vi "COD主界面（列队使用）.vi"() -> (8 "多列列表框":i32(listbox))   [LabVIEW 2016, in "斯坦道CODMn.lvlib"]
uses:
  <vilib>/Analysis/6fits.llb/Curve Fitting Criteria.ctl
  <vilib>/Utility/miscctls.llb/LVPointTypeDef.ctl
  <vilib>/Utility/config.llb/Read Key (I32).vi
  <vilib>/Utility/config.llb/Read Key (Double).vi
  <vilib>/Utility/config.llb/Read Key (Boolean).vi
  <vilib>/Utility/config.llb/Write Key (I32).vi
  <vilib>/Utility/config.llb/Read Key (String).vi
  <vilib>/Utility/config.llb/Write Key (Double).vi
  <vilib>/Utility/config.llb/Write Key (Boolean).vi
  <vilib>/Utility/config.llb/Write Key (String).vi
  <vilib>/Waveform/WDTFileIO.llb/Read Waveform from File.vi
  <vilib>/ptbypt/NI_PtbyPt.lvlib
  <vilib>/Utility/config.llb/NI_LVConfig.lvlib
  <vilib>/Analysis/NI_AALPro.lvlib
panel:
  in  "方程系数 2":cluster{"K":dbl, "b":dbl, "X^2":dbl} {"X^2" format="%#.6g"; "b" format="%#.6g"; "K" format="%#.6g"}
  out "r^2 2":dbl caption="r^2" format="%.8g"
  out "拟合公式 2":string
  in  "跨度值":dbl
  in  "公式切换阈值滴定数(0-9999)":u16
  out "公式系数":dbl[](array[numeric])
  in  "存校准信息":bool
  out "标液校准时间4":timestamp format="%<%Y/%m/%d %H:%M:%S>T"
  out "标液校准时间3":timestamp format="%<%Y/%m/%d %H:%M:%S>T"
  out "标液校准时间2":timestamp format="%<%Y/%m/%d %H:%M:%S>T"
  out "标液校准时间1":timestamp format="%<%Y/%m/%d %H:%M:%S>T"
  out "零点校准时间":timestamp format="%<%Y/%m/%d %H:%M:%S>T"
  in  "远程标样校准":enum16{"标液1", "标液2", "标液3", "标液4"}(ring)
  in  "远程校准量程":enum16{"低量程", "高量程"}(ring)
  in  "温度曲线":bool
  out "温度波形时间":timestamp
  in  "历史波形 2":bool
  out "时间-温度":u16[](array[numeric]) caption="数组"
  in  "关闭 4":bool
  out "时间温度曲线":u16[](graph)
  in  "加标回收量程：":enum32{"H", "L", "AUTO"}(ring)=enum."AUTO"
  in  "定时设置":cluster{"启动":bool, "控制命令":T1, "测量参数":T2}(xcontrol)
  out "氢氧化钠":dbl
  in  "序列号变更":bool
  out "模块版本号":string
  in  "更新程序":bool
  out "进样无液体告警":bool
  out "校准内容显示":string
  out "60分钟超时报警":bool
  in  "仪器参数":bool
  out "CODMn序列号":string
  out "CODMn软件版本：":string
  in  "标样核查量程选择":enum32{"H", "L", "AUTO"}(ring)=enum."AUTO"
  in  "标样浓度":dbl
  in  "零点核查量程选择":enum32{"H", "L", "AUTO"}(ring)=enum."AUTO"
  in  "零点核查浓度":dbl
  out "序列号":string
  in  "采水泵排液时间/s:":i32
  in  "采水泵润洗时间/s:":i32
  in  "采水泵沉淀时间/s:":i32
  in  "采水泵进样时间/s:":i32
  in  "常规版/认证版":enum16{"常规版-酸性", "常规版-碱性", "认证版", "浮台版"}(ring)
  in  "释放串口":bool
  in  "打开串口":bool
  in  "保存参数":dbl[](array[numeric])
  out "报警数字":i16
  out "CODMn工作状态":T3(ring)
  out "ORP-K":string
  out "ORP-B":string
  out "ORP-A":string
  out "x = y?":bool
  out "稀释倍数解释":string
  in  "跨度量程选择":enum32{"H", "L", "AUTO"}(ring)=enum."AUTO"
  in  "跨度液浓度":dbl
  in  "水样：":dbl
  in  "蒸馏水：":dbl
  in  "标液：":dbl
  in  "零点核查样：":dbl
  in  "加标回收样：":dbl
  in  "草酸钠":dbl
  in  "高锰酸钾":dbl
  in  "硫酸":dbl
  out "量程解释说明":string
  in  "高切低阈值:":dbl
  in  "低切高阈值:":dbl
  in  "水样量程选择:":enum16{"L", "H", "自动切换测一次", "自动切换测两次"}(ring)
  in  "氢氧化钠：":dbl
  in  "标准液浓度":dbl
  in  "温度":dbl
  in  "恒温时间":dbl
  in  "当前量程：":enum16{"L", "H"}(ring)
  in  "CODMn零点核查选择":enum16{"零点核查走纯水管", "零点核查走零漂管"}(ring)
  in  "锁定按钮":bool
  in  "低量程稀释倍数:":i8=1
  in  "高量程稀释倍数:":i8=2
  out "基本量程(显示)":string
  out "测量模式(显示)":string
  out "数据时间":string
  out "断电排液标记":bool
  out "COM":string
  in  "启用5":bool
  in  "校准5":bool
  in  "泵滴定数5":dbl
  in  "浓度5":dbl
  in  "启用4":bool
  in  "校准4":bool
  in  "泵滴定数4":dbl
  in  "浓度4":dbl
  out "波形时间":timestamp
  in  "历史波形":bool
  out "滴定数-ORP值":u16[](array[numeric]) caption="数组"
  in  "关闭 3":bool
  in  "滴定曲线":bool
  out "ORP滴定曲线":u16[](graph)
  out "空白测试标记":bool
  out "跨度核查标记":bool
  in  "量程选择":enum16{"低量程", "高量程"}(ring)
  in  "手动控制":bool
  in  "选用水样":enum16{"葡萄糖", "草酸钠"}(ring)
  in  "方程系数":cluster{"K":dbl, "b":dbl, "X^2":dbl} {"X^2" format="%#.6g"; "b" format="%#.6g"; "K" format="%#.6g"}
  out "XY图":cluster{"X Values":dbl[], "Y Values":dbl[]}[](graph)
  in  "模型":enum32{"线性", "多项式", "折线"}(ring)
  out "启动时间":timestamp format="%<%Y/%m/%d %H:%M:%S>T"
  in  "关闭 2":bool
  out "r^2":dbl format="%.8g"
  out "拟合公式":string
  in  "启用3":bool
  in  "启用2":bool
  in  "启用1":bool
  in  "校准3":bool
  in  "校准2":bool
  in  "校准1":bool
  in  "泵滴定数3":dbl
  in  "泵滴定数2":dbl
  in  "泵滴定数1":dbl
  in  "浓度3":dbl
  in  "浓度2":dbl
  in  "浓度1":dbl
  in  "写入":bool
  out "零点核查标记":bool
  out "排液故障":bool
  out "进水样超量程":bool
  out "标样核查标记":bool
  out "平行样测量":bool
  out "加标回收测量":bool
  out "质控样测量":bool
  out "待机":bool
  out "校标错误":bool
  out "校零错误":bool
  out "测量错误":bool
  out "草酸钠报警":bool
  out "高锰酸钾报警":bool
  out "加热故障":bool
  out "温控器故障":bool
  out "ORP故障":bool
  out "排液标记":bool
  out "故障标记":bool
  out "校标标记":bool
  out "校零标记":bool
  out "通讯状态":bool
  out "水样测量":bool
  in  "读取":bool
  in  "返回":bool
  in  "校准配置":bool
  in  "零点泵计量数 2":dbl
  in  "标度泵计量数 2":dbl
  out "标度滴定值":dbl
  out "零点滴定值":dbl
  in  "保存":bool
  in  "关闭":bool
  out "仪器时间":timestamp format="%<%Y/%m/%d %H:%M:%S>T"
  out "秒":u16
  out "分":u16
  out "COD浓度（mg/L)":dbl format="%.2g"
  out "进样管":dbl
  out "高锰酸钾":dbl
  out "草酸钠":dbl
  out "硫酸":dbl
  out "实时ORP":dbl
  out "温度℃":dbl
  out "加热":bool
  out "搅拌":bool
  out "进硫酸":bool
  out "进加标回收样":bool
  out "进零点核查样":bool
  out "进标液":bool
  out "进蒸馏水":bool
  out "进水样":bool
  out "进草酸钠":bool
  out "进高锰酸钾":bool
  in  "启动":bool
  in  "故障清除":bool
  in  "参数配置":bool
  in  "停止":bool
  in  "单步启动":bool
  out "系统时间":timestamp
  in  "时间校准":bool
  out "模式（受控）":u16
  # "测试时长："
  # "注：遇到加热故障和排液故障时仪器不能正常启动，\n必须排查故障并点击报警清除按钮方可运行。"
  # "mg/L"
  # "基本参数设置"
  # "校零校标结果"
  # "泵计量参数设置"
  # "校零结果："
  # "校零滴定值："
  # "高锰酸钾："
  # "加热恒温温度(℃):"
  # "草酸钠："
  # "校标结果："
  # "标度滴定值："
  # "恒温时间(分钟):"
  # "零点泵计量值："
  # "硫酸："
  # "标准液浓度(mg/L):"
  # "标度泵计量值："
  # "跨度核查浓度："
  # "跨度核查量程："
  # "零点核查浓度："
  # "标样浓度："
  # "零点核查量程："
  # "标样核查量程："
  # "跨度值:"
  # "校准配置界面"
  # "测量信号值"
  # "启用"
  # "校准时间"
  # "浓度"
  # "零点"
  # "标液1"
  # "标液2"
  # "标液3"
  # "标液4"
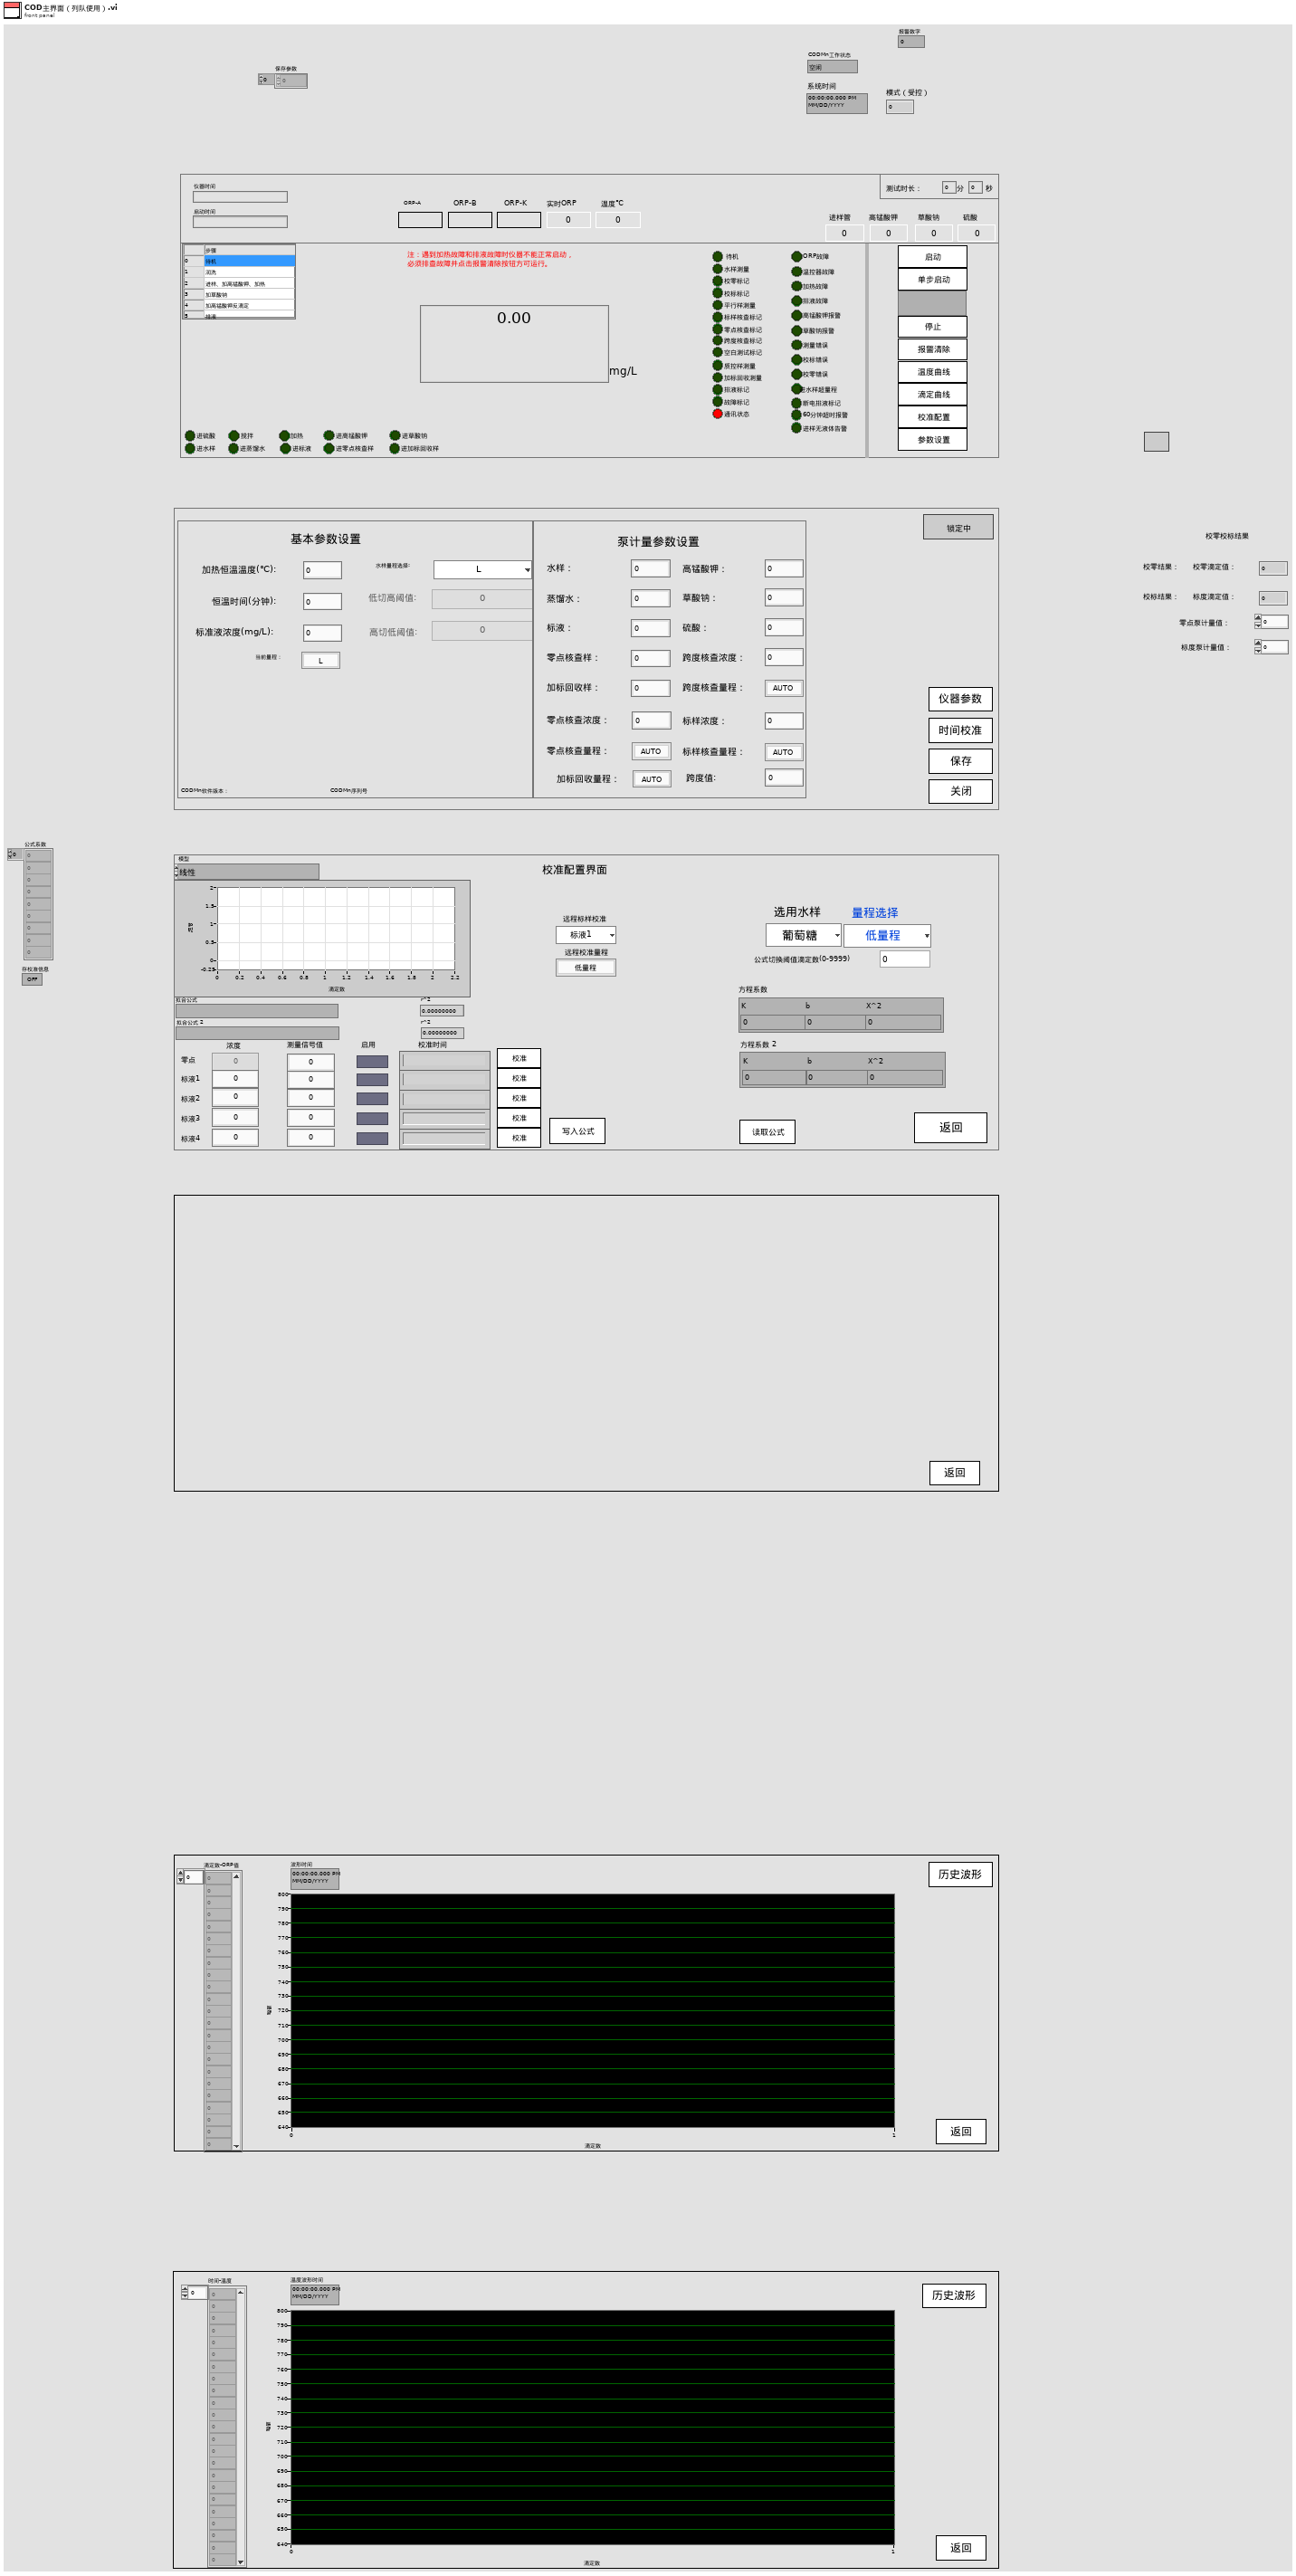
[diagram p1: front panel]
types:
  T1 = typedef "定时设置.xctl/国标控制命令.ctl" = enum16{"启动测量", "标样核查", "零点核查", "跨度核查", "空白测试", "平行样测试", "加标回收", "空白校准", "标样校准", "初始化（清洗）", "停止测试", "仪器重启", "校时", "模式设置", "测量间隔设置"}
  T2 = typedef "定时设置.xctl/测量参数.ctl" = u16
  T3 = enum16{"空闲", "水样测试", "标样核查", "零点核查", "跨度核查", "空白测试", "平行样测试", "质控样", "空白校准", "标样校准", "加标回收"}
  T4 = typedef "LVPointTypeDef.ctl" = cluster{"Horizontal":i16, "Vertical":i16}
  T5 = cluster{"Major":u16, "Minor":u16, "Fix":u16, "Build":u16}
  T6 = typedef "NI_LVConfig.lvlib/Config Data RefNum.ctl" = refnum<k1>
  T7 = cluster{"时间源选择":enum16{"系统时间源", "仪器时间源"}, "外部时间源":timestamp}
  T8 = enum32{"Bad", "Idle", "Run top level", "Running"}
  T9 = enum8{"Enabled", "Disabled", "Disabled and Grayed Out"}
  T10 = cluster{"时间":timestamp, "测量模式":string, "数据类型":string, "检测值":sgl, "单位":string, "数据标识":string, "因子编码":string, "标样参考值":sgl, "ORP-A":sgl, "ORP-B":sgl, "ORP-K":sgl, "COD滴定值":sgl, "高锰酸钾滴定数":sgl, "温度":sgl, "量程":sgl, "LastTime":timestamp, "序列号:":string, "跨度值":sgl}
  T11 = cluster{"因子编码":u32, "单位":u16, "标样参考值":sgl, "水样数据时间":timestamp, "水样实测值":sgl, "水样数据标识":string, "标样数据时间":timestamp, "标样实测值":sgl, "标样数据标识":string, "空白数据时间":timestamp, "空白实测值":sgl, "空白数据标识":string, "零点核查数据时间":timestamp, "零点核查实测值":sgl, "零点核查数据标识":string, "跨度核查数据时间":timestamp, "跨度核查实测值":sgl, "跨度核查数据标识":string, "加标回收数据时间":timestamp, "加标回收实测值":sgl, "加标回收数据标识":string, "平行样数据时间":timestamp, "平行样实测值":sgl, "平行样数据标识":string}
  T12 = cluster{"测量量程":dbl, "测量精度":dbl, "测量间隔":dbl, "消解温度":dbl, "消解时长":dbl, "空白校准时间":timestamp, "曲线截距":dbl, "曲线斜率":dbl, "测量检出限":dbl, "测量信号值":dbl, "线性相关系数":dbl, "二次多项式系数":dbl, "标样校准时间":timestamp, "稀释倍数":dbl, "三项式系数":dbl, "空白标定系数":dbl, "量程系数":dbl, "F0/ORPA":dbl, "F1/ORPB":dbl, "F2/ORPK":dbl, "F3":dbl, "F4":dbl, "F5":dbl, "F6":dbl, "F7":dbl, "X0/滴定数":dbl, "量程":dbl}
  T13 = cluster{"运行模式":enum16{"维护模式", "常规模式", "应急模式", "质控模式"}, "质控频次":enum16{"关闭", "每天", "星期一", "星期二", "星期三", "星期四", "星期五", "星期六", "星期日"}, "空白核查时间":u16, "跨度核查时间":u16, "24H周期设置":bool[]}
  T14 = cluster{"数组 2[0]":sgl, "数组 2[1]":sgl, "数组 2[2]":sgl, "数组 2[3]":sgl, "数组 2[4]":sgl, "数组 2[5]":sgl, "数组 2[6]":sgl, "数组 2[7]":sgl, "数组 2[8]":sgl, "数组 2[9]":sgl, "数组 2[10]":sgl, "数组 2[11]":sgl, "数组 2[12]":sgl, "数组 2[13]":sgl, "数组 2[14]":sgl, "数组 2[15]":sgl, "数组 2[16]":sgl, "数组 2[17]":sgl, "数组 2[18]":sgl, "数组 2[19]":sgl, "数组 2[20]":sgl, "数组 2[21]":sgl, "数组 2[22]":sgl, "数组 2[23]":sgl, "数组 2[24]":sgl, "数组 2[25]":sgl, "数组 2[26]":sgl, "数组 2[27]":sgl, "数组 2[28]":sgl, "数组 2[29]":sgl, "数组 2[30]":sgl, "数组 2[31]":sgl, "数组 2[32]":sgl, "数组 2[33]":sgl, "数组 2[34]":sgl, "数组 2[35]":sgl, "数组 2[36]":sgl, "数组 2[37]":sgl, "数组 2[38]":sgl, "数组 2[39]":sgl, "数组 2[40]":sgl, "数组 2[41]":sgl}
  T15 = typedef "NI_AALPro.lvlib/Curve Fitting Criteria.ctl" = u16
  T16 = cluster{"ORP故障":bool, "温控器故障":bool, "加热故障":bool, "高锰酸钾报警":bool, "草酸钠报警":bool, "测量错误":bool, "校零错误":bool, "校标错误":bool, " 进水样超量程":bool, "排液阀故障":bool, "60分钟超时报警":bool, "进样无液体报警":bool}
  T17 = cluster{"时间标识":timestamp, "参数":string, "日志信息":string, "流程参数":string}
  T18 = cluster{"确定":bool, "测量量程":dbl, "测量精度":dbl, "测量间隔":dbl, "消解温度":dbl, "消解时长":dbl, "空白校准时间":timestamp, "曲线截距":dbl, "曲线斜率":dbl, "测量检出限":dbl, "测量信号值":dbl, "线性相关系数":dbl, "二次多项式系数":dbl, "标样校准时间":timestamp, "稀释倍数":dbl, "三项式系数":dbl, "空白标定系数":dbl, "量程系数":dbl, "F0/ORPA":dbl, "F1/ORPB":dbl, "F2/ORPK":dbl, "F3":dbl, "F4":dbl, "F5":dbl, "F6":dbl, "F7":dbl, "X0/滴定数":dbl, "量程":dbl}
  T19 = cluster{"时间标识":timestamp, "设备":string, "日志信息":string, "流程参数":string}
  T20 = cluster{"[0]":string, "[1]":string, "[2]":string}
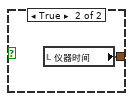
[diagram p3: hidden frame]
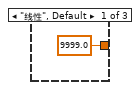
[diagram p9: hidden frame]
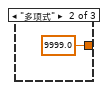
[diagram p10: hidden frame]
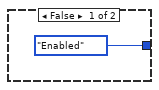
[diagram p11: hidden frame]
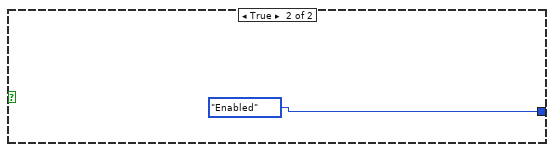
[diagram p12: hidden frame]
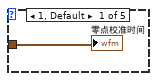
[diagram p17: hidden frame]
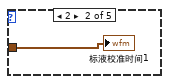
[diagram p18: hidden frame]
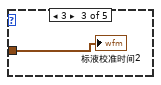
[diagram p19: hidden frame]
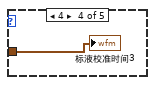
[diagram p20: hidden frame]
diagram:
  n1 = flat-sequence {
    tunnel: w3 -> [_]
    frame #0 {
      n2 = vi-ref "斯坦道CODMn.lvlib:待机状态数据存储写入和切换量程(子VI).vi"() -> (w64:refnum<vi>)
      n3 = vi-ref "斯坦道CODMn.lvlib:日志报警状态存储 (子VI).vi"() -> (w57:refnum<vi>)
      n4 = vi-ref "斯坦道CODMn.lvlib:高锰酸钾-ORP滴定曲线(子VI).vi"() -> (w44:refnum<vi>)
      n5 = property class="VI"(reference=w57, error in=errorcluster {"status"=FALSE, "code"=0, "source"=""} ("错误输出")) -> ("Name"=w56:string)  [unwired: 2 out]
      n6 = property class="VI"(reference=w44, error in=errorcluster {"status"=FALSE, "code"=0, "source"=""} ("错误输出")) -> ("Name"=w45:string)  [unwired: 2 out]
      n7 = property class="VI"(reference=w64, error in=errorcluster {"status"=FALSE, "code"=0, "source"=""} ("错误输出")) -> ("Name"=w63:string)  [unwired: 2 out]
      n8 = Open VI Reference(type specifier VI Refnum (for type only)=refnum<vi> refnum, vi path=w56, options=128 ("选项")) -> (vi reference=w40:refnum<vi>, error out=w54:errorcluster)  [unwired: 3 in]
      n9 = Open VI Reference(type specifier VI Refnum (for type only)=refnum<vi> refnum, vi path=w45, options=128 ("选项")) -> (vi reference=w43:refnum<vi>, error out=w47:errorcluster)  [unwired: 3 in]
      n10 = call-by-ref "?"(reference=w40, error in=w54) -> (reference out=w52:refnum<vi>, error out=w53:errorcluster)  [unwired: 12 in]
      n11 = call-by-ref "?"(reference=w43, error in=w47) -> (reference out=w49:refnum<vi>, error out=w48:errorcluster)  [unwired: 12 in]
      n12 = Open VI Reference(type specifier VI Refnum (for type only)=refnum<vi> refnum, vi path=w63, options=128 ("选项")) -> (vi reference=w38:refnum<vi>, error out=w61:errorcluster)  [unwired: 3 in]
      n13 = Close Reference(reference=w52, error in (no error)=w53) -> ()  [unwired: 1 out]
      n14 = call-by-ref "?"(reference=w38, error in=w61) -> (reference out=w59:refnum<vi>, error out=w60:errorcluster)  [unwired: 12 in]
      n15 = Close Reference(reference=w49, error in (no error)=w48) -> ()  [unwired: 1 out]
      n16 = Close Reference(reference=w59, error in (no error)=w60) -> ()  [unwired: 1 out]
      n17 = vi-ref "斯坦道CODMn.lvlib:时间-温度曲线(子VI).vi"() -> (w26:refnum<vi>)
      n18 = vi-ref "斯坦道CODMn.lvlib:关键参数交互.vi"() -> (w35:refnum<vi>)
      n19 = property class="VI"(reference=w35, error in=errorcluster {"status"=FALSE, "code"=0, "source"=""} ("错误输出")) -> ("Name"=w34:string)  [unwired: 2 out]
      n20 = property class="VI"(reference=w26, error in=errorcluster {"status"=FALSE, "code"=0, "source"=""} ("错误输出")) -> ("Name"=w25:string)  [unwired: 2 out]
      n21 = Open VI Reference(type specifier VI Refnum (for type only)=refnum<vi> refnum, vi path=w34, options=128 ("选项")) -> (vi reference=w36:refnum<vi>, error out=w32:errorcluster)  [unwired: 3 in]
      n22 = call-by-ref "?"(reference=w36, error in=w32, "量程选择"=enum16{"低量程", "高量程"}."低量程", "模型"=enum32{"线性", "多项式", "折线"}."线性") -> (reference out=w30:refnum<vi>, error out=w31:errorcluster)  [unwired: 10 in]
      n23 = Open VI Reference(type specifier VI Refnum (for type only)=refnum<vi> refnum, vi path=w25, options=128 ("选项")) -> (vi reference=w27:refnum<vi>, error out=w23:errorcluster)  [unwired: 3 in]
      n24 = call-by-ref "?"(reference=w27, error in=w23) -> (reference out=w21:refnum<vi>, error out=w22:errorcluster)  [unwired: 12 in]
      n25 = Close Reference(reference=w30, error in (no error)=w31) -> ()  [unwired: 1 out]
      n26 = Close Reference(reference=w21, error in (no error)=w22) -> ()  [unwired: 1 out]
    }
  }
  n27 = property on="定时设置" class="定时设置 (严格)"("引用参数"="CODMn") -> (error out=w1:errorcluster)  [unwired: 2 in, 1 out]
  n28 = flat-sequence {
    tunnel: [w68] -> w5
    tunnel: [errorcluster {"status"=FALSE, "code"=0, "source"=""} ("错误输出")] -> w3
    tunnel: [w70] -> w4
    frame #0 {
      w92 = "192.168.1.100" ("名称")
      n29 = global write "COD内部交互全局.vi" "量程切换次数"(u8 0 ("量程切换次数")) -> ()
      n30 = global write "COD内部交互全局.vi" "切换量程连续测两次"(FALSE ("切换量程连续测两次")) -> ()
      n31 = global read "COD内部交互全局.vi" "序列号:"() -> (w99:string)
      n32 = property on="窗格" class="Pane"("Origin"=T4 {"Horizontal"=0, "Vertical"=0} ("原点")) -> ()  [unwired: 2 in, 2 out]
      n33 = Empty String/Path?(string/path=w99) -> (empty?=w67:bool)
      n34 = case shown="真" w67 {
        tunnel: w99 -> [w113 _]
        tunnel: [w112 "data\\CODMnSet.ini" ("名称或相对路径")] -> w80
        frame False {
          # "与生产用上位机交互"
          n35 = Concatenate Strings("data\\" ("字符串"), "序列号" ("字符串"), w113, "Set.ini" ("名称或相对路径")) -> (w112:string)
        }
        frame True {
        }
      }
      n36 = String To IP(1:w92) -> (0:w85:u32)
      n37 = IP To String(2:w85) -> (0:w88:string)  [unwired: 1 in]
      n38 = Not Equal?(x=w92, y=w88) -> (x != y?=w93:bool)
      n39 = Concatenate Strings("\\\\" ("字符串"), w88) -> (w87:string)
      n40 = global write "CODMN外部API.vi" "ping"(w93) -> ()
      n41 = String To Path(string=w87) -> (path=w94:path)
      n42 = Build Path(base path=w94, name or relative path=w80) -> (appended path=w89:path)
      n43 = local write "量程选择"(enum16{"低量程", "高量程"}."低量程" ("量程选择")) -> ()
      n44 = local write "选用水样"(enum16{"葡萄糖", "草酸钠"}."葡萄糖" ("选用水样")) -> ()
      n45 = global write "COD内部交互全局.vi" "配置文件ini"(w80) -> ()
      n46 = case shown="真" w93 {
        tunnel: w89 -> [w103 w107]
        tunnel: [w103 w106] -> w90
        tunnel: [FALSE w105] -> w91
        frame False {
        }
        frame True {
          n47 = call <vilib>:"Check if File or Folder Exists.vi"("path"=w107) -> ("file or folder exists?"=w105:bool, "dup path"=w106:path)  [unwired: 8 in, 1 out]
        }
      }
      n48 = control-ref of="本VI"() -> (w79:refnum<vi>)
      n49 = case shown="假" w91 {
        tunnel: w90 -> [_ w111]
        tunnel: [w109 w111] -> w71
        tunnel: w80 -> [w108 _]
        frame False {
          # "本地文件地址"
          n50 = call <vilib>:"Application Directory.vi"() -> ("Application Directory"=w110:path)
          n51 = Build Path(base path=w110, name or relative path=w108) -> (appended path=w109:path)
        }
        frame True {
          # "网络共享地址"
        }
      }
      n52 = property class="VI"(reference=w79) -> ("Library.Version"=w78:T5)  [unwired: 1 in, 2 out]
      n53 = Unbundle By Name(w78) -> ("Major"=w76:u16, "Minor"=w75:u16, "Fix"=w74:u16, "Build"=w73:u16)
      n54 = Format Into String(format string="模块版本号：%d.%d.%d.%d" ("格式字符串"), w76, w75, w74, w73) -> (resulting string=→"模块版本号":string)  [unwired: 2 in, 1 out]
      n55 = global write "CODMN外部API.vi" "配置文件 path"(w71) -> ()
      n56 = call <vilib>:"Open Config Data.vi"("configuration file path"=w71) -> ("error out"=w81:errorcluster, "refnum"=w82:T6)  [unwired: 8 in, 1 out]
      n57 = vi-ref "斯坦道CODMn.lvlib:CODMn断电保存全局变量.vi"() -> (w95:refnum<vi>)
      n58 = call <userlib>:"Read Panel from INI__ogtk.vi"("error in (no error)"=w81, "VI ref"=w95, "refnum"=w82) -> ("error out"=w83:errorcluster, "refnum out"=w84:T6)  [unwired: 7 in]
      n59 = call <vilib>:"Close Config Data.vi"("error in (no error)"=w83, "refnum"=w84) -> ("error out"=w69:errorcluster)  [unwired: 8 in, 1 out]
      n60 = call <vilib>:"Clear Errors.vi"("error in (no error)"=w69) -> ("error out"=w66:errorcluster)  [unwired: 5 in, 1 out]
      n61 = Read from Text File(file (use dialog)=w71, error in=w66) -> (text=w70:string, error out=w68:errorcluster)  [unwired: 2 in, 2 out]
      "稀释倍数解释" <- "稀释倍数解释：\n稀释倍数选择1，表示不稀释\n默认低量程系数倍数1，高量程系数倍数2\n则低量程为0~8，高量程为0~16" ("稀释倍数解释")
    }
  }
  n62 = while {
    tunnel: w1 -> [_]
    stop <- FALSE stop-if-true
    n63 = Wait (ms)(milliseconds to wait=u32 500 ("等待时间（毫秒）")) -> ()  [unwired: 1 out]
    n64 = global read "COD测量模式全局.vi" "CODMn工作状态"() -> (w124:T3)
    n65 = local read "通讯状态"() -> (w118:bool)
    n66 = case shown="假" w118 {
      tunnel: [w134 w135] -> w122
      frame False {
        n67 = Get Date/Time In Seconds() -> (seconds since 1Jan1904=w134:timestamp)
      }
      frame True {
        n68 = local read "仪器时间"() -> (w135:timestamp)
      }
    }
    n69 = vi-ref "斯坦道CODMn.lvlib:CODMn测量流程.vi"() -> (w131:refnum<vi>)
    n70 = Bundle By Name(cluster=T7 {"时间源选择"=enum."系统时间源", "外部时间源"=timestamp(0 s since 1904-01-01)} ("时间源"), "时间源选择"=enum16{"系统时间源", "仪器时间源"}."仪器时间源", "外部时间源"=w122) -> (w120:T7)
    n71 = property class="VI"(reference=w131) -> ("Exec.State"=w129:T8, "Name"=w130:string)  [unwired: 1 in, 2 out]
    n72 = Not Equal?(x=w124, y=T3."空闲") -> (x != y?=w119:bool)
    n73 = property on="定时设置" class="定时设置 (严格)"("仪器状态"=w119, "时间源"=w120) -> ()  [unwired: 2 in, 2 out]
    n74 = Unbundle By Name("定时设置") -> ("启动"=w127:bool, "控制命令"=w128:T1)
    n75 = case shown="真" w127 {
      tunnel: w130 -> [_ w138]
      tunnel: w128 -> [_ w137]
      tunnel: w129 -> [_ w136]
      frame False {
      }
      frame True {
        n76 = case shown="\"Idle\"" w136 {
          tunnel: w138 -> [_ w142]
          tunnel: w137 -> [_ w139]
          frame "Bad", Default {
          }
          frame "Idle" {
            n77 = Open VI Reference(type specifier VI Refnum (for type only)=refnum<vi> refnum, vi path=w142, options=128 ("选项")) -> (vi reference=w143:refnum<vi>, error out=w144:errorcluster)  [unwired: 3 in]
            n78 = call-by-ref "开始异步调用"(reference=w143, error in=w144, "控制命令"=w139) -> (reference out=w145:refnum<vi>, error out=w146:errorcluster)  [unwired: 11 in]
            n79 = Close Reference(reference=w145, error in (no error)=w146) -> ()  [unwired: 1 out]
          }
        }
      }
    }
  }
  n80 = Obtain Queue(name (unnamed)="CODMn" ("名称（未命名）"), element data type=cluster{"命令":string} {"命令"="启用模块"} ("元素")) -> (queue out=w15:refnum<queue>, error out=w14:errorcluster)  [unwired: 3 in, 1 out]
  n81 = while {
    tunnel: [w153] -> _
    shift-right: [w151] -> _
    shift-left: w4 -> [w150]
    tunnel: w5 -> [_]
    stop <- FALSE stop-if-true
    n82 = global read "CODMN外部API.vi" "配置文件 path"() -> (w147:path)
    n83 = Wait (ms)(milliseconds to wait=u32 1000 ("等待时间（毫秒）")) -> ()  [unwired: 1 out]
    n84 = Read from Text File(file (use dialog)=w147) -> (text=w151:string, error out=w148:errorcluster)  [unwired: 3 in, 2 out]
    n85 = Not Equal?(x=w151, y=w150) -> (x != y?=w149:bool)
    n86 = case shown="真" w149 {
      tunnel: [w155 w162] -> w153
      tunnel: w147 -> [_ w156]
      tunnel: w148 -> [w155 _]
      frame False {
      }
      frame True {
        # "文件发生改变进行更新，远端和本地都更新"
        n87 = vi-ref "斯坦道CODMn.lvlib:CODMn断电保存全局变量.vi"() -> (w157:refnum<vi>)
        n88 = call <vilib>:"Open Config Data.vi"("configuration file path"=w156) -> ("error out"=w161:errorcluster, "refnum"=w160:T6)  [unwired: 8 in, 1 out]
        n89 = call <userlib>:"Read Panel from INI__ogtk.vi"("error in (no error)"=w161, "VI ref"=w157, "refnum"=w160) -> ("error out"=w159:errorcluster, "refnum out"=w158:T6)  [unwired: 7 in]
        n90 = call <vilib>:"Close Config Data.vi"("error in (no error)"=w159, "refnum"=w158) -> ("error out"=w162:errorcluster)  [unwired: 8 in, 1 out]
      }
    }
  }
  n91 = vi-ref "CODMn通讯.vi"() -> (w6:refnum<vi>)
  n92 = while {
    stop <- FALSE stop-if-true
    n93 = global read "COD内部交互全局.vi" "待机"() -> (w164:bool)
    n94 = Wait (ms)(milliseconds to wait=u32 1000 ("等待时间（毫秒）")) -> ()  [unwired: 1 out]
    n95 = case shown="假" w164 {
      tunnel: [w181 T9."Enabled" ("禁用")] -> w166
      tunnel: [w180 _] -> w165
      frame False {
        # "运行中"
        n96 = local read "校标标记"() -> (w179:bool)
        n97 = local read "校零标记"() -> (w178:bool)
        n98 = Or(x=w179, y=w178) -> (x .or. y?=w182:bool)
        n99 = case shown="真" w182 {
          tunnel: [T9."Enabled" ("禁用") T9."Disabled and Grayed Out" ("禁用")] -> w181
          tunnel: [_ TRUE] -> w180
          frame False {
          }
          frame True {
          }
        }
      }
      frame True {
      }
    }
    n100 = control-ref of="量程选择"() -> (w172:refnum<vi>)
    n101 = property on="校准内容显示" class="Str"("Visible"=w165) -> ()  [unwired: 2 in, 2 out]
    n102 = control-ref of="选用水样"() -> (w173:refnum<vi>)
    n103 = control-ref of="校准5"() -> (w167:refnum<vi>)
    n104 = control-ref of="校准4"() -> (w168:refnum<vi>)
    n105 = control-ref of="校准3"() -> (w169:refnum<vi>)
    n106 = control-ref of="校准2"() -> (w170:refnum<vi>)
    n107 = control-ref of="校准1"() -> (w171:refnum<vi>)
    n108 = Build Array(w167, w168, w169, w170, w171, w173, w172) -> (w174:refnum<vi>[])
    n109 = for {
      tunnel: w174 -> [w177] mode=indexing
      tunnel: w166 -> [w176]
      n110 = property class="Ctl"(reference=w177, "DisabledEnum"=w176) -> ()  [unwired: 1 in, 2 out]
    }
  }
  n111 = while {
    tunnel: w5 -> [_]
    stop <- FALSE stop-if-true
    # "赋值循环"
    n112 = flat-sequence {
      frame #0 {
        # "测量数据区"
        n113 = global read "COD内部交互全局.vi" "data"() -> (w326:T10)
        n114 = global read "COD测量模式全局.vi" "测量模式文字实时"() -> (w312:string)
        "测量模式(显示)" <- w312
        n115 = global read "CODMn断电保存全局变量.vi" "测量数据区"() -> (w321:T11)
        n116 = Unbundle By Name(w326) -> ("时间"=w325:timestamp, "检测值"=w324:sgl, "数据标识"=w323:string)
        n117 = case shown="\"水样测试\"" w312 {
          tunnel: w321 -> [w327 w332 w337 w342 w347 w352 w357 w362 w367 w372]
          tunnel: [w327 w331 w336 w338 w346 w351 w356 w361 w363 w371] -> w322
          tunnel: w325 -> [_ w330 w335 w341 w345 w350 w355 w360 w366 w370]
          tunnel: w324 -> [_ w329 w334 w340 w344 w349 w354 w359 w365 w369]
          tunnel: w323 -> [_ w328 w333 w339 w343 w348 w353 w358 w364 w368]
          frame "", Default {
          }
          frame "水样测试" {
            n118 = Bundle By Name(cluster=w332, "水样数据时间"=w330, "水样实测值"=w329, "水样数据标识"=w328) -> (w331:T11)
          }
          frame "标样核查" {
            n119 = Bundle By Name(cluster=w337, "标样数据时间"=w335, "标样实测值"=w334, "标样数据标识"=w333) -> (w336:T11)
          }
          frame "跨度核查" {
            n120 = Bundle By Name(cluster=w342, "跨度核查数据时间"=w341, "跨度核查实测值"=w340, "跨度核查数据标识"=w339) -> (w338:T11)
          }
          frame "零点核查" {
            n121 = Bundle By Name(cluster=w347, "零点核查数据时间"=w345, "零点核查实测值"=w344, "零点核查数据标识"=w343) -> (w346:T11)
          }
          frame "空白测试" {
            n122 = Bundle By Name(cluster=w352, "空白数据时间"=w350, "空白实测值"=w349, "空白数据标识"=w348) -> (w351:T11)
          }
          frame "加标回收" {
            n123 = Bundle By Name(cluster=w357, "加标回收数据时间"=w355, "加标回收实测值"=w354, "加标回收数据标识"=w353) -> (w356:T11)
          }
          frame "平行样" {
            n124 = Bundle By Name(cluster=w362, "平行样数据时间"=w360, "平行样实测值"=w359, "平行样数据标识"=w358) -> (w361:T11)
          }
          frame "校零" {
            n125 = Bundle By Name(cluster=w367, "空白数据时间"=w366, "空白实测值"=w365, "空白数据标识"=w364) -> (w363:T11)
          }
          frame "校标" {
            n126 = Bundle By Name(cluster=w372, "标样数据时间"=w370, "标样实测值"=w369, "标样数据标识"=w368) -> (w371:T11)
          }
        }
        n127 = Unbundle By Name(w321) -> ("水样实测值"=w318:sgl)
        n128 = feedback-in #1(w321) -> ()
        n129 = feedback #1(w321) -> (w320:T11)
        n130 = global read "CODMn断电保存全局变量.vi" "水样测试量程"() -> (w314:enum16{"L", "H"})
        n131 = Unbundle By Name(w320) -> ("水样实测值"=w319:sgl)
        n132 = feedback #2(w314) -> (w315:enum16{"L", "H"})
        n133 = feedback-in #2(w314) -> ()
        n134 = Not Equal?(x=w315, y=w314) -> (x != y?=w313:bool)
        n135 = Not Equal?(x=w318, y=w319) -> (x != y?=w317:bool)
        n136 = global write "CODMn断电保存全局变量.vi" "测量数据区"(w322) -> ()
        n137 = Or(x=w317, y=w313) -> (x .or. y?=w316:bool)
        n138 = case shown="真" w316 {
          frame False {
          }
          frame True {
            # "水样值发送改变存储本地"
            n139 = call "配置文件保存.vi"() -> ()  [unwired: 12 in]
          }
        }
      }
    }
    n140 = flat-sequence {
      frame #0 {
        # "局部变量给内部交互用全局变量"
        n141 = local read "COD浓度（mg/L)"() -> (w219:dbl)
        n142 = local read "CODMn工作状态"() -> (w222:T3)
        n143 = local read "多列列表框"() -> (w220:i32)
        n144 = local read "标准液浓度"() -> (w218:dbl)
        n145 = local read "温度℃"() -> (w213:dbl)
        n146 = local read "高锰酸钾报警"() -> (w216:bool)
        n147 = local read "断电排液标记"() -> (w215:bool)
        n148 = local read "实时ORP"() -> (w212:dbl)
        n149 = local read "故障标记"() -> (w221:bool)
        n150 = local read "高锰酸钾"() -> (w214:dbl)
        n151 = local read "待机"() -> (w217:bool)
        n152 = global write "COD内部交互全局.vi" "实时温度"(w213) -> ()
        n153 = global write "运行时序全局变量.vi" "多列列表框"(w220) -> ()
        n154 = global write "COD内部交互全局.vi" "故障标记"(w221) -> ()
        n155 = global write "COD内部交互全局.vi" "ORP显示"(w212) -> ()
        n156 = global write "COD浓度全局变量.vi" "标准液浓度"(w218) -> ()
        n157 = global write "COD内部交互全局.vi" "高锰酸钾"(w214) -> ()
        n158 = global write "COD内部交互全局.vi" "待机"(w217) -> ()
        n159 = global write "COD测量模式全局.vi" "CODMn工作状态"(w222) -> ()
        n160 = global write "COD内部交互全局.vi" "高锰酸钾报警"(w216) -> ()
        n161 = global write "COD内部交互全局.vi" "断电排液标记"(w215) -> ()
        n162 = global write "COD浓度全局变量.vi" "COD浓度（mg/L)"(w219) -> ()
      }
    }
    n163 = flat-sequence {
      frame #0 {
        # "断电保存全局给局部变量"
        n164 = global read "CODMn断电保存全局变量.vi" "高切低阈值:"() -> (w392:dbl)
        n165 = global read "CODMn断电保存全局变量.vi" "低切高阈值:"() -> (w391:dbl)
        n166 = global read "CODMn断电保存全局变量.vi" "跨度液浓度"() -> (w389:dbl)
        n167 = global read "COD内部交互全局.vi" "波形时间"() -> (→"波形时间":timestamp)
        n168 = global read "CODMn断电保存全局变量.vi" "启动时间"() -> (→"启动时间":timestamp)
        n169 = global read "CODMn断电保存全局变量.vi" "标样浓度"() -> (w387:dbl)
        n170 = global read "CODMn断电保存全局变量.vi" "CODMn跨度量程选择"() -> (w393:enum32{"H", "L", "AUTO"})
        n171 = global read "CODMn断电保存全局变量.vi" "标样核查量程选择"() -> (w384:enum32{"H", "L", "AUTO"})
        n172 = global read "CODMn断电保存全局变量.vi" "零点核查量程选择"() -> (w386:enum32{"H", "L", "AUTO"})
        n173 = global read "CODMn断电保存全局变量.vi" "加标回收量程选择"() -> (w379:enum32{"H", "L", "AUTO"})
        n174 = global read "COD内部交互全局.vi" "滴定数-ORP值"() -> (→"滴定数-ORP值":u16[])
        n175 = global read "CODMn断电保存全局变量.vi" "常规版/认证版"() -> (w388:enum16{"常规版-酸性", "常规版-碱性", "认证版", "浮台版"})
        n176 = global read "CODMn断电保存全局变量.vi" "自动切换量程:"() -> (w390:enum16{"L", "H", "自动切换测一次", "自动切换测两次"})
        n177 = global read "CODMn断电保存全局变量.vi" "零点核查浓度"() -> (w385:dbl)
        n178 = local write "高切低阈值:"(w392) -> ()
        n179 = global read "CODMn断电保存全局变量.vi" "跨度值"() -> (w373:dbl)
        n180 = local write "跨度液浓度"(w389) -> ()
        n181 = local write "低切高阈值:"(w391) -> ()
        n182 = global read "COD内部交互全局.vi" "ORP滴定曲线"() -> (→"ORP滴定曲线":u16[])
        n183 = local write "标样浓度"(w387) -> ()
        n184 = local write "标样核查量程选择"(w384) -> ()
        n185 = local write "水样量程选择:"(w390) -> ()
        n186 = local write "常规版/认证版"(w388) -> ()
        n187 = local write "零点核查浓度"(w385) -> ()
        n188 = local write "零点核查量程选择"(w386) -> ()
        n189 = local write "加标回收量程："(w379) -> ()
        n190 = local write "跨度量程选择"(w393) -> ()
        n191 = local write "跨度值"(w373) -> ()
        n192 = global read "CODMn断电保存全局变量.vi" "远程校准量程"() -> (w374:enum16{"低量程", "高量程"})
        n193 = global read "CODMn断电保存全局变量.vi" "远程标样校准"() -> (w375:enum16{"标液1", "标液2", "标液3", "标液4"})
        n194 = global read "COD内部交互全局.vi" "温度波形时间"() -> (→"温度波形时间":timestamp)
        n195 = global read "COD内部交互全局.vi" "时间温度曲线"() -> (→"时间温度曲线":u16[])
        n196 = global read "COD内部交互全局.vi" "时间-温度"() -> (→"时间-温度":u16[])
        n197 = local write "远程标样校准"(w375) -> ()
        n198 = local write "远程校准量程"(w374) -> ()
      }
    }
    n199 = flat-sequence {
      frame #0 {
        # "保存参数赋值"
        n200 = Multiply(x="温度", y=10.0) -> (x*y=w197:dbl)
        n201 = Multiply(x="标准液浓度", y=100.0) -> (x*y=w194:dbl)
        n202 = Build Array(w197, "恒温时间", w194, "氢氧化钠：", "当前量程：", "水样：", "蒸馏水：", "标液：", "零点核查样：", "加标回收样：", "高锰酸钾", "草酸钠", "硫酸", "零点泵计量数 2", "标度泵计量数 2", "高量程稀释倍数:", "低量程稀释倍数:", "CODMn零点核查选择") -> (w191:dbl[])
        n203 = local write "保存参数"(w191) -> ()
      }
    }
    n204 = flat-sequence {
      frame #0 {
        # "显示量程说明"
        n205 = global read "COD内部交互全局.vi" "通讯状态"() -> (→"通讯状态":bool)
        n206 = global read "CODMn断电保存全局变量.vi" "MB通信方式选择"() -> (w397:enum16{"串口", "TCP"})
        n207 = local read "低量程稀释倍数:"() -> (w410:i8)
        n208 = local read "高量程稀释倍数:"() -> (w400:i8)
        n209 = case shown="\"TCP\"" w397 {
          tunnel: [w413 w414] -> w401
          frame "串口", Default {
            n210 = global read "CODMn断电保存全局变量.vi" "VISA resource name"() -> (w413:refnum<visa-resource-name>)
          }
          frame "TCP" {
            n211 = global read "CODMn断电保存全局变量.vi" "IP"() -> (w414:string)
          }
        }
        "COM" <- w401
        n212 = Multiply(x=w410, y=i8 8) -> (x*y=w402:i8)
        n213 = Multiply(x=w400, y=i8 8) -> (x*y=w394:i8)
        n214 = Number To Decimal String(number=w402) -> (decimal integer string=w407:string)  [unwired: 1 in]
        n215 = Number To Decimal String(number=w394) -> (decimal integer string=w405:string)  [unwired: 1 in]
        n216 = global read "CODMn断电保存全局变量.vi" "CODMn仪器参数"() -> (w396:T12)
        n217 = Concatenate Strings("L低量程范围:0~" ("量程解释说明"), w407, "(mg/L)\n\nH高量程范围:" ("量程解释说明"), "0" ("字符串"), "~" ("量程解释说明"), w405, "(mg/L)" ("量程解释说明")) -> (→"量程解释说明":string)
        n218 = Bundle By Name(cluster=w396, "测量量程"=w394) -> (w395:T12)
        n219 = global write "CODMn断电保存全局变量.vi" "CODMn仪器参数"(w395) -> ()
      }
    }
    n220 = flat-sequence {
      frame #0 {
        # "参数赋值（只在读取参数时候改变一次）"
        n221 = global read "COD内部交互全局.vi" "读取浮台参数显示"() -> (w224:bool)
        n222 = global read "COD内部交互全局.vi" "读取浮台参数"() -> (w223:u16[])
        n223 = global read "COD内部交互全局.vi" "读取参数显示"() -> (w225:bool)
        n224 = global read "COD内部交互全局.vi" "读取参数"() -> (w226:u16[])
        n225 = case shown="真" w224 {
          tunnel: w223 -> [_ w232]
          frame False {
          }
          frame True {
            n226 = Index Array(array=w232) -> (element #1=w231:u16, element #2=w230:u16, element #3=w229:u16, element #4=w228:u16)  [unwired: 4 in]
            n227 = global write "COD内部交互全局.vi" "读取浮台参数显示"(FALSE ("读取参数显示")) -> ()
            n228 = local write "采水泵进样时间/s:"(w231) -> ()
            n229 = local write "采水泵润洗时间/s:"(w230) -> ()
            n230 = local write "采水泵沉淀时间/s:"(w229) -> ()
            n231 = local write "采水泵排液时间/s:"(w228) -> ()
          }
        }
        n232 = case shown="真" w225 {
          tunnel: w226 -> [_ w254]
          frame False {
          }
          frame True {
            n233 = Index Array(array=w254) -> (element #1=w263:u16, element #2=w233:u16, element #3=w259:u16, element #4=w237:u16, element #5=w262:u16, element #6=w261:u16, element #7=w273:u16, element #8=w272:u16, element #9=w271:u16, element #10=w270:u16, element #11=w269:u16, element #12=w268:u16, element #13=w267:u16, element #14=w266:u16, element #15=w265:u16, element #16=w257:u16, element #17=w256:u16, element #18=w255:u16, element #19=w252:u16, element #20=w251:u16, element #21=w250:u16, element #22=w249:u16, element #23=w248:u16, element #27=w244:u16, element #28=w243:u16, element #29=w242:u16, element #30=w241:u16, element #31=w240:u16)  [unwired: 31 in, 3 out]
            n234 = global write "COD内部交互全局.vi" "读取参数显示"(FALSE ("读取参数显示")) -> ()
            n235 = local write "水样："(w261) -> ()
            n236 = local write "标液："(w272) -> ()
            n237 = local write "硫酸"(w267) -> ()
            n238 = global read "CODMn断电保存全局变量.vi" "CODMn仪器参数"() -> (w236:T12)
            n239 = local write "零点核查样："(w271) -> ()
            n240 = local write "加标回收样："(w270) -> ()
            n241 = local write "当前量程："(w262) -> ()
            n242 = local write "蒸馏水："(w273) -> ()
            n243 = local write "恒温时间"(w233) -> ()
            n244 = local write "高锰酸钾"(w269) -> ()
            n245 = local write "草酸钠"(w268) -> ()
            n246 = local write "零点泵计量数 2"(w266) -> ()
            n247 = local write "标度泵计量数 2"(w265) -> ()
            n248 = local write "高量程稀释倍数:"(w257) -> ()
            n249 = local write "低量程稀释倍数:"(w256) -> ()
            n250 = local write "CODMn零点核查选择"(w255) -> ()
            n251 = Build Array(w252, w251, w250, w249, w248) -> (w247:u16[])
            n252 = Build Array(w244, w243, w242, w241, w240) -> (w239:u16[])
            n253 = Divide(x=w263, y=u16 10) -> (x/y=w234:dbl)
            n254 = Divide(x=w259, y=u16 100) -> (x/y=w258:dbl)
            n255 = local write "氢氧化钠："(w237) -> ()
            n256 = local write "温度"(w234) -> ()
            n257 = local write "标准液浓度"(w258) -> ()
            n258 = call "HexToString.vi"("数组"=w239) -> ("字符串"=w238:string)  [unwired: 10 in]
            "CODMn序列号" <- w238
            "序列号" <- w238
            n259 = call "FATEK_HexToString.vi"("数组"=w247) -> ("STRING"=w246:string[])  [unwired: 10 in]
            n260 = Bundle By Name(cluster=w236, "消解温度"=w234, "消解时长"=w233) -> (w235:T12)
            n261 = Index Array(array=w246) -> (element=→"CODMn软件版本：":string)  [unwired: 1 in]
            n262 = global write "CODMn断电保存全局变量.vi" "CODMn仪器参数"(w235) -> ()
            n263 = global write "COD内部交互全局.vi" "序列号:"(w238) -> ()
          }
        }
      }
    }
    n264 = flat-sequence {
      frame #0 {
        # "权限隐藏和显示功能"
        n265 = local read "x = y?"() -> (w420:bool)
        n266 = global read "CODMn断电保存全局变量.vi" "CODMn系统周期测试?"() -> (w417:bool)
        n267 = global read "CODMn断电保存全局变量.vi" "运行周期"() -> (w418:T13)
        n268 = property on="更新程序" class="Bool (严格)"("Visible"=w420) -> ()  [unwired: 2 in, 2 out]
        n269 = property on="释放串口" class="Bool"("Visible"=w420) -> ()  [unwired: 2 in, 2 out]
        n270 = property on="打开串口" class="Bool"("Visible"=w420) -> ()  [unwired: 2 in, 2 out]
        n271 = case shown="假" w417 {
          tunnel: w418 -> [_ w441]
          tunnel: [T9."Enabled" ("禁用") w439] -> w416
          frame False {
          }
          frame True {
            n272 = Unbundle By Name(w441) -> ("运行模式"=w440:enum16{"维护模式", "常规模式", "应急模式", "质控模式"})
            n273 = case shown="\"维护模式\", 默认" w440 {
              tunnel: [T9."Enabled" ("禁用") T9."Disabled and Grayed Out" ("禁用") T9."Disabled and Grayed Out" ("禁用") T9."Disabled and Grayed Out" ("禁用")] -> w439
              frame "维护模式", Default {
              }
              frame "常规模式" {
              }
              frame "应急模式" {
              }
              frame "质控模式" {
              }
            }
          }
        }
        n274 = property on="序列号变更" class="Bool"("Visible"=w420) -> ()  [unwired: 2 in, 2 out]
        n275 = property on="常规版/认证版" class="Enum (严格)"("Visible"=w420) -> ()  [unwired: 2 in, 2 out]
        n276 = property on="CODMn零点核查选择" class="Enum (严格)"("Visible"=w420) -> ()  [unwired: 2 in, 2 out]
        n277 = property on="低量程稀释倍数:" class="DigNum (严格)"("Visible"=w420) -> ()  [unwired: 2 in, 2 out]
        n278 = property on="稀释倍数解释" class="Str"("Visible"=w420) -> ()  [unwired: 2 in, 2 out]
        n279 = property on="高量程稀释倍数:" class="DigNum (严格)"("Visible"=w420) -> ()  [unwired: 2 in, 2 out]
        n280 = control-ref of="水样："() -> (w430:refnum<vi>)
        n281 = control-ref of="蒸馏水："() -> (w429:refnum<vi>)
        n282 = control-ref of="标液："() -> (w428:refnum<vi>)
        n283 = control-ref of="零点核查样："() -> (w427:refnum<vi>)
        n284 = control-ref of="加标回收样："() -> (w426:refnum<vi>)
        n285 = local read "水样量程选择:"() -> (w434:enum16{"L", "H", "自动切换测一次", "自动切换测两次"})
        n286 = control-ref of="量程解释说明"() -> (w424:refnum<vi>)
        n287 = control-ref of="氢氧化钠："() -> (w425:refnum<vi>)
        n288 = property on="定时设置" class="定时设置 (严格)"("DisabledEnum"=w416) -> ()  [unwired: 2 in, 2 out]
        n289 = local read "常规版/认证版"() -> (w432:enum16{"常规版-酸性", "常规版-碱性", "认证版", "浮台版"})
        n290 = Not Equal To 0?(x=w434) -> (x != 0?=w433:bool)
        n291 = control-ref of="进样管"() -> (w422:refnum<vi>)
        n292 = case shown="\"认证版\"" w432 {
          tunnel: [T9."Enabled" ("禁用") T9."Enabled" ("禁用") T9."Disabled and Grayed Out" ("禁用") T9."Enabled" ("禁用")] -> _
          tunnel: [i32[] [2] ("禁用项[]") i32[] [2] ("禁用项[]") i32[] [] ("禁用项[]") i32[] [2] ("禁用项[]")] -> _
          tunnel: [w449 w454 T9."Disabled and Grayed Out" ("禁用") w465] -> _
          tunnel: [w448 FALSE FALSE TRUE] -> w431
          tunnel: [w449 w454 T9."Disabled and Grayed Out" ("禁用") w465] -> w421
          tunnel: [w448 TRUE FALSE FALSE] -> w419
          frame "常规版-酸性", Default {
            w448 = FALSE
            w449 = T9."Enabled" ("禁用")
          }
          frame "常规版-碱性" {
            w454 = T9."Enabled" ("禁用")
          }
          frame "认证版" {
            w460 = u16 1 items=["水样测试"=1, "标样核查"=2, "零点核查"=3, "跨度核查"=4, "空白测试"=5, "平行样"=6, "加标回收"=7] ("测量模式(公式)")
            n293 = global write "CODMn断电保存全局变量.vi" "测量模式(公式)"(w460) -> ()
          }
          frame "浮台版" {
            w465 = T9."Enabled" ("禁用")
          }
        }
        n294 = Build Array(w430, w429, w428, w427, w426, w424, w425, w422) -> (w423:refnum<vi>[])
        n295 = Select(t=T9."Enabled" ("禁用"), s=w433, f=T9."Disabled and Grayed Out" ("禁用")) -> (s? t:f=w435:T9)
        n296 = for {
          tunnel: w423 -> [w447] mode=indexing
          tunnel: w421 -> [w446]
          n297 = property class="Ctl"(reference=w447, "DisabledEnum"=w446) -> ()  [unwired: 1 in, 2 out]
        }
        n298 = property on="低切高阈值:" class="DigNum (严格)"("DisabledEnum"=w435) -> ()  [unwired: 2 in, 2 out]
        n299 = property on="高切低阈值:" class="DigNum (严格)"("DisabledEnum"=w435) -> ()  [unwired: 2 in, 2 out]
        n300 = property on="采水泵润洗时间/s:" class="DigNum (严格)"("Visible"=w431) -> ()  [unwired: 2 in, 2 out]
        n301 = property on="采水泵沉淀时间/s:" class="DigNum (严格)"("Visible"=w431) -> ()  [unwired: 2 in, 2 out]
        n302 = property on="采水泵排液时间/s:" class="DigNum (严格)"("Visible"=w431) -> ()  [unwired: 2 in, 2 out]
        n303 = property on="采水泵进样时间/s:" class="DigNum (严格)"("Visible"=w431) -> ()  [unwired: 2 in, 2 out]
        n304 = property on="氢氧化钠：" class="DigNum (严格)"("Visible"=w419) -> ()  [unwired: 2 in, 2 out]
        n305 = property on="氢氧化钠" class="DigNum (严格)"("Visible"=w419) -> ()  [unwired: 2 in, 2 out]
        n306 = property on="公式切换阈值滴定数(0-9999)" class="DigNum (严格)"("Visible"=TRUE) -> ()  [unwired: 2 in, 2 out]
      }
    }
    n307 = flat-sequence {
      frame #0 {
        # "公式读取显示（只在读取公式的时候改变一次）"
        n308 = global read "COD内部交互全局.vi" "读取公式显示"() -> (w274:bool)
        n309 = case shown="真" w274 {
          frame False {
          }
          frame True {
            n310 = global write "COD内部交互全局.vi" "读取公式显示"(FALSE ("读取参数显示")) -> ()
            n311 = global read "COD内部交互全局.vi" "读取公式"() -> (w295:u16[])
            n312 = Array Subset(array=w295, index=10 ("索引"), length=84 ("长度")) -> (w283:u16[])
            n313 = Index Array(array=w283, index #1=24 ("索引")) -> (element #1=w281:u16, element #2=w280:u16)  [unwired: 1 in]
            n314 = call "浮点CDAB转换COD.vi"("数组"=w283) -> ("数组 2"=w292:sgl[])  [unwired: 10 in]
            n315 = Array To Cluster(array=w292) -> (cluster=w294:T14)
            n316 = local read "量程选择"() -> (w285:enum16{"低量程", "高量程"})
            n317 = case shown="\"低量程\", 默认" w285 {
              tunnel: w294 -> [w303 w311]
              tunnel: [w302 w310] -> w288
              tunnel: [w301 w309] -> w287
              tunnel: [w300 w308] -> w286
              tunnel: w281 -> [w299 _]
              tunnel: w280 -> [_ w307]
              tunnel: [w298 w306] -> w277
              tunnel: [w297 w304] -> w276
              tunnel: [w296 w305] -> w275
              frame "低量程", Default {
                n318 = local write "公式切换阈值滴定数(0-9999)"(w299) -> ()
                n319 = Unbundle By Name(w303) -> ("数组 2[0]"=w302:sgl, "数组 2[1]"=w301:sgl, "数组 2[2]"=w300:sgl, "数组 2[3]"=w298:sgl, "数组 2[4]"=w297:sgl, "数组 2[5]"=w296:sgl)
              }
              frame "高量程" {
                n320 = local write "公式切换阈值滴定数(0-9999)"(w307) -> ()
                n321 = Unbundle By Name(w311) -> ("数组 2[6]"=w310:sgl, "数组 2[7]"=w309:sgl, "数组 2[8]"=w308:sgl, "数组 2[9]"=w306:sgl, "数组 2[10]"=w304:sgl, "数组 2[11]"=w305:sgl)
              }
            }
            n322 = Bundle By Name(cluster=cluster{"X":dbl, "b":dbl, "X^2":dbl} {"X"=0.0, "b"=0.0, "X^2"=0.0} ("方程系数"), "X"=w288, "b"=w287, "X^2"=w286) -> (w293:cluster{"X":dbl, "b":dbl, "X^2":dbl})
            n323 = Bundle By Name(cluster=cluster{"X":dbl, "b":dbl, "X^2":dbl} {"X"=0.0, "b"=0.0, "X^2"=0.0} ("方程系数"), "X"=w277, "b"=w276, "X^2"=w275) -> (w278:cluster{"X":dbl, "b":dbl, "X^2":dbl})
            n324 = local write "方程系数 2"(w278) -> ()
            n325 = local write "方程系数"(w293) -> ()
          }
        }
      }
    }
    n326 = Wait (ms)(milliseconds to wait=u32 1000 ("等待时间（毫秒）")) -> ()  [unwired: 1 out]
  }
  n327 = while {
    stop <- FALSE stop-if-true
    w503 = T15 0 items=["最小二乘", "最小绝对残差", "Bisquare"] ("method")
    # "计算线性、多项式公式、远程校准"
    n328 = local read "浓度1"() -> (w485:dbl)
    n329 = local read "浓度2"() -> (w504:dbl)
    n330 = local read "浓度3"() -> (w505:dbl)
    n331 = local read "浓度4"() -> (w499:dbl)
    n332 = local read "浓度5"() -> (w498:dbl)
    n333 = Build Array("泵滴定数1", "泵滴定数2", "泵滴定数3", "泵滴定数4", "泵滴定数5") -> (w470:dbl[])
    n334 = Build Array(w485, w504, w505, w499, w498) -> (w469:dbl[])
    n335 = Build Array("启用1", "启用2", "启用3", "启用4", "启用5") -> (w471:bool[])
    n336 = call "将启用的浓度作为新的浓度数组.vi"("启用布尔数组"=w471, "输入浓度数组"=w469) -> ("启用的浓度数组"=w484:dbl[])  [unwired: 13 in]
    n337 = global read "CODMN外部API.vi" "远程反控校准CODMn"() -> (w483:bool)
    n338 = call "CODMn线性公式.vi"("标液浓度"=w469, "滴定数"=w470, "启用"=w471, "method"=w503, "模型"="模型", "精度"=6) -> ("Polynomial Coefficients 2"=w474:dbl[], "拟合方程"=w491:string, "r^2"=w473:dbl, "拟合方程 2"=w479:string, "r^2 2"=→"r^2 2":dbl, "XY图"=→"XY图":cluster{"X Values":dbl[], "Y Values":dbl[]}[], "Polynomial Coefficients"=w500:dbl[])  [unwired: 7 in]
    "拟合公式" <- w491
    "r^2" <- w473
    "拟合公式 2" <- w479
    n339 = global write "COD内部交互全局.vi" "启用的浓度数组"(w484) -> ()
    n340 = feedback #3(w479) -> (w480:string)
    n341 = feedback-in #3(w479) -> ()
    n342 = feedback #4(w491) -> (w492:string)
    n343 = feedback-in #4(w491) -> ()
    n344 = Not Equal?(x=w479, y=w480) -> (x != y?=w477:bool)
    n345 = call <vilib>:"Boolean Crossing PtByPt.vi"("direction"=enum16{"either", "false-true", "true-false"}."false-true", "input"=w483) -> ("crossing"=w482:bool)  [unwired: 1 in]
    n346 = Not Equal?(x=w491, y=w492) -> (x != y?=w478:bool)
    n347 = Or(x=w478, y=w477) -> (x .or. y?=w476:bool)
    n348 = case shown="真" w476 {
      tunnel: w500 -> [_ w525]
      tunnel: w474 -> [_ w521]
      tunnel: w473 -> [_ w517]
      tunnel: "模型" -> [_ w515]
      tunnel: w471 -> [_ w514]
      tunnel: w470 -> [_ w513]
      tunnel: w469 -> [_ w512]
      frame False {
      }
      frame True {
        # "当公式发生改变时赋值到右侧公式"
        n349 = case shown="\"折线\"" w515 {
          tunnel: [9999.0 ("泵滴定数5") 9999.0 ("泵滴定数5") w530] -> w516
          tunnel: w513 -> [_ _ w536]
          tunnel: w514 -> [_ _ w537]
          tunnel: w512 -> [_ _ w535]
          frame "线性", Default {
          }
          frame "多项式" {
          }
          frame "折线" {
            n350 = call "监测浓度升序排列 (子VI).vi"("标液浓度"=w535, "滴定数"=w536, "启用"=w537) -> ("输出数组"=w531:dbl[][])  [unwired: 8 in]
            n351 = Index Array(array=w531, index (col)=0 ("禁用的索引 (列)")) -> (element=w533:dbl[])  [unwired: 1 in]
            n352 = Index Array(array=w533, index=1 ("索引")) -> (element=w530:dbl)
          }
        }
        n353 = Rotate 1D Array(1:w525, 2:-1 ("n")) -> (0:w526:dbl[])
        n354 = Rotate 1D Array(1:w521, 2:-1 ("n")) -> (0:w523:dbl[])
        n355 = global read "CODMn断电保存全局变量.vi" "CODMn仪器参数"() -> (w519:T12)
        n356 = Array To Cluster(array=w526) -> (cluster=w524:cluster{"[0]":dbl, "[1]":dbl, "[2]":dbl})
        n357 = Array To Cluster(array=w523) -> (cluster=w520:cluster{"[0]":dbl, "[1]":dbl, "[2]":dbl})
        n358 = Bundle By Name(cluster=w519, "线性相关系数"=w517) -> (w518:T12)
        n359 = global write "CODMn断电保存全局变量.vi" "CODMn仪器参数"(w518) -> ()
        n360 = local write "公式切换阈值滴定数(0-9999)"(w516) -> ()
        n361 = local write "方程系数"(w524) -> ()
        n362 = local write "方程系数 2"(w520) -> ()
      }
    }
    n363 = case shown="真" w482 {
      tunnel: w469 -> [_ _]
      frame False {
      }
      frame True {
        n364 = global read "CODMn断电保存全局变量.vi" "远程标样校准"() -> (w510:enum16{"标液1", "标液2", "标液3", "标液4"})
        n365 = local read "远程校准量程"() -> (w508:enum16{"低量程", "高量程"})
        n366 = Increment(x=w510) -> (x+1=w509:enum16{"标液1", "标液2", "标液3", "标液4"})
        n367 = property on="量程选择" class="Enum (严格)"("Val(Sgnl)"=w508) -> ()  [unwired: 2 in, 2 out]
        n368 = Increment(x=w509) -> (x+1=w511:enum16{"标液1", "标液2", "标液3", "标液4"})
        n369 = global write "COD内部交互全局.vi" "当前校准"(w511) -> ()
      }
    }
    n370 = Wait (ms)(milliseconds to wait=u32 1000 ("等待时间（毫秒）")) -> ()  [unwired: 1 out]
  }
  n371 = while {
    tunnel: w15 -> [w547]
    tunnel: w14 -> [w546]
    tunnel: w5 -> [_]
    stop <- FALSE stop-if-true
    # "主循环界面显示"
    n372 = flat-sequence {
      frame #0 {
        # "A，B，K"
        # "CODMn读取状态"
        n373 = global read "COD内部交互全局.vi" "ORP、时间"() -> (w682:u16[])
        n374 = To Word Integer(number=w682) -> (16bit integer=w703:i16[])
        n375 = Split 1D Array(array=w703, index=3 ("索引")) -> (first subarray=w684:i16[], second subarray=w702:i16[])
        n376 = Index Array(array=w684) -> (element #1=w688:i16, element #2=w687:i16, element #3=w686:i16)  [unwired: 3 in]
        n377 = Index Array(array=w702) -> (element #1=w697:i16, element #2=w701:i16, element #3=w700:i16, element #4=w699:i16)  [unwired: 4 in]
        n378 = To Single Precision Float(number=w699) -> (single precision float=w690:sgl)
        n379 = Build Array(w688, w687, w686) -> (w685:i16[])
        n380 = To Single Precision Float(number=w697) -> (single precision float=w696:sgl)
        n381 = To Single Precision Float(number=w701) -> (single precision float=w695:sgl)
        n382 = To Single Precision Float(number=w700) -> (single precision float=w691:sgl)
        n383 = call "HexToDate.vi"("数组"=w685) -> ("DATE"=w689:timestamp[])  [unwired: 10 in]
        n384 = Number To Decimal String(number=w695) -> (decimal integer string=→"ORP-A":string)  [unwired: 1 in]
        n385 = Number To Decimal String(number=w691) -> (decimal integer string=→"ORP-B":string)  [unwired: 1 in]
        n386 = Number To Decimal String(number=w690) -> (decimal integer string=→"ORP-K":string)  [unwired: 1 in]
        n387 = Divide(x=w696, y=sgl 100.0) -> (x/y=→"COD浓度（mg/L)":sgl)
        n388 = Index Array(array=w689) -> (element=w683:timestamp)  [unwired: 1 in]
        n389 = Format Date/Time String(seconds (now)=w683) -> (date/time string=→"数据时间":string)  [unwired: 2 in]
      }
    }
    n390 = flat-sequence {
      frame #0 {
        # "测量状态显示"
        n391 = global read "COD内部交互全局.vi" "测量状态"() -> (w596:u16[])
        n392 = To Word Integer(number=w596) -> (16bit integer=w606:i16[])
        n393 = Index Array(array=w606, index #1=0 ("索引"), index #4=3 ("索引"), index #14=13 ("索引"), index #15=14 ("索引"), index #21=20 ("索引"), index #32=31 ("索引")) -> (element #1=w610:i16, element #2=w609:i16, element #3=w608:i16, element #4=w592:i16, element #5=→"模式（受控）":i16, element #6=→"进样管":i16, element #7=→"高锰酸钾":i16, element #8=→"草酸钠":i16, element #9=→"硫酸":i16, element #10=w605:i16, element #11=w625:i16, element #12=w601:i16, element #13=→"报警数字":i16, element #14=w631:i16, element #15=w616:i16, element #16=→"多列列表框":i16, element #20=→"氢氧化钠":i16, element #21=w589:i16, element #33=→"分":i16, element #34=→"秒":i16)  [unwired: 28 in, 14 out]
        "CODMn工作状态" <- w592
        n394 = global write "COD内部交互全局.vi" "基本量程实时读取"(w589) -> ()
        n395 = Build Array(w610, w609, w608) -> (w611:i16[])
        n396 = To Single Precision Float(number=w605) -> (single precision float=→"实时ORP":sgl)
        n397 = Number To Decimal String(number=w589) -> (decimal integer string=→"基本量程(显示)":string)  [unwired: 1 in]
        n398 = Equal?(x=w601, y=u16 1) -> (x = y?=→"排液标记":bool)
        n399 = Equal?(x=w601, y=u16 2) -> (x = y?=→"断电排液标记":bool)
        n400 = Divide(x=w625, y=u16 10) -> (x/y=→"温度℃":dbl)
        n401 = Divide(x=w631, y=u16 1000) -> (x/y=→"零点滴定值":dbl)
        n402 = Divide(x=w616, y=u16 1000) -> (x/y=→"标度滴定值":dbl)
        n403 = Equal?(x=w592, y=T3."水样测试" ("CODMn工作状态")) -> (x = y?=w590:bool)
        n404 = call "HexToDate.vi"("数组"=w611) -> ("DATE"=w607:timestamp[])  [unwired: 10 in]
        n405 = case shown="真" w590 {
          tunnel: w589 -> [_ w634]
          frame False {
          }
          frame True {
            n406 = global write "CODMn断电保存全局变量.vi" "水样测试量程"(w634) -> ()
          }
        }
        n407 = Index Array(array=w607) -> (element=→"仪器时间":timestamp)  [unwired: 1 in]
      }
    }
    n408 = flat-sequence {
      frame #0 {
        # "报警状态显示"
        n409 = global read "COD内部交互全局.vi" "报警点位"() -> (w649:bool[])
        n410 = Index Array(array=w649, index #1=0 ("索引")) -> (element #1=w646:bool, element #2=w645:bool, element #3=w644:bool, element #4=w643:bool, element #5=w642:bool, element #6=w641:bool, element #7=w640:bool, element #8=w639:bool, element #9=w638:bool, element #11=w637:bool, element #13=w636:bool, element #14=w635:bool)  [unwired: 13 in, 2 out]
        "ORP故障" <- w646
        "温控器故障" <- w645
        "加热故障" <- w638
        "高锰酸钾报警" <- w640
        "草酸钠报警" <- w639
        "测量错误" <- w644
        "校零错误" <- w643
        "校标错误" <- w642
        "进水样超量程" <- w641
        "排液故障" <- w637
        "60分钟超时报警" <- w636
        "进样无液体告警" <- w635
        n411 = Compound Arithmetic op=OR ("复合运算")(w646, w645, w638, w640, w639, w644, w642, w643, w641, w637, w636) -> (→"故障标记":bool)
        n412 = Bundle By Name(cluster=T16 {"ORP故障"=FALSE, "温控器故障"=FALSE, "加热故障"=FALSE, "高锰酸钾报警"=FALSE, "草酸钠报警"=FALSE, "测量错误"=FALSE, "校零错误"=FALSE, "校标错误"=FALSE, " 进水样超量程"=FALSE, "排液阀故障"=FALSE, "60分钟超时报警"=FALSE, "进样无液体报警"=FALSE} ("报警簇"), "ORP故障"=w646, "温控器故障"=w645, "加热故障"=w638, "高锰酸钾报警"=w640, "草酸钠报警"=w639, "测量错误"=w644, "校零错误"=w643, "校标错误"=w642, "进水样超量程"=w641, "排液阀故障"=w637, "60分钟超时报警"=w636, "进样无液体报警"=w635) -> (w647:T16)
        n413 = global write "COD内部交互全局.vi" "报警簇"(w647) -> ()
      }
    }
    n414 = flat-sequence {
      frame #0 {
        # "CODMn读取状态"
        n415 = global read "COD内部交互全局.vi" "温度"() -> (w679:bool[])
        n416 = global read "COD内部交互全局.vi" "M输出点"() -> (w678:bool[])
        n417 = Index Array(array=w679) -> (element=→"加热":bool)  [unwired: 1 in]
        n418 = Index Array(array=w678) -> (element #1=→"搅拌":bool, element #4=→"进水样":bool, element #5=→"进蒸馏水":bool, element #6=→"进标液":bool, element #7=→"进零点核查样":bool, element #8=→"进加标回收样":bool, element #9=→"进高锰酸钾":bool, element #10=→"进草酸钠":bool, element #11=→"进硫酸":bool)  [unwired: 11 in, 2 out]
      }
    }
    n419 = flat-sequence {
      frame #0 {
        # "工作状态显示"
        n420 = local read "CODMn工作状态"() -> (w557:T3)
        n421 = case shown="\"标样校准\"" w557 {
          tunnel: [_ u16 0 ("y") u16 1 ("y") u16 2 ("y") u16 3 ("y") u16 4 ("y") u16 6 ("y") _ u16 7 ("y") u16 8 ("y") u16 5 ("y")] -> w556
          frame "空闲", Default {
          }
          frame "水样测试" {
          }
          frame "标样核查" {
          }
          frame "零点核查" {
          }
          frame "跨度核查" {
          }
          frame "空白测试" {
          }
          frame "平行样测试" {
          }
          frame "质控样" {
          }
          frame "空白校准" {
          }
          frame "标样校准" {
          }
          frame "加标回收" {
          }
        }
        n422 = Equal?(x=w557, y=u16 8) -> (x = y?=→"校零标记":bool)
        n423 = Equal?(x=w557, y=u16 4) -> (x = y?=→"跨度核查标记":bool)
        n424 = Equal?(x=w557, y=u16 0) -> (x = y?=→"待机":bool)
        n425 = Equal?(x=w557, y=u16 3) -> (x = y?=→"零点核查标记":bool)
        n426 = Equal?(x=w557, y=u16 7) -> (x = y?=→"质控样测量":bool)
        n427 = Equal?(x=w557, y=u16 1) -> (x = y?=→"水样测量":bool)
        n428 = Equal?(x=w557, y=u16 2) -> (x = y?=→"标样核查标记":bool)
        n429 = Equal?(x=w557, y=u16 6) -> (x = y?=→"平行样测量":bool)
        n430 = Equal?(x=w557, y=u16 9) -> (x = y?=→"校标标记":bool)
        n431 = Equal?(x=w557, y=u16 5) -> (x = y?=→"空白测试标记":bool)
        n432 = Equal?(x=w557, y=u16 10) -> (x = y?=→"加标回收测量":bool)
        n433 = global write "COD内部交互全局.vi" "测量模式数字"(w556) -> ()
      }
    }
    n434 = Get Date/Time In Seconds() -> (seconds since 1Jan1904=→"系统时间":timestamp)
    n435 = First Call?() -> (First Call?: T/F=w545:bool)
    n436 = Wait (ms)(milliseconds to wait=u32 1000 ("等待时间（毫秒）")) -> ()  [unwired: 1 out]
    n437 = case shown="真" w545 {
      tunnel: w547 -> [w653 w664]
      tunnel: w546 -> [w652 w663]
      tunnel: [w653 w655] -> w543
      tunnel: [w652 w654] -> w542
      frame False {
      }
      frame True {
        n438 = Bundle By Name(cluster=cluster{"命令":string} {"命令"=""} ("元素"), "命令"="CODMn读取参数" ("名称（未命名）")) -> (w667:cluster{"命令":string})
        n439 = Enqueue Element(queue=w664, element=w667, timeout in ms (-1)=1000 ("超时毫秒(-1)"), error in (no error)=w663) -> (queue out=w657:refnum<queue>, error out=w656:errorcluster)  [unwired: 1 out]
        n440 = Bundle By Name(cluster=cluster{"命令":string} {"命令"=""} ("元素"), "命令"="CODMn读取公式" ("名称（未命名）")) -> (w658:cluster{"命令":string})
        n441 = Enqueue Element(queue=w657, element=w658, timeout in ms (-1)=1000 ("超时毫秒(-1)"), error in (no error)=w656) -> (queue out=w655:refnum<queue>, error out=w654:errorcluster)  [unwired: 1 out]
      }
    }
    n442 = Get Queue Status(queue=w543, error in (no error)=w542) -> (queue out=w539:refnum<queue>, error out=w538:errorcluster, # elements in queue=w541:i32)  [unwired: 1 in, 5 out]
    n443 = Equal To 0?(x=w541) -> (x = 0?=w540:bool)
    n444 = case shown="真" w540 {
      tunnel: w539 -> [_ w551]
      tunnel: w538 -> [_ w550]
      frame False {
      }
      frame True {
        n445 = Bundle By Name(cluster=cluster{"命令":string} {"命令"=""} ("元素"), "命令"="CODMn读取" ("名称（未命名）")) -> (w553:cluster{"命令":string})
        n446 = Enqueue Element(queue=w551, element=w553, timeout in ms (-1)=1000 ("超时毫秒(-1)"), error in (no error)=w550) -> ()  [unwired: 3 out]
      }
    }
  }
  n447 = while {
    tunnel: w15 -> [w706]
    tunnel: w14 -> [w705]
    stop <- FALSE stop-if-true
    # "主线事件"
    n448 = event shown="[18] \"校准1\", \"校准2\", \"校准3\", \"校准4\", \"校准5\": 值改变" {
      selector: _ -> [_ _ _ _ _ _ _ _ _ _ _ _ _ _ _ _ _ _ _ _ _ _ _ _ _ _ _ _ _ _ _]
      dyn-events: _ -> [_ _ _ _ _ _ _ _ _ _ _ _ _ _ _ _ _ _ _ _ _ _ _ _ _ _ _ _ _ _ _]
      timeout: _ -> [_ _ _ _ _ _ _ _ _ _ _ _ _ _ _ _ _ _ _ _ _ _ _ _ _ _ _ _ _ _ _]
      tunnel: w706 -> [_ _ _ _ _ w797 _ _ w830 w968 w1094 _ _ _ _ _ _ _ w1307 _ _ _ w1570 _ _ _ w1634 w1641 w1663 w1706 _]
      tunnel: w705 -> [_ _ _ _ _ w796 _ _ w829 w967 w1093 _ _ _ _ _ _ _ w1304 _ _ _ w1569 _ _ _ w1633 w1640 w1662 w1705 _]
      event "单步启动": Value Change {
        n449 = event-data() -> ()  [unwired: 1 in, 6 out]
        n450 = call "CODMn手动控制框.vi"() -> ()  [unwired: 12 in]
      }
      event "启动": Mouse Down {
        n451 = event-data() -> ()  [unwired: 1 in, 8 out]
        n452 = global read "COD内部交互全局.vi" "基本量程实时读取"() -> (w710:enum16{"L", "H", "AUTO"})
        n453 = call "启动测量模式选择对话框.vi"("量程选择"=w710) -> ("标样浓度输出"=w708:dbl, "量程选择输出"=w709:enum16{"L", "H", "AUTO"}, "启动选择输出"=w714:u16)  [unwired: 8 in]
        n454 = Not Equal?(x=w714, y=u16 8) -> (x != y?=w711:bool)
        n455 = Not Equal?(x=w714, y=u16 7) -> (x != y?=w712:bool)
        n456 = And(x=w712, y=w711) -> (x .and. y?=w716:bool)
        n457 = case shown="真" w716 {
          tunnel: w714 -> [_ w731]
          tunnel: w709 -> [_ w722]
          tunnel: w708 -> [_ w721]
          frame False {
            n458 = One Button Dialog(message="请到校准配置里面进行校准操作！" ("消息")) -> ()  [unwired: 1 in, 1 out]
          }
          frame True {
            n459 = Not Equal?(x=w731, y=u16 9) -> (x != y?=w726:bool)
            n460 = case shown="\"H\"" w722 {
              tunnel: [w732 w736 errorcluster {"status"=FALSE, "code"=0, "source"=""} ("error out")] -> w720
              frame "L", Default {
                n461 = call "CODMnMB_api.vi"("STEP"=enum16{"open", "read", "write", "close"}."write", "values"=u16[] [0], "starting address"=u16 4276) -> ("error out"=w732:errorcluster)  [unwired: 6 in, 2 out]
              }
              frame "H" {
                n462 = call "CODMnMB_api.vi"("STEP"=enum16{"open", "read", "write", "close"}."write", "values"=u16[] [1], "starting address"=u16 4276) -> ("error out"=w736:errorcluster)  [unwired: 6 in, 2 out]
              }
              frame "AUTO" {
              }
            }
            n463 = global write "CODMN外部API.vi" "手动启动CODMn"(w726) -> ()
            n464 = call "单步测试一键复位.vi"("Error in"=w720) -> ("error out"=w719:errorcluster)  [unwired: 10 in]
            n465 = call <vilib>:"Clear Errors.vi"("error in (no error)"=w719) -> ("error out"=w718:errorcluster)  [unwired: 5 in, 1 out]
            n466 = case shown="0" w731 {
              tunnel: [u16 4608 ("address") u16 4608 ("address") u16 4608 ("address") u16 4608 ("address") u16 4608 ("address") u16 4608 ("address") u16 4608 ("address") u16 4608 ("address") u16 4608 ("address") u16 4608 ("address")] -> w724
              tunnel: [u16 1 ("address") u16 2 ("address") u16 3 ("address") u16 4 ("address") u16 5 ("address") u16 7 ("address") u16 6 ("address") u16 8 ("address") u16 9 ("address") u16 0 ("address")] -> w728
              tunnel: w721 -> [_ w744 _ _ _ _ _ _ _ _]
              frame 0 {
              }
              frame 1 {
                n467 = property on="标样浓度" class="DigNum (严格)"("Val(Sgnl)"=w744) -> ()  [unwired: 2 in, 2 out]
              }
              frame 2 {
              }
              frame 3 {
              }
              frame 4 {
              }
              frame 5 {
              }
              frame 6 {
              }
              frame 7 {
              }
              frame 8 {
              }
              frame 9, Default {
              }
            }
            n468 = Insert Into Array(array=u16[] [] ("values"), index=0 ("索引"), new element=w728) -> (w723:u16[])
            n469 = call "CODMnMB_api.vi"("STEP"=enum16{"open", "read", "write", "close"}."write", "Error in"=w718, "values"=w723, "starting address"=w724) -> ()  [unwired: 5 in, 3 out]
          }
        }
      }
      event "停止": Value Change {
        n470 = event-data() -> ()  [unwired: 1 in, 6 out]
        n471 = Two Button Dialog(message="确认是否停止？" ("消息"), 1:"否" ("F按钮名称（“取消”）"), 2:"是" ("T按钮名称（“确定”）")) -> (T button?=w764:bool)
        n472 = case shown="真" w764 {
          frame False {
          }
          frame True {
            n473 = Obtain Notifier(name (unnamed)="CODMn" ("名称（未命名）"), notification data type=FALSE) -> (notifier out=w770:refnum<notifier>, error out=w768:errorcluster)  [unwired: 2 in, 1 out]
            n474 = Send Notification(notification=TRUE ("通知"), notifier=w770, error in (no error)=w768) -> (notifier out=w767:refnum<notifier>, error out=w766:errorcluster)
            n475 = Release Notifier(notifier=w767, error in (no error)=w766) -> ()  [unwired: 1 in, 3 out]
            n476 = call "CODMnMB_api.vi"("STEP"=enum16{"open", "read", "write", "close"}."write", "values"=u16[] [11], "starting address"=u16 4608) -> ()  [unwired: 6 in, 3 out]
          }
        }
      }
      event "手动控制": Value Change {
        n477 = event-data() -> ()  [unwired: 1 in, 6 out]
        n478 = call "数字密码键盘.vi"() -> ("NewNumber"=w776:sgl)  [unwired: 1 in]
        n479 = Equal?(x=w776, y=8.0) -> (x = y?=w777:bool)
        n480 = case shown="假" w777 {
          frame False {
            n481 = call "窗口弹出对话框(子VI).vi"("消息"="密码错误") -> ()  [unwired: 10 in, 1 out]
          }
          frame True {
          }
        }
      }
      event "锁定按钮": Mouse Down {
        n482 = event-data() -> ("CtlRef"=w782:refnum<vi>)  [unwired: 1 in, 7 out]
        n483 = property class="Bool (严格)"(reference=w782) -> ("Value"=w781:bool)  [unwired: 1 in, 2 out]
        n484 = case shown="真" w781 {
          selector: w781 -> [w783 _]
          tunnel: [w783 w787] -> w780
          frame False {
          }
          frame True {
            n485 = call "数字密码键盘.vi"() -> ("NewNumber"=w784:sgl)  [unwired: 1 in]
            n486 = Equal?(x=w784, y=23506.0) -> (x = y?=w788:bool)
            n487 = Equal?(x=w784, y=8.0) -> (x = y?=w785:bool)
            n488 = Or(x=w788, y=w785) -> (x .or. y?=w787:bool)
            n489 = case shown="假" w787 {
              selector: w787 -> [w791 _]
              frame False {
                n490 = local write "锁定按钮"(w791) -> ()
                n491 = One Button Dialog(message="密码错误!" ("消息")) -> ()  [unwired: 1 in, 1 out]
              }
              frame True {
                n492 = One Button Dialog(message="解锁成功!" ("消息")) -> ()  [unwired: 1 in, 1 out]
              }
            }
          }
        }
        "x = y?" <- w780
      }
      event "参数配置": Value Change {
        (unwired) u16 20 ("number of holding registers")
        (unwired) u16 4272 ("starting address")
        n493 = event-data() -> ()  [unwired: 1 in, 6 out]
        n494 = global read "CODMN外部API.vi" "ping"() -> (w795:bool)
        n495 = property on="窗格" class="Pane"("Origin"=T4 {"Horizontal"=0, "Vertical"=650} ("原点")) -> ()  [unwired: 2 in, 2 out]
        n496 = case shown="假" w795 {
          tunnel: [w807 w810] -> w794
          frame False {
            n497 = global read "COD内部交互全局.vi" "配置文件ini"() -> (w809:string)
            n498 = call <vilib>:"Application Directory.vi"() -> ("Application Directory"=w808:path)
            n499 = Build Path(base path=w808, name or relative path=w809) -> (appended path=w807:path)
          }
          frame True {
            n500 = global read "CODMN外部API.vi" "配置文件 path"() -> (w810:path)
          }
        }
        n501 = Bundle By Name(cluster=cluster{"命令":string} {"命令"=""} ("元素"), "命令"="CODMn读取参数" ("名称（未命名）")) -> (w798:cluster{"命令":string})
        n502 = call <vilib>:"Open Config Data.vi"("configuration file path"=w794) -> ("error out"=w804:errorcluster, "refnum"=w801:T6)  [unwired: 8 in, 1 out]
        n503 = Enqueue Element(queue=w797, element=w798, error in (no error)=w796) -> ()  [unwired: 1 in, 3 out]
        n504 = vi-ref "斯坦道CODMn.lvlib:CODMn断电保存全局变量.vi"() -> (w802:refnum<vi>)
        n505 = call <userlib>:"Read Panel from INI__ogtk.vi"("error in (no error)"=w804, "VI ref"=w802, "refnum"=w801) -> ("error out"=w805:errorcluster, "refnum out"=w803:T6)  [unwired: 7 in]
        n506 = call <vilib>:"Close Config Data.vi"("error in (no error)"=w805, "refnum"=w803) -> ("error out"=w793:errorcluster)  [unwired: 8 in, 1 out]
        n507 = call <vilib>:"Clear Errors.vi"("error in (no error)"=w793) -> ()  [unwired: 5 in, 2 out]
      }
      event "保存": Mouse Down {
        n508 = event-data() -> ()  [unwired: 1 in, 8 out]
        n509 = local read "通讯状态"() -> (w811:bool)
        n510 = Two Button Dialog(message="确定保存参数，保存参数将会替换原有参数！" ("消息")) -> (T button?=w813:bool)  [unwired: 2 in]
        n511 = case shown="真" w813 {
          tunnel: w811 -> [_ w814]
          frame False {
          }
          frame True {
            n512 = case shown="真" w814 {
              frame False {
                n513 = One Button Dialog(message="保存失败，当前无通讯！" ("消息")) -> ()  [unwired: 1 in, 1 out]
              }
              frame True {
                n514 = One Button Dialog(message="参数保存成功！" ("消息")) -> ()  [unwired: 1 in, 1 out]
                n515 = Build Array("采水泵进样时间/s:", "采水泵润洗时间/s:", "采水泵沉淀时间/s:", "采水泵排液时间/s:") -> (w817:i32[])
                n516 = call "CODMnMB_api.vi"("STEP"=enum16{"open", "read", "write", "close"}."write", "values"="保存参数", "starting address"=u16 4272) -> ("error out"=w823:errorcluster)  [unwired: 6 in, 2 out]
                n517 = call "CODMnMB_api.vi"("STEP"=enum16{"open", "read", "write", "close"}."write", "Error in"=w823, "values"=w817, "starting address"=u16 5596) -> ()  [unwired: 5 in, 3 out]
              }
            }
          }
        }
      }
      event "常规版/认证版": Value Change {
        n518 = event-data() -> ()  [unwired: 1 in, 6 out]
        n519 = flat-sequence {
          frame #0 {
            n520 = global write "CODMn断电保存全局变量.vi" "常规版/认证版"("常规版/认证版") -> ()
          }
          frame #1 {
            n521 = call "配置文件保存.vi"() -> ()  [unwired: 12 in]
          }
        }
      }
      event "校准配置": Value Change {
        w843 = "量程选择" ("section")
        n522 = event-data() -> ()  [unwired: 1 in, 6 out]
        n523 = global read "CODMN外部API.vi" "ping"() -> (w847:bool)
        n524 = property on="窗格" class="Pane"("Origin"=T4 {"Horizontal"=0, "Vertical"=1300} ("原点")) -> ()  [unwired: 2 in, 2 out]
        n525 = case shown="假" w847 {
          tunnel: [w925 w928] -> w846
          frame False {
            n526 = global read "COD内部交互全局.vi" "配置文件ini"() -> (w927:string)
            n527 = call <vilib>:"Application Directory.vi"() -> ("Application Directory"=w926:path)
            n528 = Build Path(base path=w926, name or relative path=w927) -> (appended path=w925:path)
          }
          frame True {
            n529 = global read "CODMN外部API.vi" "配置文件 path"() -> (w928:path)
          }
        }
        n530 = Bundle By Name(cluster=cluster{"命令":string} {"命令"=""} ("元素"), "命令"="CODMn读取公式" ("名称（未命名）")) -> (w831:cluster{"命令":string})
        n531 = Enqueue Element(queue=w830, element=w831, error in (no error)=w829) -> ()  [unwired: 1 in, 3 out]
        n532 = call <vilib>:"Open Config Data.vi"("configuration file path"=w846) -> ("error out"=w864:errorcluster, "refnum"=w865:T6)  [unwired: 8 in, 1 out]
        n533 = call-poly <vilib>:"Read Key.vi"("section"="CODMn模型选择" ("key"), "error in (no error)"=w864, "key"="线性和多项式", "refnum"=w865) -> ("error out"=w861:errorcluster, "value"=w863:i32, "refnum out"=w862:T6)  [unwired: 4 in, 1 out]
        n534 = local write "模型"(w863) -> ()
        n535 = call-poly <vilib>:"Read Key.vi"("section"="标线选择", "error in (no error)"=w861, "key"="选用水样", "refnum"=w862) -> ("error out"=w844:errorcluster, "value"=w848:i32, "refnum out"=w845:T6)  [unwired: 4 in, 1 out]
        n536 = local write "选用水样"(w848) -> ()
        n537 = case shown="0, 默认" w848 {
          tunnel: ["葡萄糖标线" ("section") "草酸钠标线" ("section")] -> w870
          frame 0, Default {
          }
          frame 1 {
          }
        }
        n538 = call-poly <vilib>:"Read Key.vi"("section"=w843, "error in (no error)"=w844, "key"=w843, "refnum"=w845) -> ("error out"=w841:errorcluster, "value"=w840:i32, "refnum out"=w842:T6)  [unwired: 4 in, 1 out]
        n539 = local write "量程选择"(w840) -> ()
        n540 = case shown="2" w840 {
          tunnel: ["低量程" "高量程" "0-2量程"] -> w869
          frame 0, Default {
          }
          frame 1 {
          }
          frame 2 {
          }
        }
        n541 = Concatenate Strings(w870, w869) -> (w868:string)
        n542 = call-poly <vilib>:"Read Key.vi"("section"=w868, "error in (no error)"=w841, "key"="浓度1", "refnum"=w842) -> ("error out"=w895:errorcluster, "value"=w893:dbl, "refnum out"=w894:T6)  [unwired: 4 in, 1 out]
        n543 = local write "浓度1"(w893) -> ()
        n544 = call-poly <vilib>:"Read Key.vi"("section"=w868, "error in (no error)"=w895, "key"="浓度2", "refnum"=w894) -> ("error out"=w909:errorcluster, "value"=w896:dbl, "refnum out"=w908:T6)  [unwired: 4 in, 1 out]
        n545 = local write "浓度2"(w896) -> ()
        n546 = call-poly <vilib>:"Read Key.vi"("section"=w868, "error in (no error)"=w909, "key"="浓度3", "refnum"=w908) -> ("error out"=w910:errorcluster, "value"=w898:dbl, "refnum out"=w907:T6)  [unwired: 4 in, 1 out]
        n547 = local write "浓度3"(w898) -> ()
        n548 = call-poly <vilib>:"Read Key.vi"("section"=w868, "error in (no error)"=w910, "key"="泵滴定数1", "refnum"=w907) -> ("error out"=w911:errorcluster, "value"=w900:dbl, "refnum out"=w906:T6)  [unwired: 4 in, 1 out]
        n549 = local write "泵滴定数1"(w900) -> ()
        n550 = call-poly <vilib>:"Read Key.vi"("section"=w868, "error in (no error)"=w911, "key"="泵滴定数2", "refnum"=w906) -> ("error out"=w905:errorcluster, "value"=w903:dbl, "refnum out"=w912:T6)  [unwired: 4 in, 1 out]
        n551 = local write "泵滴定数2"(w903) -> ()
        n552 = call-poly <vilib>:"Read Key.vi"("section"=w868, "error in (no error)"=w905, "key"="泵滴定数3", "refnum"=w912) -> ("error out"=w917:errorcluster, "value"=w916:dbl, "refnum out"=w913:T6)  [unwired: 4 in, 1 out]
        n553 = local write "泵滴定数3"(w916) -> ()
        n554 = call-poly <vilib>:"Read Key.vi"("section"=w868, "error in (no error)"=w917, "key"="浓度4", "refnum"=w913) -> ("error out"=w918:errorcluster, "value"=w854:dbl, "refnum out"=w914:T6)  [unwired: 4 in, 1 out]
        n555 = local write "浓度4"(w854) -> ()
        n556 = call-poly <vilib>:"Read Key.vi"("section"=w868, "error in (no error)"=w918, "key"="浓度5", "refnum"=w914) -> ("error out"=w859:errorcluster, "value"=w853:dbl, "refnum out"=w860:T6)  [unwired: 4 in, 1 out]
        n557 = local write "浓度5"(w853) -> ()
        n558 = call-poly <vilib>:"Read Key.vi"("section"=w868, "error in (no error)"=w859, "key"="泵滴定数4", "refnum"=w860) -> ("error out"=w919:errorcluster, "value"=w852:dbl, "refnum out"=w915:T6)  [unwired: 4 in, 1 out]
        n559 = local write "泵滴定数4"(w852) -> ()
        n560 = call-poly <vilib>:"Read Key.vi"("section"=w868, "error in (no error)"=w919, "key"="泵滴定数5", "refnum"=w915) -> ("error out"=w857:errorcluster, "value"=w851:dbl, "refnum out"=w858:T6)  [unwired: 4 in, 1 out]
        n561 = local write "泵滴定数5"(w851) -> ()
        n562 = call-poly <vilib>:"Read Key.vi"("section"=w868, "error in (no error)"=w857, "key"="当前选用的校准", "refnum"=w858) -> ("error out"=w889:errorcluster, "refnum out"=w890:T6)  [unwired: 4 in, 2 out]
        n563 = call-poly <vilib>:"Read Key.vi"("section"=w868, "error in (no error)"=w889, "key"="启用1", "refnum"=w890) -> ("error out"=w886:errorcluster, "value"=w875:bool, "refnum out"=w887:T6)  [unwired: 4 in, 1 out]
        n564 = local write "启用1"(w875) -> ()
        n565 = call-poly <vilib>:"Read Key.vi"("section"=w868, "error in (no error)"=w886, "key"="启用2", "refnum"=w887) -> ("error out"=w884:errorcluster, "value"=w874:bool, "refnum out"=w885:T6)  [unwired: 4 in, 1 out]
        n566 = local write "启用2"(w874) -> ()
        n567 = call-poly <vilib>:"Read Key.vi"("section"=w868, "error in (no error)"=w884, "key"="启用3", "refnum"=w885) -> ("error out"=w882:errorcluster, "value"=w873:bool, "refnum out"=w883:T6)  [unwired: 4 in, 1 out]
        n568 = local write "启用3"(w873) -> ()
        n569 = call-poly <vilib>:"Read Key.vi"("section"=w868, "error in (no error)"=w882, "key"="启用4", "refnum"=w883) -> ("error out"=w880:errorcluster, "value"=w850:bool, "refnum out"=w881:T6)  [unwired: 4 in, 1 out]
        n570 = local write "启用4"(w850) -> ()
        n571 = call-poly <vilib>:"Read Key.vi"("section"=w868, "error in (no error)"=w880, "key"="启用5", "refnum"=w881) -> ("error out"=w855:errorcluster, "value"=w849:bool, "refnum out"=w856:T6)  [unwired: 4 in, 1 out]
        n572 = local write "启用5"(w849) -> ()
        n573 = call <vilib>:"Close Config Data.vi"("error in (no error)"=w855, "refnum"=w856) -> ("error out"=w834:errorcluster, "file path"=w835:path)  [unwired: 8 in]
        n574 = Open/Create/Replace File(file path (use dialog)=w835, error in=w834) -> (refnum out=w837:refnum<file>, error out=w836:errorcluster)  [unwired: 4 in, 1 out]
        n575 = Flush File(refnum=w837, error in=w836) -> (refnum out=w838:refnum<file>, error out=w839:errorcluster)
        n576 = Close File(refnum=w838, error in=w839) -> ()  [unwired: 2 out]
      }
      event "选用水样": Value Change {
        (unwired) "浓度6" ("key")
        n577 = event-data() -> ()  [unwired: 1 in, 6 out]
        n578 = local read "量程选择"() -> (w997:enum16{"低量程", "高量程"})
        n579 = property on="窗格" class="Pane"("Origin"=T4 {"Horizontal"=0, "Vertical"=1300} ("原点")) -> ()  [unwired: 2 in, 2 out]
        n580 = case shown="\"葡萄糖\", 默认" "选用水样" {
          tunnel: ["葡萄糖标线" ("section") "草酸钠标线" ("section")] -> w999
          frame "葡萄糖", Default {
          }
          frame "草酸钠" {
          }
        }
        n581 = global read "CODMN外部API.vi" "ping"() -> (w986:bool)
        n582 = case shown="\"高量程\"" w997 {
          tunnel: ["低量程" "高量程"] -> w998
          frame "低量程", Default {
          }
          frame "高量程" {
          }
        }
        n583 = case shown="假" w986 {
          tunnel: [w1052 w1055] -> w985
          frame False {
            n584 = global read "COD内部交互全局.vi" "配置文件ini"() -> (w1054:string)
            n585 = call <vilib>:"Application Directory.vi"() -> ("Application Directory"=w1053:path)
            n586 = Build Path(base path=w1053, name or relative path=w1054) -> (appended path=w1052:path)
          }
          frame True {
            n587 = global read "CODMN外部API.vi" "配置文件 path"() -> (w1055:path)
          }
        }
        n588 = Concatenate Strings(w999, w998) -> (w952:string)
        n589 = call <vilib>:"Open Config Data.vi"("configuration file path"=w985) -> ("error out"=w981:errorcluster, "refnum"=w982:T6)  [unwired: 8 in, 1 out]
        n590 = Bundle By Name(cluster=cluster{"命令":string} {"命令"=""} ("元素"), "命令"="CODMn读取公式" ("名称（未命名）")) -> (w969:cluster{"命令":string})
        n591 = call-poly <vilib>:"Write Key.vi"("section"="标线选择", "error in (no error)"=w981, "value"="选用水样", "key"="选用水样", "refnum"=w982) -> ("error out"=w978:errorcluster, "refnum out"=w979:T6)  [unwired: 4 in, 1 out]
        n592 = call-poly <vilib>:"Read Key.vi"("section"=w952, "error in (no error)"=w978, "key"="浓度1", "refnum"=w979) -> ("error out"=w1022:errorcluster, "value"=w1020:dbl, "refnum out"=w1021:T6)  [unwired: 4 in, 1 out]
        n593 = Enqueue Element(queue=w968, element=w969, error in (no error)=w967) -> ()  [unwired: 1 in, 3 out]
        n594 = local write "浓度1"(w1020) -> ()
        n595 = call-poly <vilib>:"Read Key.vi"("section"=w952, "error in (no error)"=w1022, "key"="浓度2", "refnum"=w1021) -> ("error out"=w1036:errorcluster, "value"=w1023:dbl, "refnum out"=w1035:T6)  [unwired: 4 in, 1 out]
        n596 = local write "浓度2"(w1023) -> ()
        n597 = call-poly <vilib>:"Read Key.vi"("section"=w952, "error in (no error)"=w1036, "key"="浓度3", "refnum"=w1035) -> ("error out"=w1037:errorcluster, "value"=w1025:dbl, "refnum out"=w1034:T6)  [unwired: 4 in, 1 out]
        n598 = local write "浓度3"(w1025) -> ()
        n599 = call-poly <vilib>:"Read Key.vi"("section"=w952, "error in (no error)"=w1037, "key"="泵滴定数1", "refnum"=w1034) -> ("error out"=w1038:errorcluster, "value"=w1027:dbl, "refnum out"=w1033:T6)  [unwired: 4 in, 1 out]
        n600 = local write "泵滴定数1"(w1027) -> ()
        n601 = call-poly <vilib>:"Read Key.vi"("section"=w952, "error in (no error)"=w1038, "key"="泵滴定数2", "refnum"=w1033) -> ("error out"=w1032:errorcluster, "value"=w1030:dbl, "refnum out"=w1039:T6)  [unwired: 4 in, 1 out]
        n602 = local write "泵滴定数2"(w1030) -> ()
        n603 = call-poly <vilib>:"Read Key.vi"("section"=w952, "error in (no error)"=w1032, "key"="泵滴定数3", "refnum"=w1039) -> ("error out"=w1044:errorcluster, "value"=w1043:dbl, "refnum out"=w1040:T6)  [unwired: 4 in, 1 out]
        n604 = local write "泵滴定数3"(w1043) -> ()
        n605 = call-poly <vilib>:"Read Key.vi"("section"=w952, "error in (no error)"=w1044, "key"="浓度4", "refnum"=w1040) -> ("error out"=w1045:errorcluster, "value"=w992:dbl, "refnum out"=w1041:T6)  [unwired: 4 in, 1 out]
        n606 = local write "浓度4"(w992) -> ()
        n607 = call-poly <vilib>:"Read Key.vi"("section"=w952, "error in (no error)"=w1045, "key"="浓度5", "refnum"=w1041) -> ("error out"=w995:errorcluster, "value"=w991:dbl, "refnum out"=w996:T6)  [unwired: 4 in, 1 out]
        n608 = local write "浓度5"(w991) -> ()
        n609 = call-poly <vilib>:"Read Key.vi"("section"=w952, "error in (no error)"=w995, "key"="泵滴定数4", "refnum"=w996) -> ("error out"=w1046:errorcluster, "value"=w990:dbl, "refnum out"=w1042:T6)  [unwired: 4 in, 1 out]
        n610 = local write "泵滴定数4"(w990) -> ()
        n611 = call-poly <vilib>:"Read Key.vi"("section"=w952, "error in (no error)"=w1046, "key"="泵滴定数5", "refnum"=w1042) -> ("error out"=w993:errorcluster, "value"=w989:dbl, "refnum out"=w994:T6)  [unwired: 4 in, 1 out]
        n612 = local write "泵滴定数5"(w989) -> ()
        n613 = call-poly <vilib>:"Read Key.vi"("section"=w952, "error in (no error)"=w993, "key"="当前选用的校准", "refnum"=w994) -> ("error out"=w1016:errorcluster, "refnum out"=w1017:T6)  [unwired: 4 in, 2 out]
        n614 = call-poly <vilib>:"Read Key.vi"("section"=w952, "error in (no error)"=w1016, "key"="启用1", "refnum"=w1017) -> ("error out"=w1013:errorcluster, "value"=w1002:bool, "refnum out"=w1014:T6)  [unwired: 4 in, 1 out]
        n615 = local write "启用1"(w1002) -> ()
        n616 = call-poly <vilib>:"Read Key.vi"("section"=w952, "error in (no error)"=w1013, "key"="启用2", "refnum"=w1014) -> ("error out"=w1011:errorcluster, "value"=w1001:bool, "refnum out"=w1012:T6)  [unwired: 4 in, 1 out]
        n617 = local write "启用2"(w1001) -> ()
        n618 = call-poly <vilib>:"Read Key.vi"("section"=w952, "error in (no error)"=w1011, "key"="启用3", "refnum"=w1012) -> ("error out"=w1009:errorcluster, "value"=w1000:bool, "refnum out"=w1010:T6)  [unwired: 4 in, 1 out]
        n619 = local write "启用3"(w1000) -> ()
        n620 = call-poly <vilib>:"Read Key.vi"("section"=w952, "error in (no error)"=w1009, "key"="启用4", "refnum"=w1010) -> ("error out"=w1007:errorcluster, "value"=w988:bool, "refnum out"=w1008:T6)  [unwired: 4 in, 1 out]
        n621 = local write "启用4"(w988) -> ()
        n622 = call-poly <vilib>:"Read Key.vi"("section"=w952, "error in (no error)"=w1007, "key"="启用5", "refnum"=w1008) -> ("error out"=w949:errorcluster, "value"=w987:bool, "refnum out"=w953:T6)  [unwired: 4 in, 1 out]
        n623 = call-poly <vilib>:"Read Key.vi"("section"=w952, "error in (no error)"=w949, "key"="零点校准时间", "refnum"=w953) -> ("error out"=w965:errorcluster, "value"=w934:string, "refnum out"=w964:T6)  [unwired: 4 in, 1 out]
        n624 = Unflatten From String(type=timestamp(0 s since 1904-01-01), binary string=w934) -> (value=w935:timestamp)  [unwired: 3 in, 2 out]
        n625 = call-poly <vilib>:"Read Key.vi"("section"=w952, "error in (no error)"=w965, "key"="标液1校准时间", "refnum"=w964) -> ("error out"=w960:errorcluster, "value"=w937:string, "refnum out"=w957:T6)  [unwired: 4 in, 1 out]
        n626 = local write "零点校准时间"(w935) -> ()
        n627 = Unflatten From String(type=timestamp(0 s since 1904-01-01), binary string=w937) -> (value=w936:timestamp)  [unwired: 3 in, 2 out]
        n628 = call-poly <vilib>:"Read Key.vi"("section"=w952, "error in (no error)"=w960, "key"="标液2校准时间", "refnum"=w957) -> ("error out"=w961:errorcluster, "value"=w940:string, "refnum out"=w955:T6)  [unwired: 4 in, 1 out]
        n629 = local write "标液校准时间1"(w936) -> ()
        n630 = local write "启用5"(w987) -> ()
        n631 = Unflatten From String(type=timestamp(0 s since 1904-01-01), binary string=w940) -> (value=w939:timestamp)  [unwired: 3 in, 2 out]
        n632 = call-poly <vilib>:"Read Key.vi"("section"=w952, "error in (no error)"=w961, "key"="标液3校准时间", "refnum"=w955) -> ("error out"=w962:errorcluster, "value"=w943:string, "refnum out"=w963:T6)  [unwired: 4 in, 1 out]
        n633 = local write "标液校准时间2"(w939) -> ()
        n634 = Unflatten From String(type=timestamp(0 s since 1904-01-01), binary string=w943) -> (value=w942:timestamp)  [unwired: 3 in, 2 out]
        n635 = call-poly <vilib>:"Read Key.vi"("section"=w952, "error in (no error)"=w962, "key"="标液4校准时间", "refnum"=w963) -> ("error out"=w950:errorcluster, "value"=w946:string, "refnum out"=w951:T6)  [unwired: 4 in, 1 out]
        n636 = call <vilib>:"Close Config Data.vi"("error in (no error)"=w950, "refnum"=w951) -> ("error out"=w972:errorcluster, "file path"=w973:path)  [unwired: 8 in]
        n637 = Open/Create/Replace File(file path (use dialog)=w973, error in=w972) -> (refnum out=w975:refnum<file>, error out=w974:errorcluster)  [unwired: 4 in, 1 out]
        n638 = Flush File(refnum=w975, error in=w974) -> (refnum out=w976:refnum<file>, error out=w977:errorcluster)
        n639 = Close File(refnum=w976, error in=w977) -> ()  [unwired: 2 out]
        n640 = local write "标液校准时间3"(w942) -> ()
        n641 = Unflatten From String(type=timestamp(0 s since 1904-01-01), binary string=w946) -> (value=w945:timestamp)  [unwired: 3 in, 2 out]
        n642 = local write "标液校准时间4"(w945) -> ()
      }
      event "量程选择": Value Change {
        w1109 = "量程选择" ("section")
        n643 = event-data() -> ()  [unwired: 1 in, 6 out]
        n644 = local read "选用水样"() -> (w1124:enum16{"葡萄糖", "草酸钠"})
        n645 = property on="窗格" class="Pane"("Origin"=T4 {"Horizontal"=0, "Vertical"=1300} ("原点")) -> ()  [unwired: 2 in, 2 out]
        n646 = Bundle By Name(cluster=cluster{"命令":string} {"命令"=""} ("元素"), "命令"="CODMn读取公式" ("名称（未命名）")) -> (w1095:cluster{"命令":string})
        n647 = case shown="\"葡萄糖\", 默认" w1124 {
          tunnel: ["葡萄糖标线" ("section") "草酸钠标线" ("section")] -> w1123
          frame "葡萄糖", Default {
          }
          frame "草酸钠" {
          }
        }
        n648 = global read "CODMN外部API.vi" "ping"() -> (w1111:bool)
        n649 = case shown="\"高量程\"" "量程选择" {
          tunnel: ["低量程" "高量程"] -> w1122
          frame "低量程", Default {
          }
          frame "高量程" {
          }
        }
        n650 = Enqueue Element(queue=w1094, element=w1095, error in (no error)=w1093) -> ()  [unwired: 1 in, 3 out]
        n651 = case shown="假" w1111 {
          tunnel: [w1177 w1180] -> w1110
          frame False {
            n652 = global read "COD内部交互全局.vi" "配置文件ini"() -> (w1179:string)
            n653 = call <vilib>:"Application Directory.vi"() -> ("Application Directory"=w1178:path)
            n654 = Build Path(base path=w1178, name or relative path=w1179) -> (appended path=w1177:path)
          }
          frame True {
            n655 = global read "CODMN外部API.vi" "配置文件 path"() -> (w1180:path)
          }
        }
        n656 = Concatenate Strings(w1123, w1122) -> (w1060:string)
        n657 = call <vilib>:"Open Config Data.vi"("configuration file path"=w1110) -> ("error out"=w1108:errorcluster, "refnum"=w1107:T6)  [unwired: 8 in, 1 out]
        n658 = call-poly <vilib>:"Write Key.vi"("section"=w1109, "error in (no error)"=w1108, "value"="量程选择", "key"=w1109, "refnum"=w1107) -> ("error out"=w1104:errorcluster, "refnum out"=w1106:T6)  [unwired: 4 in, 1 out]
        n659 = call-poly <vilib>:"Read Key.vi"("section"=w1060, "error in (no error)"=w1104, "key"="浓度1", "refnum"=w1106) -> ("error out"=w1147:errorcluster, "value"=w1145:dbl, "refnum out"=w1146:T6)  [unwired: 4 in, 1 out]
        n660 = local write "浓度1"(w1145) -> ()
        n661 = call-poly <vilib>:"Read Key.vi"("section"=w1060, "error in (no error)"=w1147, "key"="浓度2", "refnum"=w1146) -> ("error out"=w1161:errorcluster, "value"=w1148:dbl, "refnum out"=w1160:T6)  [unwired: 4 in, 1 out]
        n662 = local write "浓度2"(w1148) -> ()
        n663 = call-poly <vilib>:"Read Key.vi"("section"=w1060, "error in (no error)"=w1161, "key"="浓度3", "refnum"=w1160) -> ("error out"=w1162:errorcluster, "value"=w1150:dbl, "refnum out"=w1159:T6)  [unwired: 4 in, 1 out]
        n664 = local write "浓度3"(w1150) -> ()
        n665 = call-poly <vilib>:"Read Key.vi"("section"=w1060, "error in (no error)"=w1162, "key"="泵滴定数1", "refnum"=w1159) -> ("error out"=w1163:errorcluster, "value"=w1152:dbl, "refnum out"=w1158:T6)  [unwired: 4 in, 1 out]
        n666 = local write "泵滴定数1"(w1152) -> ()
        n667 = call-poly <vilib>:"Read Key.vi"("section"=w1060, "error in (no error)"=w1163, "key"="泵滴定数2", "refnum"=w1158) -> ("error out"=w1157:errorcluster, "value"=w1155:dbl, "refnum out"=w1164:T6)  [unwired: 4 in, 1 out]
        n668 = local write "泵滴定数2"(w1155) -> ()
        n669 = call-poly <vilib>:"Read Key.vi"("section"=w1060, "error in (no error)"=w1157, "key"="泵滴定数3", "refnum"=w1164) -> ("error out"=w1169:errorcluster, "value"=w1168:dbl, "refnum out"=w1165:T6)  [unwired: 4 in, 1 out]
        n670 = local write "泵滴定数3"(w1168) -> ()
        n671 = call-poly <vilib>:"Read Key.vi"("section"=w1060, "error in (no error)"=w1169, "key"="浓度4", "refnum"=w1165) -> ("error out"=w1170:errorcluster, "value"=w1115:dbl, "refnum out"=w1166:T6)  [unwired: 4 in, 1 out]
        n672 = local write "浓度4"(w1115) -> ()
        n673 = call-poly <vilib>:"Read Key.vi"("section"=w1060, "error in (no error)"=w1170, "key"="浓度5", "refnum"=w1166) -> ("error out"=w1120:errorcluster, "value"=w1114:dbl, "refnum out"=w1121:T6)  [unwired: 4 in, 1 out]
        n674 = local write "浓度5"(w1114) -> ()
        n675 = call-poly <vilib>:"Read Key.vi"("section"=w1060, "error in (no error)"=w1120, "key"="泵滴定数4", "refnum"=w1121) -> ("error out"=w1171:errorcluster, "value"=w1113:dbl, "refnum out"=w1167:T6)  [unwired: 4 in, 1 out]
        n676 = local write "泵滴定数4"(w1113) -> ()
        n677 = call-poly <vilib>:"Read Key.vi"("section"=w1060, "error in (no error)"=w1171, "key"="泵滴定数5", "refnum"=w1167) -> ("error out"=w1118:errorcluster, "value"=w1112:dbl, "refnum out"=w1119:T6)  [unwired: 4 in, 1 out]
        n678 = local write "泵滴定数5"(w1112) -> ()
        n679 = call-poly <vilib>:"Read Key.vi"("section"=w1060, "error in (no error)"=w1118, "key"="当前选用的校准", "refnum"=w1119) -> ("error out"=w1141:errorcluster, "refnum out"=w1142:T6)  [unwired: 4 in, 2 out]
        n680 = call-poly <vilib>:"Read Key.vi"("section"=w1060, "error in (no error)"=w1141, "key"="启用1", "refnum"=w1142) -> ("error out"=w1138:errorcluster, "value"=w1127:bool, "refnum out"=w1139:T6)  [unwired: 4 in, 1 out]
        n681 = local write "启用1"(w1127) -> ()
        n682 = call-poly <vilib>:"Read Key.vi"("section"=w1060, "error in (no error)"=w1138, "key"="启用2", "refnum"=w1139) -> ("error out"=w1136:errorcluster, "value"=w1126:bool, "refnum out"=w1137:T6)  [unwired: 4 in, 1 out]
        n683 = local write "启用2"(w1126) -> ()
        n684 = call-poly <vilib>:"Read Key.vi"("section"=w1060, "error in (no error)"=w1136, "key"="启用3", "refnum"=w1137) -> ("error out"=w1134:errorcluster, "value"=w1125:bool, "refnum out"=w1135:T6)  [unwired: 4 in, 1 out]
        n685 = local write "启用3"(w1125) -> ()
        n686 = call-poly <vilib>:"Read Key.vi"("section"=w1060, "error in (no error)"=w1134, "key"="启用4", "refnum"=w1135) -> ("error out"=w1132:errorcluster, "value"=w1117:bool, "refnum out"=w1133:T6)  [unwired: 4 in, 1 out]
        n687 = local write "启用4"(w1117) -> ()
        n688 = call-poly <vilib>:"Read Key.vi"("section"=w1060, "error in (no error)"=w1132, "key"="启用5", "refnum"=w1133) -> ("error out"=w1062:errorcluster, "value"=w1116:bool, "refnum out"=w1061:T6)  [unwired: 4 in, 1 out]
        n689 = call-poly <vilib>:"Read Key.vi"("section"=w1060, "error in (no error)"=w1062, "key"="零点校准时间", "refnum"=w1061) -> ("error out"=w1091:errorcluster, "value"=w1065:string, "refnum out"=w1090:T6)  [unwired: 4 in, 1 out]
        n690 = Unflatten From String(type=timestamp(0 s since 1904-01-01), binary string=w1065) -> (value=w1066:timestamp)  [unwired: 3 in, 2 out]
        n691 = call-poly <vilib>:"Read Key.vi"("section"=w1060, "error in (no error)"=w1091, "key"="标液1校准时间", "refnum"=w1090) -> ("error out"=w1086:errorcluster, "value"=w1068:string, "refnum out"=w1083:T6)  [unwired: 4 in, 1 out]
        n692 = local write "零点校准时间"(w1066) -> ()
        n693 = Unflatten From String(type=timestamp(0 s since 1904-01-01), binary string=w1068) -> (value=w1067:timestamp)  [unwired: 3 in, 2 out]
        n694 = call-poly <vilib>:"Read Key.vi"("section"=w1060, "error in (no error)"=w1086, "key"="标液2校准时间", "refnum"=w1083) -> ("error out"=w1087:errorcluster, "value"=w1071:string, "refnum out"=w1081:T6)  [unwired: 4 in, 1 out]
        n695 = local write "标液校准时间1"(w1067) -> ()
        n696 = local write "启用5"(w1116) -> ()
        n697 = Unflatten From String(type=timestamp(0 s since 1904-01-01), binary string=w1071) -> (value=w1070:timestamp)  [unwired: 3 in, 2 out]
        n698 = call-poly <vilib>:"Read Key.vi"("section"=w1060, "error in (no error)"=w1087, "key"="标液3校准时间", "refnum"=w1081) -> ("error out"=w1088:errorcluster, "value"=w1074:string, "refnum out"=w1089:T6)  [unwired: 4 in, 1 out]
        n699 = local write "标液校准时间2"(w1070) -> ()
        n700 = Unflatten From String(type=timestamp(0 s since 1904-01-01), binary string=w1074) -> (value=w1073:timestamp)  [unwired: 3 in, 2 out]
        n701 = call-poly <vilib>:"Read Key.vi"("section"=w1060, "error in (no error)"=w1088, "key"="标液4校准时间", "refnum"=w1089) -> ("error out"=w1063:errorcluster, "value"=w1077:string, "refnum out"=w1064:T6)  [unwired: 4 in, 1 out]
        n702 = call <vilib>:"Close Config Data.vi"("error in (no error)"=w1063, "refnum"=w1064) -> ("error out"=w1098:errorcluster, "file path"=w1099:path)  [unwired: 8 in]
        n703 = Open/Create/Replace File(file path (use dialog)=w1099, error in=w1098) -> (refnum out=w1101:refnum<file>, error out=w1100:errorcluster)  [unwired: 4 in, 1 out]
        n704 = Flush File(refnum=w1101, error in=w1100) -> (refnum out=w1102:refnum<file>, error out=w1103:errorcluster)
        n705 = Close File(refnum=w1102, error in=w1103) -> ()  [unwired: 2 out]
        n706 = local write "标液校准时间3"(w1073) -> ()
        n707 = Unflatten From String(type=timestamp(0 s since 1904-01-01), binary string=w1077) -> (value=w1076:timestamp)  [unwired: 3 in, 2 out]
        n708 = local write "标液校准时间4"(w1076) -> ()
      }
      event "返回": Value Change {
        w1206 = "CODMn" ("section")
        n709 = event-data() -> ()  [unwired: 1 in, 6 out]
        n710 = property on="窗格" class="Pane"("Origin"=T4 {"Horizontal"=0, "Vertical"=0} ("原点")) -> ()  [unwired: 2 in, 2 out]
        n711 = global read "CODMN外部API.vi" "ping"() -> (w1192:bool)
        n712 = case shown="假" w1192 {
          tunnel: [w1257 w1260] -> w1191
          frame False {
            n713 = global read "COD内部交互全局.vi" "配置文件ini"() -> (w1259:string)
            n714 = call <vilib>:"Application Directory.vi"() -> ("Application Directory"=w1258:path)
            n715 = Build Path(base path=w1258, name or relative path=w1259) -> (appended path=w1257:path)
          }
          frame True {
            n716 = global read "CODMN外部API.vi" "配置文件 path"() -> (w1260:path)
          }
        }
        n717 = call <vilib>:"Open Config Data.vi"("configuration file path"=w1191) -> ("error out"=w1255:errorcluster, "refnum"=w1256:T6)  [unwired: 8 in, 1 out]
        n718 = local read "浓度1"() -> (w1253:dbl)
        n719 = call-poly <vilib>:"Write Key.vi"("section"=w1206, "error in (no error)"=w1255, "value"=w1253, "key"="浓度1", "refnum"=w1256) -> ("error out"=w1252:errorcluster, "refnum out"=w1251:T6)  [unwired: 4 in, 1 out]
        n720 = local read "浓度2"() -> (w1237:dbl)
        n721 = call-poly <vilib>:"Write Key.vi"("section"=w1206, "error in (no error)"=w1252, "value"=w1237, "key"="浓度2", "refnum"=w1251) -> ("error out"=w1250:errorcluster, "refnum out"=w1249:T6)  [unwired: 4 in, 1 out]
        n722 = local read "浓度3"() -> (w1233:dbl)
        n723 = local read "泵滴定数1"() -> (w1231:dbl)
        n724 = call-poly <vilib>:"Write Key.vi"("section"=w1206, "error in (no error)"=w1250, "value"=w1233, "key"="浓度3", "refnum"=w1249) -> ("error out"=w1248:errorcluster, "refnum out"=w1247:T6)  [unwired: 4 in, 1 out]
        n725 = local read "泵滴定数2"() -> (w1229:dbl)
        n726 = call-poly <vilib>:"Write Key.vi"("section"=w1206, "error in (no error)"=w1248, "value"=w1231, "key"="泵滴定数1", "refnum"=w1247) -> ("error out"=w1246:errorcluster, "refnum out"=w1245:T6)  [unwired: 4 in, 1 out]
        n727 = local read "泵滴定数3"() -> (w1227:dbl)
        n728 = call-poly <vilib>:"Write Key.vi"("section"=w1206, "error in (no error)"=w1246, "value"=w1229, "key"="泵滴定数2", "refnum"=w1245) -> ("error out"=w1244:errorcluster, "refnum out"=w1243:T6)  [unwired: 4 in, 1 out]
        n729 = call-poly <vilib>:"Write Key.vi"("section"=w1206, "error in (no error)"=w1244, "value"=w1227, "key"="泵滴定数3", "refnum"=w1243) -> ("error out"=w1242:errorcluster, "refnum out"=w1241:T6)  [unwired: 4 in, 1 out]
        n730 = local read "浓度4"() -> (w1194:dbl)
        n731 = call-poly <vilib>:"Write Key.vi"("section"=w1206, "error in (no error)"=w1242, "value"=w1194, "key"="浓度4", "refnum"=w1241) -> ("error out"=w1235:errorcluster, "refnum out"=w1236:T6)  [unwired: 4 in, 1 out]
        n732 = local read "浓度5"() -> (w1193:dbl)
        n733 = local read "泵滴定数4"() -> (w1195:dbl)
        n734 = call-poly <vilib>:"Write Key.vi"("section"=w1206, "error in (no error)"=w1235, "value"=w1193, "key"="浓度5", "refnum"=w1236) -> ("error out"=w1203:errorcluster, "refnum out"=w1204:T6)  [unwired: 4 in, 1 out]
        n735 = local read "泵滴定数5"() -> (w1196:dbl)
        n736 = call-poly <vilib>:"Write Key.vi"("section"=w1206, "error in (no error)"=w1203, "value"=w1195, "key"="泵滴定数4", "refnum"=w1204) -> ("error out"=w1240:errorcluster, "refnum out"=w1239:T6)  [unwired: 4 in, 1 out]
        n737 = call-poly <vilib>:"Write Key.vi"("section"=w1206, "error in (no error)"=w1240, "value"=w1196, "key"="泵滴定数5", "refnum"=w1239) -> ("error out"=w1201:errorcluster, "refnum out"=w1202:T6)  [unwired: 4 in, 1 out]
        n738 = local read "启用1"() -> (w1215:bool)
        n739 = call-poly <vilib>:"Write Key.vi"("section"=w1206, "error in (no error)"=w1201, "value"=w1215, "key"="启用1", "refnum"=w1202) -> ("error out"=w1211:errorcluster, "refnum out"=w1214:T6)  [unwired: 4 in, 1 out]
        n740 = local read "启用2"() -> (w1212:bool)
        n741 = call-poly <vilib>:"Write Key.vi"("section"=w1206, "error in (no error)"=w1211, "value"=w1212, "key"="启用2", "refnum"=w1214) -> ("error out"=w1222:errorcluster, "refnum out"=w1221:T6)  [unwired: 4 in, 1 out]
        n742 = local read "启用3"() -> (w1210:bool)
        n743 = call-poly <vilib>:"Write Key.vi"("section"=w1206, "error in (no error)"=w1222, "value"=w1210, "key"="启用3", "refnum"=w1221) -> ("error out"=w1220:errorcluster, "refnum out"=w1219:T6)  [unwired: 4 in, 1 out]
        n744 = local read "启用4"() -> (w1198:bool)
        n745 = call-poly <vilib>:"Write Key.vi"("section"=w1206, "error in (no error)"=w1220, "value"=w1198, "key"="启用4", "refnum"=w1219) -> ("error out"=w1218:errorcluster, "refnum out"=w1217:T6)  [unwired: 4 in, 1 out]
        n746 = local read "启用5"() -> (w1197:bool)
        n747 = call-poly <vilib>:"Write Key.vi"("section"=w1206, "error in (no error)"=w1218, "value"=w1197, "key"="启用5", "refnum"=w1217) -> ("error out"=w1199:errorcluster, "refnum out"=w1200:T6)  [unwired: 4 in, 1 out]
        n748 = call <vilib>:"Close Config Data.vi"("error in (no error)"=w1199, "refnum"=w1200) -> ("error out"=w1185:errorcluster, "file path"=w1186:path)  [unwired: 8 in]
        n749 = Open/Create/Replace File(file path (use dialog)=w1186, error in=w1185) -> (refnum out=w1188:refnum<file>, error out=w1187:errorcluster)  [unwired: 4 in, 1 out]
        n750 = Flush File(refnum=w1188, error in=w1187) -> (refnum out=w1189:refnum<file>, error out=w1190:errorcluster)
        n751 = Close File(refnum=w1189, error in=w1190) -> ()  [unwired: 2 out]
      }
      event "关闭", "关闭 2", "关闭 3", "关闭 4": Value Change {
        n752 = event-data() -> ()  [unwired: 1 in, 6 out]
        n753 = property on="窗格" class="Pane"("Origin"=T4 {"Horizontal"=0, "Vertical"=0} ("原点")) -> ()  [unwired: 2 in, 2 out]
      }
      event Application Instance Close {
        n754 = event-data() -> ()  [unwired: 1 in, 4 out]
      }
      event "时间校准": Value Change {
        n755 = event-data() -> ()  [unwired: 1 in, 6 out]
        n756 = Get Date/Time In Seconds() -> (seconds since 1Jan1904=w1270:timestamp)
        n757 = Build Array(w1270) -> (w1269:timestamp[])
        n758 = call "DateToHex.vi"("DATE"=w1269) -> ("数组"=w1267:u16[])  [unwired: 10 in]
        n759 = Insert Into Array(array=u16[] [1] ("values"), index=1 ("索引"), new element=w1267) -> (w1263:u16[])
        n760 = call "CODMnMB_api.vi"("STEP"=enum16{"open", "read", "write", "close"}."write", "values"=w1263, "starting address"=u16 4612) -> ("error out"=w1262:errorcluster)  [unwired: 6 in, 2 out]
        n761 = call <vilib>:"Clear Errors.vi"("error in (no error)"=w1262) -> ()  [unwired: 5 in, 2 out]
      }
      event "故障清除": Value Change {
        n762 = event-data() -> ()  [unwired: 1 in, 6 out]
        n763 = call "CODMnMB_api.vi"("STEP"=enum16{"open", "read", "write", "close"}."write", "values"=u16[] [1], "starting address"=u16 4611) -> ()  [unwired: 6 in, 3 out]
      }
      event "仪器参数": Value Change {
        n764 = event-data() -> ()  [unwired: 1 in, 6 out]
        n765 = global read "CODMn断电保存全局变量.vi" "CODMn仪器参数"() -> (w1274:T12)
        n766 = call "仪器参数设置.vi"("氨氮仪器参数"=w1274) -> ("仪器参数设置输出"=w1275:T18)  [unwired: 10 in]
        n767 = Unbundle By Name(w1275) -> ("确定"=w1276:bool)
        n768 = case shown="真" w1276 {
          tunnel: w1275 -> [_ w1278]
          tunnel: w1274 -> [_ w1277]
          frame False {
          }
          frame True {
            n769 = flat-sequence {
              tunnel: w1278 -> [w1295]
              tunnel: w1277 -> [w1294]
              frame #0 {
                n770 = Unbundle By Name(w1295) -> ("测量量程"=w1293:dbl, "测量精度"=w1292:dbl, "测量间隔"=w1291:dbl, "消解温度"=w1290:dbl, "消解时长"=w1289:dbl, "空白校准时间"=w1288:timestamp, "曲线截距"=w1287:dbl, "曲线斜率"=w1286:dbl, "测量检出限"=w1285:dbl, "测量信号值"=w1284:dbl, "线性相关系数"=w1283:dbl, "二次多项式系数"=w1282:dbl, "标样校准时间"=w1281:timestamp, "稀释倍数"=w1280:dbl)
                n771 = Bundle By Name(cluster=w1294, "测量量程"=w1293, "测量精度"=w1292, "测量间隔"=w1291, "消解温度"=w1290, "消解时长"=w1289, "空白校准时间"=w1288, "曲线截距"=w1287, "曲线斜率"=w1286, "测量检出限"=w1285, "测量信号值"=w1284, "线性相关系数"=w1283, "二次多项式系数"=w1282, "标样校准时间"=w1281, "稀释倍数"=w1280) -> (w1279:T12)
                n772 = global write "CODMn断电保存全局变量.vi" "CODMn仪器参数"(w1279) -> ()
              }
              frame #1 {
                n773 = call "配置文件保存.vi"() -> ()  [unwired: 12 in]
              }
            }
          }
        }
      }
      event "跨度量程选择", "跨度液浓度", "零点核查量程选择", "零点核查浓度", "标样浓度", "标样核查量程选择", "加标回收量程：", "跨度值": Value Change {
        n774 = event-data() -> ()  [unwired: 1 in, 6 out]
        n775 = flat-sequence {
          frame #0 {
            n776 = global write "CODMn断电保存全局变量.vi" "标样浓度"("标样浓度") -> ()
            n777 = global write "CODMn断电保存全局变量.vi" "零点核查浓度"("零点核查浓度") -> ()
            n778 = global write "CODMn断电保存全局变量.vi" "跨度液浓度"("跨度液浓度") -> ()
            n779 = global write "CODMn断电保存全局变量.vi" "CODMn跨度量程选择"("跨度量程选择") -> ()
            n780 = global write "CODMn断电保存全局变量.vi" "加标回收量程选择"("加标回收量程：") -> ()
            n781 = global write "CODMn断电保存全局变量.vi" "跨度值"("跨度值") -> ()
            n782 = global write "CODMn断电保存全局变量.vi" "标样核查量程选择"("标样核查量程选择") -> ()
            n783 = global write "CODMn断电保存全局变量.vi" "零点核查量程选择"("零点核查量程选择") -> ()
          }
          frame #1 {
            n784 = call "配置文件保存.vi"() -> ()  [unwired: 12 in]
          }
        }
      }
      event "校准1", "校准2", "校准3", "校准4", "校准5": Value Change {
        n785 = event-data() -> ()  [unwired: 1 in, 6 out]
        n786 = flat-sequence {
          tunnel: w1307 -> [w1316]
          tunnel: [w1316] -> w1309
          tunnel: w1304 -> [w1315]
          tunnel: [w1315] -> w1306
          tunnel: w1309 -> [w1351]
          tunnel: [w1351] -> w1308
          tunnel: w1306 -> [w1350]
          tunnel: [w1350] -> w1305
          tunnel: w1308 -> [w1378]
          tunnel: w1305 -> [w1377]
          frame #0 {
            n787 = Build Array("校准1", "校准2", "校准3", "校准4", "校准5") -> (w1319:bool[])
            n788 = for {
              tunnel: w1319 -> [w1333] mode=indexing
              tunnel: [w1325] -> w1310
              i -> [w1326]
              n789 = case shown="4" w1326 {
                tunnel: ["浓度1" "浓度2" "浓度3" "浓度4" "浓度5"] -> w1329
                frame 0, Default {
                }
                frame 1 {
                }
                frame 2 {
                }
                frame 3 {
                }
                frame 4 {
                }
              }
              n790 = Multiply(x=w1329, y=100.0) -> (x*y=w1327:dbl)
              n791 = Insert Into Array(array=u16[] [] ("values"), index=0 ("索引"), new element=w1327) -> (w1330:u16[])
              n792 = case shown="真" w1333 {
                tunnel: w1330 -> [_ w1342]
                tunnel: w1326 -> [_ w1344]
                tunnel: [_ w1339] -> w1325
                frame False {
                }
                frame True {
                  n793 = Increment(x=w1344) -> (x+1=w1340:i32)
                  n794 = global write "COD内部交互全局.vi" "当前校准"(w1340) -> ()
                  n795 = call "CODMnMB_api.vi"("STEP"=enum16{"open", "read", "write", "close"}."write", "values"=w1342, "starting address"=u16 4274) -> ("error out"=w1339:errorcluster)  [unwired: 6 in, 2 out]
                }
              }
            }
            n796 = local read "量程选择"() -> (w1312:enum16{"低量程", "高量程"})
            n797 = case shown="\"高量程\"" w1312 {
              tunnel: [u16[] [0] ("values") u16[] [1] ("values")] -> w1311
              frame "低量程", Default {
              }
              frame "高量程" {
              }
            }
            n798 = call "CODMnMB_api.vi"("STEP"=enum16{"open", "read", "write", "close"}."write", "Error in"=w1310, "values"=w1311, "starting address"=u16 4276) -> ()  [unwired: 5 in, 3 out]
          }
          frame #1 {
            n799 = global read "COD内部交互全局.vi" "当前校准"() -> (w1352:i32)
            n800 = case shown="5" w1352 {
              tunnel: [w1360 w1361 w1362 w1363 w1364] -> w1348
              frame 1, Default {
                n801 = local read "浓度1"() -> (w1360:dbl)
              }
              frame 2 {
                n802 = local read "浓度2"() -> (w1361:dbl)
              }
              frame 3 {
                n803 = local read "浓度3"() -> (w1362:dbl)
              }
              frame 4 {
                n804 = local read "浓度4"() -> (w1363:dbl)
              }
              frame 5 {
                n805 = local read "浓度5"() -> (w1364:dbl)
              }
            }
            n806 = Number To Decimal String(number=w1348) -> (decimal integer string=w1347:string)  [unwired: 1 in]
            n807 = Concatenate Strings("仪器校准中!\n当前校准浓度为:", w1347, "mg/L" ("字符串")) -> (w1345:string)
            n808 = Not Equal To 0?(x=w1348) -> (x != 0?=w1356:bool)
            n809 = global write "COD内部交互全局.vi" "校准内容显示"(w1345) -> ()
            n810 = case shown="真" w1356 {
              tunnel: [u16 8 ("address") u16 9 ("address")] -> w1359
              tunnel: ["校零" ("测量模式") "校标" ("测量模式")] -> _
              frame False {
              }
              frame True {
              }
            }
            n811 = Insert Into Array(array=u16[] [] ("values"), index=0 ("索引"), new element=w1359) -> (w1353:u16[])
            n812 = call "CODMnMB_api.vi"("STEP"=enum16{"open", "read", "write", "close"}."write", "values"=w1353, "starting address"=u16 4608 ("address")) -> ()  [unwired: 6 in, 3 out]
          }
          frame #2 {
            n813 = local read "选用水样"() -> (w1386:enum16{"葡萄糖", "草酸钠"})
            n814 = global read "CODMN外部API.vi" "ping"() -> (w1376:bool)
            n815 = case shown="假" w1376 {
              tunnel: [w1394 w1397] -> w1375
              frame False {
                n816 = global read "COD内部交互全局.vi" "配置文件ini"() -> (w1396:string)
                n817 = call <vilib>:"Application Directory.vi"() -> ("Application Directory"=w1395:path)
                n818 = Build Path(base path=w1395, name or relative path=w1396) -> (appended path=w1394:path)
              }
              frame True {
                n819 = global read "CODMN外部API.vi" "配置文件 path"() -> (w1397:path)
              }
            }
            n820 = local read "量程选择"() -> (w1385:enum16{"低量程", "高量程"})
            n821 = case shown="\"葡萄糖\", 默认" w1386 {
              tunnel: ["葡萄糖标线" ("section") "草酸钠标线" ("section")] -> w1387
              frame "葡萄糖", Default {
              }
              frame "草酸钠" {
              }
            }
            n822 = Bundle By Name(cluster=cluster{"命令":string} {"命令"=""} ("元素"), "命令"="CODMn读取参数" ("名称（未命名）")) -> (w1382:cluster{"命令":string})
            n823 = case shown="\"低量程\", 默认" w1385 {
              tunnel: ["低量程" "高量程"] -> w1388
              frame "低量程", Default {
              }
              frame "高量程" {
              }
            }
            n824 = global read "COD内部交互全局.vi" "当前校准"() -> (w1383:i32)
            n825 = Enqueue Element(queue=w1378, element=w1382, timeout in ms (-1)=1000 ("超时毫秒(-1)"), error in (no error)=w1377) -> ()  [unwired: 3 out]
            n826 = Concatenate Strings(w1387, w1388) -> (w1384:string)
            n827 = call <vilib>:"Open Config Data.vi"("configuration file path"=w1375) -> ("error out"=w1392:errorcluster, "refnum"=w1393:T6)  [unwired: 8 in, 1 out]
            n828 = call-poly <vilib>:"Write Key.vi"("section"=w1384, "error in (no error)"=w1392, "value"=w1383, "key"="当前选用的校准" ("section"), "refnum"=w1393) -> ("error out"=w1389:errorcluster, "refnum out"=w1390:T6)  [unwired: 4 in, 1 out]
            n829 = call <vilib>:"Close Config Data.vi"("error in (no error)"=w1389, "refnum"=w1390) -> ("error out"=w1369:errorcluster, "file path"=w1370:path)  [unwired: 8 in]
            n830 = Open/Create/Replace File(file path (use dialog)=w1370, error in=w1369) -> (refnum out=w1372:refnum<file>, error out=w1371:errorcluster)  [unwired: 4 in, 1 out]
            n831 = Flush File(refnum=w1372, error in=w1371) -> (refnum out=w1373:refnum<file>, error out=w1374:errorcluster)
            n832 = Close File(refnum=w1373, error in=w1374) -> ()  [unwired: 2 out]
          }
        }
      }
      event "水样量程选择:", "低切高阈值:", "高切低阈值:": Value Change {
        n833 = event-data() -> ()  [unwired: 1 in, 6 out]
        n834 = flat-sequence {
          frame #0 {
            n835 = global write "CODMn断电保存全局变量.vi" "高切低阈值:"("高切低阈值:") -> ()
            n836 = global write "CODMn断电保存全局变量.vi" "自动切换量程:"("水样量程选择:") -> ()
            n837 = global write "CODMn断电保存全局变量.vi" "低切高阈值:"("低切高阈值:") -> ()
          }
          frame #1 {
            n838 = call "配置文件保存.vi"() -> ()  [unwired: 12 in]
          }
        }
      }
      event "模型": Value Change {
        n839 = event-data() -> ()  [unwired: 1 in, 6 out]
        n840 = global read "CODMN外部API.vi" "ping"() -> (w1412:bool)
        n841 = case shown="假" w1412 {
          tunnel: [w1420 w1423] -> w1411
          frame False {
            n842 = global read "COD内部交互全局.vi" "配置文件ini"() -> (w1422:string)
            n843 = call <vilib>:"Application Directory.vi"() -> ("Application Directory"=w1421:path)
            n844 = Build Path(base path=w1421, name or relative path=w1422) -> (appended path=w1420:path)
          }
          frame True {
            n845 = global read "CODMN外部API.vi" "配置文件 path"() -> (w1423:path)
          }
        }
        n846 = call <vilib>:"Open Config Data.vi"("configuration file path"=w1411) -> ("error out"=w1418:errorcluster, "refnum"=w1419:T6)  [unwired: 8 in, 1 out]
        n847 = local read "模型"() -> (w1413:enum32{"线性", "多项式", "折线"})
        n848 = call-poly <vilib>:"Write Key.vi"("section"="CODMn模型选择" ("key"), "error in (no error)"=w1418, "value"=w1413, "key"="线性和多项式", "refnum"=w1419) -> ("error out"=w1414:errorcluster, "refnum out"=w1415:T6)  [unwired: 4 in, 1 out]
        n849 = call <vilib>:"Close Config Data.vi"("error in (no error)"=w1414, "refnum"=w1415) -> ("error out"=w1405:errorcluster, "file path"=w1406:path)  [unwired: 8 in]
        n850 = Open/Create/Replace File(file path (use dialog)=w1406, error in=w1405) -> (refnum out=w1408:refnum<file>, error out=w1407:errorcluster)  [unwired: 4 in, 1 out]
        n851 = Flush File(refnum=w1408, error in=w1407) -> (refnum out=w1409:refnum<file>, error out=w1410:errorcluster)
        n852 = Close File(refnum=w1409, error in=w1410) -> ()  [unwired: 2 out]
      }
      event "浓度1", "浓度2", "浓度3", "泵滴定数1", "泵滴定数2", "泵滴定数3", "启用1", "启用2", "启用3", "浓度4", "浓度5", "泵滴定数4", "泵滴定数5", "启用4", "启用5", "标液校准时间1", "标液校准时间2", "标液校准时间3", "标液校准时间4", "零点校准时间": Value Change {
        n853 = event-data() -> ()  [unwired: 1 in, 6 out]
        n854 = local read "选用水样"() -> (w1476:enum16{"葡萄糖", "草酸钠"})
        n855 = local read "量程选择"() -> (w1475:enum16{"低量程", "高量程"})
        n856 = case shown="\"葡萄糖\", 默认" w1476 {
          tunnel: ["葡萄糖标线" ("section") "草酸钠标线" ("section")] -> w1480
          frame "葡萄糖", Default {
          }
          frame "草酸钠" {
          }
        }
        n857 = case shown="\"高量程\"" w1475 {
          tunnel: ["低量程" "高量程"] -> w1474
          frame "低量程", Default {
          }
          frame "高量程" {
          }
        }
        n858 = global read "CODMN外部API.vi" "ping"() -> (w1461:bool)
        n859 = case shown="假" w1461 {
          tunnel: [w1558 w1561] -> w1460
          frame False {
            n860 = global read "COD内部交互全局.vi" "配置文件ini"() -> (w1560:string)
            n861 = call <vilib>:"Application Directory.vi"() -> ("Application Directory"=w1559:path)
            n862 = Build Path(base path=w1559, name or relative path=w1560) -> (appended path=w1558:path)
          }
          frame True {
            n863 = global read "CODMN外部API.vi" "配置文件 path"() -> (w1561:path)
          }
        }
        n864 = Concatenate Strings(w1480, w1474) -> (w1438:string)
        n865 = call <vilib>:"Open Config Data.vi"("configuration file path"=w1460) -> ("error out"=w1529:errorcluster, "refnum"=w1530:T6)  [unwired: 8 in, 1 out]
        n866 = local read "模型"() -> (w1425:enum32{"线性", "多项式", "折线"})
        n867 = case shown="\"折线\"" w1425 {
          tunnel: [9999.0 ("泵滴定数5") 9999.0 ("泵滴定数5") w1533] -> w1424
          frame "线性", Default {
          }
          frame "多项式" {
          }
          frame "折线" {
            n868 = local read "泵滴定数5"() -> (w1540:dbl)
            n869 = local read "泵滴定数3"() -> (w1542:dbl)
            n870 = local read "泵滴定数2"() -> (w1543:dbl)
            n871 = local read "泵滴定数4"() -> (w1541:dbl)
            n872 = local read "泵滴定数1"() -> (w1544:dbl)
            n873 = Build Array(w1544, w1543, w1542, w1541, w1540) -> (w1539:dbl[])
            n874 = local read "启用5"() -> (w1545:bool)
            n875 = local read "启用1"() -> (w1549:bool)
            n876 = local read "启用2"() -> (w1548:bool)
            n877 = local read "启用3"() -> (w1547:bool)
            n878 = local read "启用4"() -> (w1546:bool)
            n879 = Build Array(w1549, w1548, w1547, w1546, w1545) -> (w1538:bool[])
            n880 = for {
              tunnel: w1539 -> [w1552] mode=indexing
              tunnel: w1538 -> [w1553] mode=indexing
              shift-right: [w1551] -> w1536
              shift-left: dbl[] [] -> [w1550]
              n881 = case shown="假" w1553 {
                tunnel: w1552 -> [_ w1557]
                tunnel: w1550 -> [w1554 w1556]
                tunnel: [w1554 w1555] -> w1551
                frame False {
                }
                frame True {
                  n882 = Build Array (concatenate)(w1556, w1557) -> (w1555:dbl[])
                }
              }
            }
            n883 = Sort 1D Array(array=w1536) -> (sorted array=w1535:dbl[])
            n884 = Index Array(array=w1535, index=1 ("索引")) -> (element=w1533:dbl)
          }
        }
        n885 = local read "浓度1"() -> (w1527:dbl)
        n886 = call-poly <vilib>:"Write Key.vi"("section"=w1438, "error in (no error)"=w1529, "value"=w1527, "key"="浓度1", "refnum"=w1530) -> ("error out"=w1526:errorcluster, "refnum out"=w1525:T6)  [unwired: 4 in, 1 out]
        n887 = local read "浓度2"() -> (w1511:dbl)
        n888 = call-poly <vilib>:"Write Key.vi"("section"=w1438, "error in (no error)"=w1526, "value"=w1511, "key"="浓度2", "refnum"=w1525) -> ("error out"=w1524:errorcluster, "refnum out"=w1523:T6)  [unwired: 4 in, 1 out]
        n889 = local read "浓度3"() -> (w1507:dbl)
        n890 = local read "泵滴定数1"() -> (w1505:dbl)
        n891 = call-poly <vilib>:"Write Key.vi"("section"=w1438, "error in (no error)"=w1524, "value"=w1507, "key"="浓度3", "refnum"=w1523) -> ("error out"=w1522:errorcluster, "refnum out"=w1521:T6)  [unwired: 4 in, 1 out]
        n892 = local read "泵滴定数2"() -> (w1503:dbl)
        n893 = call-poly <vilib>:"Write Key.vi"("section"=w1438, "error in (no error)"=w1522, "value"=w1505, "key"="泵滴定数1", "refnum"=w1521) -> ("error out"=w1520:errorcluster, "refnum out"=w1519:T6)  [unwired: 4 in, 1 out]
        n894 = local read "泵滴定数3"() -> (w1501:dbl)
        n895 = call-poly <vilib>:"Write Key.vi"("section"=w1438, "error in (no error)"=w1520, "value"=w1503, "key"="泵滴定数2", "refnum"=w1519) -> ("error out"=w1518:errorcluster, "refnum out"=w1517:T6)  [unwired: 4 in, 1 out]
        n896 = call-poly <vilib>:"Write Key.vi"("section"=w1438, "error in (no error)"=w1518, "value"=w1501, "key"="泵滴定数3", "refnum"=w1517) -> ("error out"=w1516:errorcluster, "refnum out"=w1515:T6)  [unwired: 4 in, 1 out]
        n897 = local read "浓度4"() -> (w1473:dbl)
        n898 = local write "公式切换阈值滴定数(0-9999)"(w1424) -> ()
        n899 = call-poly <vilib>:"Write Key.vi"("section"=w1438, "error in (no error)"=w1516, "value"=w1473, "key"="浓度4", "refnum"=w1515) -> ("error out"=w1509:errorcluster, "refnum out"=w1510:T6)  [unwired: 4 in, 1 out]
        n900 = local read "浓度5"() -> (w1472:dbl)
        n901 = local read "泵滴定数4"() -> (w1469:dbl)
        n902 = call-poly <vilib>:"Write Key.vi"("section"=w1438, "error in (no error)"=w1509, "value"=w1472, "key"="浓度5", "refnum"=w1510) -> ("error out"=w1470:errorcluster, "refnum out"=w1471:T6)  [unwired: 4 in, 1 out]
        n903 = local read "泵滴定数5"() -> (w1468:dbl)
        n904 = call-poly <vilib>:"Write Key.vi"("section"=w1438, "error in (no error)"=w1470, "value"=w1469, "key"="泵滴定数4", "refnum"=w1471) -> ("error out"=w1514:errorcluster, "refnum out"=w1513:T6)  [unwired: 4 in, 1 out]
        n905 = local read "零点校准时间"() -> (w1435:timestamp)
        n906 = call-poly <vilib>:"Write Key.vi"("section"=w1438, "error in (no error)"=w1514, "value"=w1468, "key"="泵滴定数5", "refnum"=w1513) -> ("error out"=w1466:errorcluster, "refnum out"=w1467:T6)  [unwired: 4 in, 1 out]
        n907 = local read "启用1"() -> (w1489:bool)
        n908 = local read "标液校准时间1"() -> (w1433:timestamp)
        n909 = Flatten To String(anything=w1435) -> (data string=w1434:string)  [unwired: 3 in, 2 out]
        n910 = call-poly <vilib>:"Write Key.vi"("section"=w1438, "error in (no error)"=w1466, "value"=w1489, "key"="启用1", "refnum"=w1467) -> ("error out"=w1485:errorcluster, "refnum out"=w1488:T6)  [unwired: 4 in, 1 out]
        n911 = Flatten To String(anything=w1433) -> (data string=w1432:string)  [unwired: 3 in, 2 out]
        n912 = local read "启用2"() -> (w1486:bool)
        n913 = local read "标液校准时间2"() -> (w1430:timestamp)
        n914 = call-poly <vilib>:"Write Key.vi"("section"=w1438, "error in (no error)"=w1485, "value"=w1486, "key"="启用2", "refnum"=w1488) -> ("error out"=w1496:errorcluster, "refnum out"=w1495:T6)  [unwired: 4 in, 1 out]
        n915 = Flatten To String(anything=w1430) -> (data string=w1431:string)  [unwired: 3 in, 2 out]
        n916 = local read "启用3"() -> (w1484:bool)
        n917 = local read "标液校准时间3"() -> (w1427:timestamp)
        n918 = call-poly <vilib>:"Write Key.vi"("section"=w1438, "error in (no error)"=w1496, "value"=w1484, "key"="启用3", "refnum"=w1495) -> ("error out"=w1494:errorcluster, "refnum out"=w1493:T6)  [unwired: 4 in, 1 out]
        n919 = local read "启用4"() -> (w1462:bool)
        n920 = Flatten To String(anything=w1427) -> (data string=w1426:string)  [unwired: 3 in, 2 out]
        n921 = call-poly <vilib>:"Write Key.vi"("section"=w1438, "error in (no error)"=w1494, "value"=w1462, "key"="启用4", "refnum"=w1493) -> ("error out"=w1492:errorcluster, "refnum out"=w1491:T6)  [unwired: 4 in, 1 out]
        n922 = local read "标液校准时间4"() -> (w1429:timestamp)
        n923 = local read "启用5"() -> (w1463:bool)
        n924 = Flatten To String(anything=w1429) -> (data string=w1428:string)  [unwired: 3 in, 2 out]
        n925 = local read "选用水样"() -> (w1479:enum16{"葡萄糖", "草酸钠"})
        n926 = call-poly <vilib>:"Write Key.vi"("section"=w1438, "error in (no error)"=w1492, "value"=w1463, "key"="启用5", "refnum"=w1491) -> ("error out"=w1464:errorcluster, "refnum out"=w1465:T6)  [unwired: 4 in, 1 out]
        n927 = call-poly <vilib>:"Write Key.vi"("section"="标线选择", "error in (no error)"=w1464, "value"=w1479, "key"="选用水样", "refnum"=w1465) -> ("error out"=w1444:errorcluster, "refnum out"=w1445:T6)  [unwired: 4 in, 1 out]
        n928 = call-poly <vilib>:"Write Key.vi"("section"=w1438, "error in (no error)"=w1444, "value"=w1434, "key"="零点校准时间", "refnum"=w1445) -> ("error out"=w1452:errorcluster, "refnum out"=w1451:T6)  [unwired: 4 in, 1 out]
        n929 = call-poly <vilib>:"Write Key.vi"("section"=w1438, "error in (no error)"=w1452, "value"=w1432, "key"="标液1校准时间", "refnum"=w1451) -> ("error out"=w1447:errorcluster, "refnum out"=w1440:T6)  [unwired: 4 in, 1 out]
        n930 = call-poly <vilib>:"Write Key.vi"("section"=w1438, "error in (no error)"=w1447, "value"=w1431, "key"="标液2校准时间", "refnum"=w1440) -> ("error out"=w1448:errorcluster, "refnum out"=w1437:T6)  [unwired: 4 in, 1 out]
        n931 = call-poly <vilib>:"Write Key.vi"("section"=w1438, "error in (no error)"=w1448, "value"=w1426, "key"="标液3校准时间", "refnum"=w1437) -> ("error out"=w1449:errorcluster, "refnum out"=w1450:T6)  [unwired: 4 in, 1 out]
        n932 = call-poly <vilib>:"Write Key.vi"("section"=w1438, "error in (no error)"=w1449, "value"=w1428, "key"="标液4校准时间", "refnum"=w1450) -> ("error out"=w1442:errorcluster, "refnum out"=w1443:T6)  [unwired: 4 in, 1 out]
        n933 = call <vilib>:"Close Config Data.vi"("error in (no error)"=w1442, "refnum"=w1443) -> ("error out"=w1454:errorcluster, "file path"=w1455:path)  [unwired: 8 in]
        n934 = Open/Create/Replace File(file path (use dialog)=w1455, error in=w1454) -> (refnum out=w1457:refnum<file>, error out=w1456:errorcluster)  [unwired: 4 in, 1 out]
        n935 = Flush File(refnum=w1457, error in=w1456) -> (refnum out=w1458:refnum<file>, error out=w1459:errorcluster)
        n936 = Close File(refnum=w1458, error in=w1459) -> ()  [unwired: 2 out]
      }
      event "读取": Value Change {
        (unwired) u16 94 ("number of holding registers")
        (unwired) u16 4616 ("starting address")
        n937 = event-data() -> ()  [unwired: 1 in, 6 out]
        n938 = Bundle By Name(cluster=cluster{"命令":string} {"命令"=""} ("元素"), "命令"="CODMn读取公式" ("名称（未命名）")) -> (w1566:cluster{"命令":string})
        n939 = Enqueue Element(queue=w1570, element=w1566, error in (no error)=w1569) -> ()  [unwired: 1 in, 3 out]
      }
      event "写入": Mouse Down {
        n940 = event-data() -> ()  [unwired: 1 in, 8 out]
        n941 = Two Button Dialog(message="即将将左侧拟合公式写入仪器当前量程\n请选择是否写入？" ("消息"), 2:"确定" ("T按钮名称（“确定”）")) -> (T button?=w1571:bool)  [unwired: 1 in]
        n942 = case shown="真" w1571 {
          frame True {
            n943 = local read "量程选择"() -> (w1577:enum16{"低量程", "高量程"})
            n944 = local read "公式切换阈值滴定数(0-9999)"() -> (w1576:u16)
            n945 = Cluster To Array(cluster="方程系数") -> (array=w1580:dbl[])
            "公式系数" <- w1580
            n946 = local read "模型"() -> (w1578:enum32{"线性", "多项式", "折线"})
            n947 = call "公式写入.vi"("公式 2"="方程系数 2", "公式切换阈值滴定数(0-9999)"=w1576, "公式"="方程系数", "量程选择"=w1577, "模型"=w1578) -> ("error out"=w1579:errorcluster)  [unwired: 6 in]
            n948 = Index Array(array=w1580) -> (element #1=w1583:dbl, element #2=w1581:dbl, element #3=w1582:dbl)  [unwired: 3 in]
            n949 = case shown="无错误" w1579 {
              tunnel: ["写入成功！" "写入失败！"] -> w1584
              tunnel: w1581 -> [w1588 _]
              tunnel: w1583 -> [w1589 _]
              tunnel: w1582 -> [w1590 _]
              tunnel: w1577 -> [_ _]
              frame No Error {
                n950 = Number To Fractional String(number=w1588) -> (F-format string=w1592:string)  [unwired: 3 in]
                n951 = Number To Fractional String(number=w1589) -> (F-format string=w1593:string)  [unwired: 3 in]
                n952 = Number To Fractional String(number=w1590) -> (F-format string=w1591:string)  [unwired: 3 in]
                n953 = property on="模型" class="Enum (严格)"() -> ("RingText.Text"=w1585:string)  [unwired: 2 in, 2 out]
                n954 = property on="量程选择" class="Enum (严格)"() -> ("RingText.Text"=w1601:string)  [unwired: 2 in, 2 out]
                n955 = Concatenate Strings("变更后:" ("table输入"), "K:" ("字符串"), w1593, "B:" ("字符串"), w1592, "X^2:" ("字符串"), w1591) -> (w1594:string)
                n956 = Concatenate Strings(w1585, w1601, "公式改变" ("日志信息")) -> (w1595:string)
                n957 = local write "存校准信息"(TRUE ("存校准信息")) -> ()
                n958 = Get Date/Time In Seconds() -> (seconds since 1Jan1904=w1604:timestamp)
                n959 = Bundle(cluster=T17 {"时间标识"=timestamp(0 s since 1904-01-01), "参数"="", "日志信息"="", "流程参数"=""} ("data in"), "时间标识"=w1604, "参数"="CODMn" ("table输入"), "日志信息"=w1595, "流程参数"=w1594) -> (w1587:T17)
                n960 = call "流程日志字段定义.vi"("table输入"="操作日志", "data in"=w1587) -> ("table输出"=w1607:string, "columns"=w1608:string[], "data out"=w1609:T19)  [unwired: 7 in]
                n961 = call "插入数据.vi"("data"=w1609, "columns"=w1608, "database"="database3.mdb", "table"=w1607) -> ()  [unwired: 7 in, 1 out]
              }
              frame Error {
              }
            }
            n962 = One Button Dialog(message=w1584) -> ()  [unwired: 1 in, 1 out]
          }
          frame False {
          }
        }
      }
      event "滴定曲线", "温度曲线": Value Change {
        n963 = event-data() -> ("CtlRef"=w1613:refnum<vi>)  [unwired: 1 in, 5 out]
        n964 = property class="Bool"(reference=w1613) -> ("Label.Text"=w1612:string)  [unwired: 1 in, 2 out]
        n965 = case shown="\"温度曲线\", 默认" w1612 {
          tunnel: [T4 {"Horizontal"=0, "Vertical"=4000} ("原点") T4 {"Horizontal"=0, "Vertical"=3200} ("原点")] -> w1614
          frame "温度曲线", Default {
          }
          frame "滴定曲线" {
          }
        }
        n966 = property on="窗格" class="Pane"("Origin"=w1614) -> ()  [unwired: 2 in, 2 out]
      }
      event "历史波形", "历史波形 2": Value Change {
        n967 = event-data() -> ("CtlRef"=w1618:refnum<vi>)  [unwired: 1 in, 5 out]
        n968 = property class="Bool (严格)"(reference=w1618) -> ("Label.Text"=w1617:string)  [unwired: 1 in, 2 out]
        n969 = case shown="\"历史波形2\"" w1617 {
          frame "历史波形2" {
            n970 = call-poly <vilib>:"Read Waveforms from File.vi"() -> ("error out"=w1619:errorcluster, "first waveform in record"=w1620:waveform(dbl))  [unwired: 6 in, 2 out]
            n971 = case shown="无错误" w1619 {
              tunnel: w1620 -> [w1623 _]
              frame No Error {
                n972 = Unbundle By Name(w1623) -> ("t0"=w1621:timestamp, "Y"=w1622:dbl[])  [unwired: 2 out]
                n973 = global write "COD内部交互全局.vi" "温度波形时间"(w1621) -> ()
                n974 = global write "COD内部交互全局.vi" "时间温度曲线"(w1622) -> ()
                n975 = global write "COD内部交互全局.vi" "时间-温度"(w1622) -> ()
              }
              frame Error {
                n976 = One Button Dialog(message="打开失败" ("消息")) -> ()  [unwired: 1 in, 1 out]
              }
            }
          }
          frame "历史波形", Default {
            n977 = call-poly <vilib>:"Read Waveforms from File.vi"() -> ("error out"=w1625:errorcluster, "first waveform in record"=w1626:waveform(dbl))  [unwired: 6 in, 2 out]
            n978 = case shown="无错误" w1625 {
              tunnel: w1626 -> [w1629 _]
              frame No Error {
                n979 = Unbundle By Name(w1629) -> ("t0"=w1627:timestamp, "Y"=w1628:dbl[])  [unwired: 2 out]
                n980 = global write "COD内部交互全局.vi" "波形时间"(w1627) -> ()
                n981 = global write "COD内部交互全局.vi" "ORP滴定曲线"(w1628) -> ()
                n982 = global write "COD内部交互全局.vi" "滴定数-ORP值"(w1628) -> ()
              }
              frame Error {
                n983 = One Button Dialog(message="打开失败" ("消息")) -> ()  [unwired: 1 in, 1 out]
              }
            }
          }
        }
      }
      event "释放串口": Value Change {
        n984 = event-data() -> ()  [unwired: 1 in, 6 out]
        n985 = Two Button Dialog(message="确认是否释放串口，释放串口将导致通信失败！" ("消息")) -> (T button?=w1631:bool)  [unwired: 2 in]
        n986 = case shown="真" w1631 {
          tunnel: w1634 -> [_ w1636]
          tunnel: w1633 -> [_ w1635]
          frame False {
          }
          frame True {
            n987 = Bundle By Name(cluster=cluster{"命令":string} {"命令"=""} ("元素"), "命令"="停用模块" ("名称（未命名）")) -> (w1637:cluster{"命令":string})
            n988 = Enqueue Element(queue=w1636, element=w1637, error in (no error)=w1635) -> ()  [unwired: 1 in, 3 out]
          }
        }
      }
      event "打开串口": Value Change {
        n989 = event-data() -> ()  [unwired: 1 in, 6 out]
        n990 = flat-sequence {
          tunnel: w1641 -> [w1649]
          tunnel: w1640 -> [w1648]
          frame #0 {
            n991 = global read "CODMn断电保存全局变量.vi" "VISA resource name"() -> (w1652:refnum<visa-resource-name>)
            n992 = global read "CODMn断电保存全局变量.vi" "MB通信方式选择"() -> (w1645:enum16{"串口", "TCP"})
            n993 = global read "CODMn断电保存全局变量.vi" "PORT"() -> (w1643:string)
            n994 = global read "CODMn断电保存全局变量.vi" "IP"() -> (w1644:string)
            n995 = call "串口配置.vi"("PORT"=w1643, "IP"=w1644, "MB通信方式选择"=w1645, "请选择串口:"=w1652) -> ("PORT 2"=w1646:string, "IP 2"=w1647:string, "确认 2"=w1650:bool, "VISA资源名称 2"=w1651:refnum<visa-resource-name>, "MB通信方式选择 2"=w1642:enum16{"串口", "TCP"})  [unwired: 3 in]
            n996 = case shown="真" w1650 {
              tunnel: w1651 -> [_ w1661]
              tunnel: w1649 -> [_ w1657]
              tunnel: w1648 -> [_ w1656]
              tunnel: w1647 -> [_ w1655]
              tunnel: w1646 -> [_ w1654]
              tunnel: w1642 -> [_ w1653]
              frame False {
              }
              frame True {
                n997 = global write "CODMn断电保存全局变量.vi" "IP"(w1655) -> ()
                n998 = global write "CODMn断电保存全局变量.vi" "PORT"(w1654) -> ()
                n999 = global write "CODMn断电保存全局变量.vi" "VISA resource name"(w1661) -> ()
                n1000 = global write "CODMn断电保存全局变量.vi" "MB通信方式选择"(w1653) -> ()
                n1001 = Bundle By Name(cluster=cluster{"命令":string} {"命令"=""} ("元素"), "命令"="启用模块" ("名称（未命名）")) -> (w1658:cluster{"命令":string})
                n1002 = Enqueue Element(queue=w1657, element=w1658, error in (no error)=w1656) -> ()  [unwired: 1 in, 3 out]
              }
            }
          }
          frame #1 {
            n1003 = call "配置文件保存.vi"() -> ()  [unwired: 12 in]
          }
        }
      }
      event "更新程序": Value Change {
        n1004 = event-data() -> ("CtlRef"=w1664:refnum<vi>, "NewVal"=w1665:bool)  [unwired: 1 in, 4 out]
        n1005 = case shown="真" w1665 {
          tunnel: w1664 -> [_ w1674]
          tunnel: w1663 -> [w1667 w1673]
          tunnel: w1662 -> [w1666 w1672]
          frame False {
            n1006 = Bundle By Name(cluster=cluster{"命令":string} {"命令"=""} ("元素"), "命令"="启用模块" ("名称（未命名）")) -> (w1668:cluster{"命令":string})
            n1007 = Enqueue Element(queue=w1667, element=w1668, error in (no error)=w1666) -> ()  [unwired: 1 in, 3 out]
          }
          frame True {
            n1008 = Two Button Dialog(message="警告，非专业人士请勿进行此操作！！！\n请确认是否继续？" ("消息")) -> (T button?=w1676:bool)  [unwired: 2 in]
            n1009 = case shown="真" w1676 {
              tunnel: w1674 -> [w1692 _]
              tunnel: w1673 -> [_ w1700]
              tunnel: w1672 -> [_ w1699]
              tunnel: [errorcluster {"status"=TRUE, "code"=0, "source"=""} ("error out") w1693] -> w1671
              frame False {
                n1010 = property class="Bool (严格)"(reference=w1692, "Value"=FALSE ("释放串口")) -> ()  [unwired: 1 in, 2 out]
              }
              frame True {
                n1011 = Bundle By Name(cluster=cluster{"命令":string} {"命令"=""} ("元素"), "命令"="CODMn程序更新" ("名称（未命名）")) -> (w1703:cluster{"命令":string})
                n1012 = Enqueue Element(queue=w1700, element=w1703, error in (no error)=w1699) -> (queue out=w1698:refnum<queue>, error out=w1697:errorcluster)  [unwired: 1 in, 1 out]
                n1013 = Bundle By Name(cluster=cluster{"命令":string} {"命令"=""} ("元素"), "命令"="停用模块" ("名称（未命名）")) -> (w1694:cluster{"命令":string})
                n1014 = Enqueue Element(queue=w1698, element=w1694, error in (no error)=w1697) -> (error out=w1693:errorcluster)  [unwired: 1 in, 2 out]
              }
            }
            n1015 = case shown="无错误" w1671 {
              frame No Error {
                n1016 = call "文件对话框"("start path"=path "D:/SRC") -> ("selected path"=w1679:path, "cancelled"=w1677:bool)  [unwired: 11 in, 2 out]
                n1017 = case shown="假" w1677 {
                  tunnel: w1679 -> [w1684 _]
                  frame False {
                    n1018 = Path To String(path=w1684) -> (string=w1681:string)
                    n1019 = Format Into String(format string="  - \"%s\"" ("格式字符串"), initial string="\"C:\\Program Files\\Fatek\\WinProladder\\WProlad.exe\"" ("command line"), w1681) -> (resulting string=w1682:string)  [unwired: 1 in, 1 out]
                    n1020 = call <vilib>:"System Exec.vi"("command line"=w1682) -> ("error out"=w1685:errorcluster)  [unwired: 7 in, 3 out]
                    n1021 = case shown="错误" w1685 {
                      tunnel: w1681 -> [_ w1688]
                      frame No Error {
                      }
                      frame Error {
                        n1022 = Format Into String(format string="  - \"%s\"" ("格式字符串"), initial string="\"C:\\Program Files (x86)\\Fatek\\WinProladder\\WProlad.exe\"" ("command line"), w1688) -> (resulting string=w1686:string)  [unwired: 1 in, 1 out]
                        n1023 = call <vilib>:"System Exec.vi"("command line"=w1686) -> ()  [unwired: 7 in, 4 out]
                      }
                    }
                  }
                  frame True {
                  }
                }
              }
              frame Error {
              }
            }
          }
        }
      }
      event "序列号变更": Value Change {
        n1024 = event-data() -> ()  [unwired: 1 in, 6 out]
        n1025 = local read "CODMn序列号"() -> (w1707:string)
        n1026 = call "序列号写入.vi"("序列号:"=w1707) -> ("确认 2"=w1704:bool, "序列号输出"=w1708:string)  [unwired: 9 in]
        n1027 = case shown="真" w1704 {
          tunnel: w1708 -> [_ w1714]
          tunnel: w1706 -> [_ w1710]
          tunnel: w1705 -> [_ w1709]
          frame False {
          }
          frame True {
            n1028 = global write "COD内部交互全局.vi" "序列号:"(w1714) -> ()
            n1029 = Bundle By Name(cluster=cluster{"命令":string} {"命令"=""} ("元素"), "命令"="CODMn序列号写入" ("名称（未命名）")) -> (w1711:cluster{"命令":string})
            n1030 = Enqueue Element(queue=w1710, element=w1711, error in (no error)=w1709) -> ()  [unwired: 1 in, 3 out]
          }
        }
      }
      event Timeout {
        n1031 = event-data() -> ()  [unwired: 1 in, 3 out]
      }
    }
  }
  n1032 = while {
    stop <- FALSE stop-if-true
    # "数字键盘输入"
    n1033 = event shown="[29] \"公式切换阈值滴定数(0-9999)\": 鼠标按下" {
      selector: _ -> [_ _ _ _ _ _ _ _ _ _ _ _ _ _ _ _ _ _ _ _ _ _ _ _ _ _ _ _ _ _ _]
      dyn-events: _ -> [_ _ _ _ _ _ _ _ _ _ _ _ _ _ _ _ _ _ _ _ _ _ _ _ _ _ _ _ _ _ _]
      timeout: _ -> [_ _ _ _ _ _ _ _ _ _ _ _ _ _ _ _ _ _ _ _ _ _ _ _ _ _ _ _ _ _ _]
      event Timeout {
        n1034 = event-data() -> ()  [unwired: 1 in, 3 out]
      }
      event "温度": Mouse Down {
        n1035 = event-data() -> ()  [unwired: 1 in, 8 out]
        n1036 = local read "温度"() -> (w1717:dbl)
        n1037 = call "数字键盘.vi"("OldNumber"=w1717) -> ("NewNumber"=w1716:sgl)
        n1038 = local write "温度"(w1716) -> ()
      }
      event "恒温时间": Mouse Down {
        n1039 = event-data() -> ()  [unwired: 1 in, 8 out]
        n1040 = local read "恒温时间"() -> (w1718:dbl)
        n1041 = call "数字键盘.vi"("OldNumber"=w1718) -> ("NewNumber"=w1719:sgl)
        n1042 = local write "恒温时间"(w1719) -> ()
      }
      event "标准液浓度": Mouse Down {
        n1043 = event-data() -> ()  [unwired: 1 in, 8 out]
        n1044 = local read "标准液浓度"() -> (w1721:dbl)
        n1045 = call "数字键盘.vi"("OldNumber"=w1721) -> ("NewNumber"=w1720:sgl)
        n1046 = local write "标准液浓度"(w1720) -> ()
      }
      event "氢氧化钠：": Mouse Down {
        n1047 = event-data() -> ()  [unwired: 1 in, 8 out]
        n1048 = local read "氢氧化钠："() -> (w1722:dbl)
        n1049 = call "数字键盘.vi"("OldNumber"=w1722) -> ("NewNumber"=w1723:sgl)
        n1050 = local write "氢氧化钠："(w1723) -> ()
      }
      event "水样：": Mouse Down {
        n1051 = event-data() -> ()  [unwired: 1 in, 8 out]
        n1052 = local read "水样："() -> (w1724:dbl)
        n1053 = call "数字键盘.vi"("OldNumber"=w1724) -> ("NewNumber"=w1725:sgl)
        n1054 = local write "水样："(w1725) -> ()
      }
      event "蒸馏水：": Mouse Down {
        n1055 = event-data() -> ()  [unwired: 1 in, 8 out]
        n1056 = local read "蒸馏水："() -> (w1726:dbl)
        n1057 = call "数字键盘.vi"("OldNumber"=w1726) -> ("NewNumber"=w1727:sgl)
        n1058 = local write "蒸馏水："(w1727) -> ()
      }
      event "标液：": Mouse Down {
        n1059 = event-data() -> ()  [unwired: 1 in, 8 out]
        n1060 = local read "标液："() -> (w1728:dbl)
        n1061 = call "数字键盘.vi"("OldNumber"=w1728) -> ("NewNumber"=w1729:sgl)
        n1062 = local write "标液："(w1729) -> ()
      }
      event "零点核查样：": Mouse Down {
        n1063 = event-data() -> ()  [unwired: 1 in, 8 out]
        n1064 = local read "零点核查样："() -> (w1730:dbl)
        n1065 = call "数字键盘.vi"("OldNumber"=w1730) -> ("NewNumber"=w1731:sgl)
        n1066 = local write "零点核查样："(w1731) -> ()
      }
      event "加标回收样：": Mouse Down {
        n1067 = event-data() -> ()  [unwired: 1 in, 8 out]
        n1068 = local read "加标回收样："() -> (w1732:dbl)
        n1069 = call "数字键盘.vi"("OldNumber"=w1732) -> ("NewNumber"=w1733:sgl)
        n1070 = local write "加标回收样："(w1733) -> ()
      }
      event "草酸钠": Mouse Down {
        n1071 = event-data() -> ()  [unwired: 1 in, 8 out]
        n1072 = local read "草酸钠"() -> (w1734:dbl)
        n1073 = call "数字键盘.vi"("OldNumber"=w1734) -> ("NewNumber"=w1735:sgl)
        n1074 = local write "草酸钠"(w1735) -> ()
      }
      event "高锰酸钾": Mouse Down {
        n1075 = event-data() -> ()  [unwired: 1 in, 8 out]
        n1076 = local read "高锰酸钾"() -> (w1736:dbl)
        n1077 = call "数字键盘.vi"("OldNumber"=w1736) -> ("NewNumber"=w1737:sgl)
        n1078 = local write "高锰酸钾"(w1737) -> ()
      }
      event "硫酸": Mouse Down {
        n1079 = event-data() -> ()  [unwired: 1 in, 8 out]
        n1080 = local read "硫酸"() -> (w1738:dbl)
        n1081 = call "数字键盘.vi"("OldNumber"=w1738) -> ("NewNumber"=w1739:sgl)
        n1082 = local write "硫酸"(w1739) -> ()
      }
      event "零点泵计量数 2": Mouse Down {
        n1083 = event-data() -> ()  [unwired: 1 in, 8 out]
        n1084 = local read "零点泵计量数 2"() -> (w1740:dbl)
        n1085 = call "数字键盘.vi"("OldNumber"=w1740) -> ("NewNumber"=w1741:sgl)
        n1086 = local write "零点泵计量数 2"(w1741) -> ()
      }
      event "标度泵计量数 2": Mouse Down {
        n1087 = event-data() -> ()  [unwired: 1 in, 8 out]
        n1088 = local read "标度泵计量数 2"() -> (w1742:dbl)
        n1089 = call "数字键盘.vi"("OldNumber"=w1742) -> ("NewNumber"=w1743:sgl)
        n1090 = local write "标度泵计量数 2"(w1743) -> ()
      }
      event "高量程稀释倍数:": Mouse Down {
        n1091 = event-data() -> ()  [unwired: 1 in, 8 out]
        n1092 = local read "高量程稀释倍数:"() -> (w1745:i8)
        n1093 = call "数字键盘.vi"("OldNumber"=w1745) -> ("NewNumber"=w1744:sgl)
        n1094 = local write "高量程稀释倍数:"(w1744) -> ()
      }
      event "低量程稀释倍数:": Mouse Down {
        n1095 = event-data() -> ()  [unwired: 1 in, 8 out]
        n1096 = local read "低量程稀释倍数:"() -> (w1747:i8)
        n1097 = call "数字键盘.vi"("OldNumber"=w1747) -> ("NewNumber"=w1746:sgl)
        n1098 = local write "低量程稀释倍数:"(w1746) -> ()
      }
      event "浓度1": Mouse Down {
        n1099 = event-data() -> ()  [unwired: 1 in, 8 out]
        n1100 = local read "浓度1"() -> (w1749:dbl)
        n1101 = call "数字键盘.vi"("OldNumber"=w1749) -> ("NewNumber"=w1748:sgl)
        n1102 = property on="浓度1" class="DigNum (严格)"("Val(Sgnl)"=w1748) -> ()  [unwired: 2 in, 2 out]
      }
      event "浓度2": Mouse Down {
        n1103 = event-data() -> ()  [unwired: 1 in, 8 out]
        n1104 = local read "浓度2"() -> (w1751:dbl)
        n1105 = call "数字键盘.vi"("OldNumber"=w1751) -> ("NewNumber"=w1750:sgl)
        n1106 = property on="浓度2" class="DigNum (严格)"("Val(Sgnl)"=w1750) -> ()  [unwired: 2 in, 2 out]
      }
      event "浓度3": Mouse Down {
        n1107 = event-data() -> ()  [unwired: 1 in, 8 out]
        n1108 = local read "浓度3"() -> (w1753:dbl)
        n1109 = call "数字键盘.vi"("OldNumber"=w1753) -> ("NewNumber"=w1752:sgl)
        n1110 = property on="浓度3" class="DigNum (严格)"("Val(Sgnl)"=w1752) -> ()  [unwired: 2 in, 2 out]
      }
      event "浓度4": Mouse Down {
        n1111 = event-data() -> ()  [unwired: 1 in, 8 out]
        n1112 = local read "浓度4"() -> (w1755:dbl)
        n1113 = call "数字键盘.vi"("OldNumber"=w1755) -> ("NewNumber"=w1754:sgl)
        n1114 = property on="浓度4" class="DigNum (严格)"("Val(Sgnl)"=w1754) -> ()  [unwired: 2 in, 2 out]
      }
      event "浓度5": Mouse Down {
        n1115 = event-data() -> ()  [unwired: 1 in, 8 out]
        n1116 = local read "浓度5"() -> (w1757:dbl)
        n1117 = call "数字键盘.vi"("OldNumber"=w1757) -> ("NewNumber"=w1756:sgl)
        n1118 = property on="浓度5" class="DigNum (严格)"("Val(Sgnl)"=w1756) -> ()  [unwired: 2 in, 2 out]
      }
      event "跨度液浓度", "零点核查浓度", "标样浓度": Mouse Down {
        n1119 = event-data() -> ("CtlRef"=w1761:refnum<vi>)  [unwired: 1 in, 7 out]
        n1120 = property class="DigNum (严格)"(reference=w1761) -> (reference out=w1758:refnum<vi>, "Value"=w1760:dbl)  [unwired: 1 in, 1 out]
        n1121 = call "数字键盘.vi"("OldNumber"=w1760) -> ("NewNumber"=w1759:sgl)
        n1122 = property class="DigNum (严格)"(reference=w1758, "Val(Sgnl)"=w1759) -> ()  [unwired: 1 in, 2 out]
      }
      event "泵滴定数1": Mouse Down {
        n1123 = event-data() -> ()  [unwired: 1 in, 8 out]
        n1124 = local read "泵滴定数1"() -> (w1763:dbl)
        n1125 = call "数字键盘.vi"("OldNumber"=w1763) -> ("NewNumber"=w1762:sgl)
        n1126 = property on="泵滴定数1" class="DigNum (严格)"("Val(Sgnl)"=w1762) -> ()  [unwired: 2 in, 2 out]
      }
      event "泵滴定数2": Mouse Down {
        n1127 = event-data() -> ()  [unwired: 1 in, 8 out]
        n1128 = local read "泵滴定数2"() -> (w1765:dbl)
        n1129 = call "数字键盘.vi"("OldNumber"=w1765) -> ("NewNumber"=w1764:sgl)
        n1130 = property on="泵滴定数2" class="DigNum (严格)"("Val(Sgnl)"=w1764) -> ()  [unwired: 2 in, 2 out]
      }
      event "泵滴定数3": Mouse Down {
        n1131 = event-data() -> ()  [unwired: 1 in, 8 out]
        n1132 = local read "泵滴定数3"() -> (w1767:dbl)
        n1133 = call "数字键盘.vi"("OldNumber"=w1767) -> ("NewNumber"=w1766:sgl)
        n1134 = property on="泵滴定数3" class="DigNum (严格)"("Val(Sgnl)"=w1766) -> ()  [unwired: 2 in, 2 out]
      }
      event "泵滴定数4": Mouse Down {
        n1135 = event-data() -> ()  [unwired: 1 in, 8 out]
        n1136 = local read "泵滴定数4"() -> (w1769:dbl)
        n1137 = call "数字键盘.vi"("OldNumber"=w1769) -> ("NewNumber"=w1768:sgl)
        n1138 = property on="泵滴定数4" class="DigNum (严格)"("Val(Sgnl)"=w1768) -> ()  [unwired: 2 in, 2 out]
      }
      event "泵滴定数5": Mouse Down {
        n1139 = event-data() -> ()  [unwired: 1 in, 8 out]
        n1140 = local read "泵滴定数5"() -> (w1771:dbl)
        n1141 = call "数字键盘.vi"("OldNumber"=w1771) -> ("NewNumber"=w1770:sgl)
        n1142 = property on="泵滴定数5" class="DigNum (严格)"("Val(Sgnl)"=w1770) -> ()  [unwired: 2 in, 2 out]
      }
      event "低切高阈值:", "高切低阈值:": Mouse Down {
        n1143 = event-data() -> ("CtlRef"=w1775:refnum<vi>)  [unwired: 1 in, 7 out]
        n1144 = property class="DigNum (严格)"(reference=w1775) -> (reference out=w1774:refnum<vi>, "Value"=w1773:dbl)  [unwired: 1 in, 1 out]
        n1145 = call "数字键盘.vi"("OldNumber"=w1773) -> ("NewNumber"=w1772:sgl)
        n1146 = property class="DigNum (严格)"(reference=w1774, "Val(Sgnl)"=w1772) -> ()  [unwired: 1 in, 2 out]
      }
      event "公式切换阈值滴定数(0-9999)": Mouse Down {
        n1147 = event-data() -> ("CtlRef"=w1776:refnum<vi>)  [unwired: 1 in, 7 out]
        n1148 = property class="DigNum (严格)"(reference=w1776) -> (reference out=w1779:refnum<vi>, "Value"=w1778:u16)  [unwired: 1 in, 1 out]
        n1149 = call "数字键盘.vi"("OldNumber"=w1778) -> ("NewNumber"=w1777:sgl)
        n1150 = property class="DigNum (严格)"(reference=w1779, "Value"=w1777) -> ()  [unwired: 1 in, 2 out]
      }
      event "远程校准量程", "远程标样校准": Value Change {
        n1151 = event-data() -> ()  [unwired: 1 in, 6 out]
        n1152 = flat-sequence {
          frame #0 {
            n1153 = global write "CODMn断电保存全局变量.vi" "远程校准量程"("远程校准量程") -> ()
            n1154 = global write "CODMn断电保存全局变量.vi" "远程标样校准"("远程标样校准") -> ()
          }
          frame #1 {
            n1155 = call "配置文件保存.vi"() -> ()  [unwired: 12 in]
          }
        }
      }
    }
  }
  n1156 = while {
    stop <- FALSE stop-if-true
    # "滚动显示"
    n1157 = global read "COD内部交互全局.vi" "待机"() -> (w1782:bool)
    n1158 = case shown="假" w1782 {
      frame False {
        # "运行中"
        n1159 = global read "COD内部交互全局.vi" "校准内容显示"() -> (w1785:string)
        n1160 = while {
          shift-right: [w1787] -> _
          shift-left: w1785 -> [w1792]
          stop <- w1786 stop-if-true
          (unwired) "仪器校准中!\n当前校准浓度为:3mg/L" ("校准内容显示")
          n1161 = Wait (ms)(milliseconds to wait=u32 500 ("等待时间（毫秒）")) -> ()  [unwired: 1 out]
          n1162 = Spreadsheet String To Array(delimiter (Tab)="\n" ("分隔符(Tab)"), format string="" ("格式字符串"), spreadsheet string=w1792, array type (2D Dbl)=string[] []) -> (array=w1795:string[])
          n1163 = for {
            tunnel: w1795 -> [w1803] mode=indexing
            tunnel: [w1801] -> _ mode=indexing
            shift-right: [w1799] -> w1790
            shift-left: "" ("格式字符串") -> [w1800]
            n1164 = call "字符串移位显示.vi"("字符框大小"=36, "字符串输入"=w1803) -> ("移位后字符串"=w1801:string)  [unwired: 8 in, 1 out]
            n1165 = Concatenate Strings(w1800, w1801, "\n" ("分隔符(Tab)")) -> (w1799:string)
          }
          n1166 = String Length(string=w1790) -> (length=w1789:i32)
          n1167 = Decrement(x=w1789) -> (x-1=w1788:i32)
          n1168 = String Subset(string=w1790, length (rest)=w1788) -> (substring=w1787:string)  [unwired: 1 in]
          "校准内容显示" <- w1787
          n1169 = global read "COD内部交互全局.vi" "待机"() -> (w1786:bool)
        }
      }
      frame True {
      }
    }
    n1170 = Wait (ms)(milliseconds to wait=u32 1000 ("等待时间（毫秒）")) -> ()  [unwired: 1 out]
  }
  n1171 = property class="VI"(reference=w6, error in=w3) -> ("Name"=w7:string)  [unwired: 2 out]
  n1172 = while {
    stop <- FALSE stop-if-true
    # "相差60秒自动校时"
    n1173 = global read "运行时序全局变量.vi" "多列列表框"() -> (w1805:i32)
    n1174 = local read "仪器时间"() -> (w1812:timestamp)
    n1175 = local read "系统时间"() -> (w1813:timestamp)
    n1176 = Wait (ms)(milliseconds to wait=u32 1000 ("等待时间（毫秒）")) -> ()  [unwired: 1 out]
    n1177 = Build Array(w1812) -> (w1811:timestamp[])
    n1178 = Build Array(w1813) -> (w1830:timestamp[])
    n1179 = Equal?(x=w1805, y=u16 5) -> (x = y?=w1807:bool)
    n1180 = call <vilib>:"Boolean Crossing PtByPt.vi"("direction"=enum16{"either", "false-true", "true-false"}."false-true", "input"=w1807) -> ("crossing"=w1804:bool)  [unwired: 1 in]
    n1181 = call "DateToHex.vi"("DATE"=w1811) -> ("数组"=w1824:u16[])  [unwired: 10 in]
    n1182 = call "DateToHex.vi"("DATE"=w1830) -> ("数组"=w1829:u16[])  [unwired: 10 in]
    n1183 = case shown="真" w1804 {
      frame False {
      }
      frame True {
        # "校准结束后自动更新曲线泵滴定数"
        n1184 = global read "COD测量模式全局.vi" "测量模式文字实时"() -> (w1831:string)
        n1185 = global read "COD测量模式全局.vi" "测量模式文字实时"() -> (w1836:string)
        n1186 = global read "CODMN外部API.vi" "远程反控校准CODMn"() -> (w1835:bool)
        n1187 = global read "COD内部交互全局.vi" "高锰酸钾"() -> (w1839:dbl)
        n1188 = Equal?(x=w1831, y="校零") -> (x = y?=w1832:bool)
        n1189 = Equal?(x=w1836, y="校标") -> (x = y?=w1838:bool)
        n1190 = Or(x=w1832, y=w1838) -> (x .or. y?=w1834:bool)
        n1191 = case shown="真" w1834 {
          tunnel: w1839 -> [_ w1844]
          tunnel: w1831 -> [_ w1843]
          frame False {
          }
          frame True {
            w1852 = "量程选择" ("section")
            n1192 = global read "COD内部交互全局.vi" "数据存储时间戳"() -> (w1841:timestamp)
            n1193 = global read "CODMN外部API.vi" "ping"() -> (w1863:bool)
            n1194 = case shown="\"校零\"" w1843 {
              tunnel: ["标样校准时间：" "空白校准时间："] -> _
              frame "校标", Default {
              }
              frame "校零" {
              }
            }
            n1195 = case shown="假" w1863 {
              tunnel: [w1872 w1875] -> w1864
              frame False {
                n1196 = global read "COD内部交互全局.vi" "配置文件ini"() -> (w1874:string)
                n1197 = call <vilib>:"Application Directory.vi"() -> ("Application Directory"=w1873:path)
                n1198 = Build Path(base path=w1873, name or relative path=w1874) -> (appended path=w1872:path)
              }
              frame True {
                n1199 = global read "CODMN外部API.vi" "配置文件 path"() -> (w1875:path)
              }
            }
            n1200 = Format Date/Time String(time format string (%c)="%Y/%m/%d %H:%M:%S" ("时间格式字符串(%c)"), seconds (now)=w1841) -> ()  [unwired: 1 in, 1 out]
            n1201 = call <vilib>:"Open Config Data.vi"("configuration file path"=w1864) -> ("error out"=w1851:errorcluster, "refnum"=w1850:T6)  [unwired: 8 in, 1 out]
            n1202 = call-poly <vilib>:"Read Key.vi"("section"="标线选择", "error in (no error)"=w1851, "key"="选用水样", "refnum"=w1850) -> ("error out"=w1853:errorcluster, "value"=w1846:i32, "refnum out"=w1854:T6)  [unwired: 4 in, 1 out]
            n1203 = local write "选用水样"(w1846) -> ()
            n1204 = call-poly <vilib>:"Read Key.vi"("section"=w1852, "error in (no error)"=w1853, "key"=w1852, "refnum"=w1854) -> ("error out"=w1847:errorcluster, "value"=w1849:i32, "refnum out"=w1848:T6)  [unwired: 4 in, 1 out]
            n1205 = case shown="1" w1846 {
              tunnel: ["葡萄糖标线" ("section") "草酸钠标线" ("section")] -> w1861
              frame 0, Default {
              }
              frame 1 {
              }
            }
            n1206 = local write "量程选择"(w1849) -> ()
            n1207 = case shown="2" w1849 {
              tunnel: ["低量程" "高量程" "0-2量程"] -> w1860
              frame 0, Default {
              }
              frame 1 {
              }
              frame 2 {
              }
            }
            n1208 = Concatenate Strings(w1861, w1860) -> (w1862:string)
            n1209 = call-poly <vilib>:"Read Key.vi"("section"=w1862, "error in (no error)"=w1847, "key"="当前选用的校准" ("section"), "refnum"=w1848) -> ("error out"=w1859:errorcluster, "value"=w1842:i32, "refnum out"=w1858:T6)  [unwired: 4 in, 1 out]
            n1210 = case shown="5" w1842 {
              tunnel: w1841 -> [w1865 w1866 w1867 w1868 w1869]
              frame 1, Default {
                "零点校准时间" <- w1865
              }
              frame 2 {
                "标液校准时间1" <- w1866
              }
              frame 3 {
                "标液校准时间2" <- w1867
              }
              frame 4 {
                "标液校准时间3" <- w1868
              }
              frame 5 {
                "标液校准时间4" <- w1869
              }
            }
            n1211 = call <vilib>:"Close Config Data.vi"("error in (no error)"=w1859, "refnum"=w1858) -> ()  [unwired: 8 in, 2 out]
            n1212 = global write "COD内部交互全局.vi" "当前校准"(w1842) -> ()
            n1213 = case shown="5" w1842 {
              tunnel: w1844 -> [w1881 w1882 w1883 w1884 w1885]
              frame 1, Default {
                n1214 = property on="泵滴定数1" class="DigNum (严格)"("Val(Sgnl)"=w1881) -> ()  [unwired: 2 in, 2 out]
              }
              frame 2 {
                n1215 = property on="泵滴定数2" class="DigNum (严格)"("Val(Sgnl)"=w1882) -> ()  [unwired: 2 in, 2 out]
              }
              frame 3 {
                n1216 = property on="泵滴定数3" class="DigNum (严格)"("Val(Sgnl)"=w1883) -> ()  [unwired: 2 in, 2 out]
              }
              frame 4 {
                n1217 = property on="泵滴定数4" class="DigNum (严格)"("Val(Sgnl)"=w1884) -> ()  [unwired: 2 in, 2 out]
              }
              frame 5 {
                n1218 = property on="泵滴定数5" class="DigNum (严格)"("Val(Sgnl)"=w1885) -> ()  [unwired: 2 in, 2 out]
              }
            }
          }
        }
        n1219 = case shown="真" w1835 {
          frame False {
          }
          frame True {
            # "校准完自动写入公式"
            n1220 = global write "CODMN外部API.vi" "远程反控校准CODMn"(FALSE ("远程反控校准CODMn")) -> ()
          }
        }
      }
    }
    n1221 = Index Array(array=w1824, index=2 ("索引")) -> (element=w1826:u16)
    n1222 = Index Array(array=w1829, index=2 ("索引")) -> (element=w1827:u16)
    n1223 = Split Number(x=w1826) -> (hi(x)=w1820:u8)  [unwired: 1 out]
    n1224 = Split Number(x=w1827) -> (hi(x)=w1823:u8)  [unwired: 1 out]
    n1225 = To Byte Integer(number=w1820) -> (8bit integer=w1819:i8)
    n1226 = To Byte Integer(number=w1823) -> (8bit integer=w1822:i8)
    n1227 = Subtract(x=w1819, y=w1822) -> (x-y=w1821:i8)
    n1228 = Absolute Value(x=w1821) -> (abs(x)=w1818:i8)
    n1229 = local read "通讯状态"() -> (w1815:bool)
    n1230 = Greater Or Equal?(x=w1818, y=i8 5) -> (x >= y?=w1816:bool)
    n1231 = And(x=w1816, y=w1815) -> (x .and. y?=w1814:bool)
    n1232 = case shown="真" w1814 {
      frame False {
      }
      frame True {
        # "相差60秒时间自动校准"
        n1233 = flat-sequence {
          frame #0 {
            n1234 = property on="时间校准" class="Bool (严格)"("Val(Sgnl)"=TRUE ("值(信号)")) -> ()  [unwired: 2 in, 2 out]
          }
          frame #1 {
            n1235 = Wait (ms)(milliseconds to wait=u32 500 ("等待时间（毫秒）")) -> ()  [unwired: 1 out]
          }
          frame #2 {
            n1236 = property on="时间校准" class="Bool (严格)"("Val(Sgnl)"=FALSE ("值(信号)")) -> ()  [unwired: 2 in, 2 out]
          }
        }
      }
    }
  }
  n1237 = Open VI Reference(type specifier VI Refnum (for type only)=refnum<vi> refnum, vi path=w7, options=128 ("选项")) -> (vi reference=w9:refnum<vi>, error out=w11:errorcluster)  [unwired: 3 in]
  n1238 = call-by-ref "?"(reference=w9, error in=w11) -> (reference out=w13:refnum<vi>, error out=w12:errorcluster)  [unwired: 12 in]
  n1239 = Close Reference(reference=w13, error in (no error)=w12) -> ()  [unwired: 1 out]
  n1240 = while {
    stop <- FALSE stop-if-true
    n1241 = Wait (ms)(milliseconds to wait=u32 1000 ("等待时间（毫秒）")) -> ()  [unwired: 1 out]
    n1242 = case shown="真" "存校准信息" {
      frame False {
      }
      frame True {
        n1243 = local read "公式系数"() -> (w1894:dbl[])
        n1244 = local read "泵滴定数2"() -> (w1916:dbl)
        n1245 = local read "泵滴定数4"() -> (w1914:dbl)
        n1246 = local read "泵滴定数3"() -> (w1915:dbl)
        n1247 = local read "泵滴定数5"() -> (w1913:dbl)
        n1248 = local read "泵滴定数1"() -> (w1917:dbl)
        n1249 = local read "浓度1"() -> (w1923:dbl)
        n1250 = local read "浓度2"() -> (w1919:dbl)
        n1251 = local read "浓度3"() -> (w1920:dbl)
        n1252 = local read "浓度4"() -> (w1921:dbl)
        n1253 = local read "浓度5"() -> (w1922:dbl)
        n1254 = local read "标液校准时间1"() -> (w1902:timestamp)
        n1255 = local read "标液校准时间2"() -> (w1901:timestamp)
        n1256 = local read "标液校准时间3"() -> (w1900:timestamp)
        n1257 = local read "零点校准时间"() -> (w1903:timestamp)
        n1258 = local read "标液校准时间4"() -> (w1899:timestamp)
        n1259 = Build Array(w1917, w1916, w1915, w1914, w1913) -> (w1912:dbl[])
        n1260 = Build Array(w1923, w1919, w1920, w1921, w1922) -> (w1918:dbl[])
        n1261 = local write "存校准信息"(FALSE ("存校准信息")) -> ()
        n1262 = for {
          tunnel: w1894 -> [w1926] mode=indexing
          tunnel: [w1925] -> w1893 mode=indexing
          n1263 = Number To Fractional String(number=w1926, precision (6)=i16 6 ("宽度(-)")) -> (F-format string=w1925:string)  [unwired: 2 in]
        }
        n1264 = for {
          tunnel: w1918 -> [w1935] mode=indexing
          tunnel: w1912 -> [w1932] mode=indexing
          tunnel: [w1931] -> w1906 mode=indexing
          tunnel: [w1930] -> w1905 mode=indexing
          n1265 = Number To Decimal String(number=w1935, width (-)=i16 0 ("宽度(-)")) -> (decimal integer string=w1931:string)
          n1266 = Number To Decimal String(number=w1932, width (-)=i16 0 ("宽度(-)")) -> (decimal integer string=w1930:string)
        }
        n1267 = Build Array(w1903, w1902, w1901, w1900, w1899) -> (w1898:timestamp[])
        n1268 = local read "启用3"() -> (w1909:bool)
        n1269 = local read "启用5"() -> (w1907:bool)
        n1270 = local read "启用4"() -> (w1908:bool)
        n1271 = local read "启用2"() -> (w1910:bool)
        n1272 = local read "启用1"() -> (w1911:bool)
        n1273 = for {
          tunnel: w1898 -> [w1928] mode=indexing
          tunnel: [w1927] -> w1897 mode=indexing
          n1274 = Format Date/Time String(time format string (%c)="%Y/%m/%d %H:%M:%S" ("时间格式字符串(%c)"), seconds (now)=w1928) -> (date/time string=w1927:string)  [unwired: 1 in]
        }
        n1275 = Build Array(w1911, w1910, w1909, w1908, w1907) -> (w1904:bool[])
        n1276 = local read "量程选择"() -> (w1896:enum16{"低量程", "高量程"})
        n1277 = Array To Cluster(array=w1893) -> (cluster=w1892:T20)
        n1278 = call "生成校准信息.vi"("量程选择"=w1896, "公式系数"=w1892, "启用"=w1904, "校准时间"=w1897, "信号值"=w1905, "校准浓度"=w1906) -> ()  [unwired: 6 in]
      }
    }
  }
